vi "Position_TOTAL_R26.vi"(5 "Distance Between \nCameras  (*unit)":sgl=2.25) -> (12 "dX, dY\nLeft Cam":cluster{"X":sgl[], "Y":sgl[]}={"X"=[-1.0065897, 0.099401906, 1.1628555, 2.2500029, 0.0], "Y"=[10.716516, 10.801518, 10.883252, 10.9668045, 0.0]}, 13 "Position Valid":bool=TRUE, 14 "Left Camera Real Coordinates":cluster{"X":sgl, "Y":sgl}={"X"=10.842023, "Y"=1.3735824}, 16 "dX, dY\nRight Cam":cluster{"X":sgl[], "Y":sgl[]}={"X"=[-2.8840373, -1.7780458, -0.7145921, 0.3725553, -1.8774476], "Y"=[9.387911, 9.472914, 9.554648, 9.638201, -1.3286046]}, 18 "Robot Coordinates":cluster{"X":sgl, "Y":sgl}={"X"=10.17772, "Y"=2.3123062}, 19 "Orietnation\n(current)":sgl=-30.94054 format="%#_13g")   [LabVIEW 2015]
uses:
  <vilib>/Analysis/NI_AALPro.lvlib
  <vilib>/myRIO/Instrument Drivers/Onboard IO/DIO/DIO.lvlib
  <vilib>/Instr/_visa.llb/VISA Configure Serial Port (Instr).vi
  <vilib>/Analysis/coordinate.llb/2D Cartesian Coordinate Rotation (Array).vi
panel:
  out "Current Template - Right":T1(ring)
  out "Current Template - Left":T1(ring)
  in  "Tab Control 2":T2(tab)
  out "Beacon Coordinates - Right Image":T3={"Beacon Position - X px"=[88.975365, 121.85722, 157.60713, 192.74931, 229.82234], "Beacon Position - Y px"=[106.21975, 102.49595, 103.61968, 103.22959, 103.920715]}
  out "Beacon Coordinates - Left Image":T3={"Beacon Position - X px"=[96.57839, 127.0317, 159.93825, 190.94315, 221.86247], "Beacon Position - Y px"=[111.67795, 107.306076, 106.92789, 105.73433, 104.09002]}
  in  "Image Width (px)":sgl=320.0
  in  "Image Height (px)":sgl=240.0
  in  "Cam AOV Horizontal (deg)":sgl=58.0
  in  "Cam AOV Vertical (deg)":sgl=45.0
  out "Angle to Pixel Ratios":T4={"Angle to Pixel\nRatio - Horizontal"=0.18125, "Angle to Pixel\nRatio - Vertical"=0.1875} {"Angle to Pixel\nRatio - Vertical" format="%#_13g"; "Angle to Pixel\nRatio - Horizontal" format="%#_13g"}
  in  "Num of Beacons (Total)":i8=5
  out "Left Data\nInput Flag\n- Internal":bool
  out "Right Data\nInput Flag\n- Internal":bool
  out "This Servo \nAngle - Left":sgl=52.96875
  in  "Valid Angles - L":bool[](array[boolean])=[TRUE, TRUE, TRUE, TRUE, TRUE]
  in  "Valid Angles -R":bool[](array[boolean])=[TRUE, TRUE, TRUE, TRUE, TRUE]
  in  "Beacon Angles - L":sgl[](array[numeric])=[64.19745, 58.642975, 52.682835, 47.05908, 41.446476]
  in  "Beacon Angles -R":sgl[](array[numeric])=[71.43643, 65.46979, 58.9926, 52.62266, 45.904842]
  out "This Servo \nAngle - Right":sgl=58.76953
  in  "Position Calc\nReady":bool=TRUE
  out "Array":sgl[](array[numeric])=[9.555056, 8.575206, 8.036942, 7.810829, 6.6351933]
  out "Array 2":sgl[](array[numeric])=[5.5039287, 6.210328, 7.1312, 8.266513, 8.73579]
  out "Array 3":sgl[](array[numeric])=[3.2039287, 3.9103284, 4.8311996, 5.9665127, 6.4357905]
  in  "stop":bool
  in  "Startup GP's - RIGHT":u16[](array[numeric])
  in  "Startup GP's - LEFT":u16[](array[numeric])
  in  "Servo Algorithm\nCycle Time(ms)":i32=25
  in  "Move Servo\nThreshold (deg)":sgl=2.0 format="%#_13g"
  in  "SERVO ENABLE":bool=TRUE
  in  "Max Write\nTx Attempts":u8=3
  in  "Max Read\nTx Attempts":u8=3
  in  "close comms":bool
  in  "Servo Comm\nLoop Time (ms)":i32=20
  out "dT - Comm Loop":u32=21
  in  "Left Servo\nID":string="\u0000"
  in  "Servo Comm\nWait Time - (ms)":i32
  in  "Right Servo\nID":string="\u0001"
  in  "Search Step Size\n(deg)":sgl=15.0 format="%#_13g"
  out "Last Orientation":sgl=-35.285717
  out "Last Position":cluster{"X":sgl, "Y":sgl}={"X"=10.147585, "Y"=2.64441}
  in  "Compliance Slope":u8=128
  in  "Search Step Size":u16=50
  in  "Mounting Offset - Left":sgl=-45.0
  in  "Minimum Delta \nServo Threshold":i16=3
  in  "Maximum Move \nServo Threshold":i16=300
  in  "Wait Tick Threshold":i32=10
  in  "Min Num Frames\nper Search":i32=3
  in  "Middle Beacon\nCoordinates":cluster{"X":sgl, "Y":sgl}={"X"=0.0, "Y"=2.5}
  in  "Max Recovery\nSearch Attempts":u16=3
  in  "Max Recovery Count\n(Recovery Search)":u16=20
  in  "Mounting Offset - Right":sgl=45.0
  in  "Tracking Timeout\nThreshold":i32=10
  in  "Timeout to \nEnable Reactive Predict":u16=5
  out "Beacon Scales - Right":sgl[](array[numeric])=[50.81787, 54.150085, 54.01553, 51.723366, 54.605507]
  out "Beacon Scales - Left":sgl[](array[numeric])=[46.59789, 48.180458, 47.842606, 46.504417, 45.297752]
  in  "Recovery Parallel\nSearch Offset":u16=50
  in  "Max # Pan Moves":u16=3
  in  "Current Angle\n - Right (internal)":sgl=58.76953
  in  "Current Angle\n - Left (internal)":sgl=52.96875
  in  "Servo Goal Position\n - Left":u16=232
  in  "Servo Goal Position\n - Right":u16=563
  out "Move Servo - R":bool
  out "Move Servo - L":bool
  out "Current L (10bit)":u16=232
  out "Servo Moving - L":bool
  out "Servo Moving - R":bool
  out "Current R (10bit)":u16=559
  out "deltaMoveServo\n- L":i16
  out "Move Respond - L":bool
  out "Move Respond - R":bool
  out "deltaMoveServo\n- R":i16
  out "Current Main State - Left":T5(ring)=enum."Tracking"
  in  "Initial Main State - Left":T5(ring)
  in  "Image Lock - Left":bool=TRUE
  in  "Track Angle Valid - Left":bool=TRUE
  out "New Data  Flag\nLeft Servo":bool
  in  "Tracking Angle - Left":sgl=52.933372
  in  "Search Direction - in - L":bool
  out "Frames Processed\nCount - in -L":i32
  out "Recovery Mode Count - in Left":u16
  in  "Image Lock - Right":bool
  out "Recovery Search\nmove Count - in - L":u16
  out "Recovery Search\nAttempt Count - in - L":u16
  out "Current Move Delta - L":u16
  out "Next Main State - Left":T5(ring)=enum."Tracking"
  in  "Recovery Search\nDirection - L":bool=TRUE
  out "Last Track Angle - L":sgl=52.96875
  in  "Initial Main State- Right":T5(ring)
  out "Current Main State - Right":T5(ring)=enum."Tracking"
  in  "Track Angle Valid  - Right":bool
  out "New Data  Flag\nRight Servo":bool
  in  "Tracking Angle - Right":sgl=58.953144
  out "Recovery Search\nAttempt Count - Right":u16
  out "Recovery Search\nmove Count - Right":u16
  out "Frames Processed\nCount - in Right":i32
  out "Recovery Mode Count in Right":i32
  in  "Recovery Search\nDirection - R":bool
  out "Next Main State - Right":T5(ring)=enum."Tracking"
  in  "Search Direction - in - Right":bool=TRUE
  out "Tracking Timeout\nCount - L":i32
  out "Tracking Timeout\nCount - R":i32
  out "Current Tracking State - Left":enum16{"Track", "Reactive Predict", ""}(ring)
  in  "Initial Tracking State - Left":enum16{"Track", "Reactive Predict", ""}(ring)
  out "Next Tracking State - Left":enum16{"Track", "Reactive Predict", ""}(ring)
  in  "Initial Tracking State - Right":enum16{"Track", "Reactive Predict", ""}(ring)
  out "Current Tracking State - Right 2":enum16{"Track", "Reactive Predict", ""}(ring)
  out "Next Tracking State - Right":enum16{"Track", "Reactive Predict", ""}(ring)
  in  "Initial Recovery State - L":enum16{"Generic Sweep", "Recovery Search"}(ring)=enum."Recovery Search"
  in  "Initial Recovery State  - Right":enum16{"Generic Sweep", "Recovery Search"}(ring)=enum."Recovery Search"
  out "Current Recovery State - Right":enum16{"Generic Sweep", "Recovery Search"}(ring)=enum."Recovery Search"
  out "Next Recovery State - Right":enum16{"Generic Sweep", "Recovery Search"}(ring)=enum."Recovery Search"
  out "Next Recovery State - Left":enum16{"Generic Sweep", "Recovery Search"}(ring)=enum."Recovery Search"
  out "Current Recovery State -L":enum16{"Generic Sweep", "Recovery Search"}(ring)=enum."Recovery Search"
  out "Current Move Delta - R":u16
  in  "Mining Alignment\nEnabled":bool
  in  "Real Beacon\n - Coordinates":cluster{"X":dbl[], "Y":dbl[]}={"X"=[0.0, 0.0, 0.0, 0.0, 0.0, 0.0], "Y"=[0.5, 1.5, 2.5, 3.5, 4.5, 0.0]}
  out "LOCAL\nBeacon Coordinates\nRelative to Robot":cluster{"dX_beacon":sgl[], "dY_beacon":sgl[]}={"dX_beacon"=[5.5039287, 6.210328, 7.1312, 8.266513, 8.73579], "dY_beacon"=[9.555056, 8.575206, 8.036942, 7.810829, 6.6351933]}
  out "Local Coordinates - Calculated":cluster{sgl[], sgl[]}(graph)={[5.5039287, 6.210328, 7.1312, 8.266513, 8.73579], [9.555056, 8.575206, 8.036942, 7.810829, 6.6351933]}
  out "Distance to LBF":sgl[](array[numeric])=[0.024284193, 0.015691843, 0.008273765, 0.028971607, 0.03291407]
  out "Right Camera Real Coordinate":cluster{"X":sgl, "Y":sgl}={"X"=9.513418, "Y"=3.25103}
  out "Post Filtering\n- Valid Beacons":bool[](array[boolean])=[TRUE, TRUE, TRUE, TRUE, FALSE]
  in  "Distance\nBetween Beacons":sgl=1.0 format="%#_13g"
  in  "Distance\nBetween Beacons \n- Tolerance":sgl=0.5 format="%#_13g"
  in  "Distance Threshold\nRef Triangles (*unit)":sgl=30.0
  out "All Object Coordinates \n- Local":cluster{"X":sgl[], "Y":sgl[]}={"X"=[2.3, 5.368779, 6.320682, 7.235974, 8.171657, 0.0], "Y"=[0.0, 9.329155, 8.759661, 8.21207, 7.6522775, 0.0]}
  out "Local Coordinates - Normalized":cluster{sgl[], dbl[]}(graph)={[2.3, 5.368779, 6.320682, 7.235974, 8.171657, 0.0], [0.0, 9.329154968261719, 8.759660720825195, 8.21207046508789, 7.65227746963501, 0.0]}
  out "All Object Coordinates \n- Local - Rotated":cluster{"X":sgl[], "Y":sgl[]}={"X"=[1.8774476, -1.0065897, 0.099401906, 1.1628555, 2.2500029, 0.0], "Y"=[1.3286046, 10.716516, 10.801518, 10.883252, 10.9668045, 0.0]}
  out "Local Coordinates - Rotated":cluster{dbl[], dbl[]}(graph)={[1.8774476489648846, -1.0065896210507148, 0.09940190570174412, 1.1628555490135675, 2.250002943734801, 0.0], [1.3286045709883498, 10.716515276262749, 10.801518262128845, 10.883252530212562, 10.966804865321656, 0.0]}
  out "Right_Flag 2":bool
  out "Beacons Found\n- Right (Bool Array)":bool[](array[boolean])=[TRUE, TRUE, TRUE, TRUE, TRUE]
  out "RIGHT Beacon Position - Y px (IN)":sgl[](array[numeric])=[106.21975, 102.49595, 103.61968, 103.22959, 103.920715]
  out "RIGHT Beacon Coord - X px (IN)":sgl[](array[numeric])=[88.975365, 121.85722, 157.60713, 192.74931, 229.82234]
  out "Left_Flag 2":bool
  out "Beacons Found\n- Left (Bool Array) 2":bool[](array[boolean])=[TRUE, TRUE, TRUE, TRUE, TRUE]
  out "LEFT Beacon Coord - X px (IN) 2":sgl[](array[numeric])=[96.57839, 127.0317, 159.93825, 190.94315, 221.86247]
  out "LEFT Beacon Position - Y px (IN) 2":sgl[](array[numeric])=[111.67795, 107.306076, 106.92789, 105.73433, 104.09002]
  in  "Fetch Input\n(mSec)":u32=20 caption="Update Camera Input\n(mSec)"
  in  "Max Std Dev (5)":sgl=0.1 format="%#_13g"
  out "Position \nLock Status":bool=TRUE
  out "Real Position in Course 2":cluster{"X":dbl[], "Y":dbl[]}(graph)={"X"=[10.147584990557128], "Y"=[2.644409845240164]}
  out "Robot Coordinates - Avgd":cluster{"X":sgl, "Y":sgl}={"X"=10.147585, "Y"=2.64441}
  in  "Max Std Dev (4)":sgl=0.1 format="%#_13g"
  in  "Max Std Dev (3)":sgl=0.2 format="%#_13g"
  in  "New Position\nWeight (X coord)":sgl=0.8 format="%#_13g"
  in  "Max X (arena)":sgl=35.0
  in  "Max Y (arena)":sgl=15.0
  in  "History Size":u8=15
  out "Orientation Avgd":sgl=-35.285717
  in  "New Position \nThreshold":sgl=2.0
  out "Robot Coordinates\nHistory":cluster{sgl, sgl}[](array[cluster])=[{10.147585, 2.64441}, {10.056327, 2.8351064}, {10.020484, 2.7815769}, {10.034186, 2.7172103}, {0.0, 0.0}, {10.036168, 2.7859242}, {9.938812, 2.8961887}, {10.1160965, 2.6632404}, {10.016709, 2.7454932}, {10.037537, 2.8544023}, {10.017025, 2.7817721}, {9.997087, 2.8064857}, {10.065648, 2.6537364}, {10.084976, 2.6750228}, {10.082739, 2.688601}]
  out "Orientation\nHistory":sgl[](array[numeric])=[-35.285717, -36.86449, -36.153664, -35.44657, 0.0, -37.6105, -36.02637, -35.82032, -36.08894, -37.01076, -36.293255, -36.40525, -35.738438, -35.683483, -35.770218]
  out "Position Valid\nHistory":bool[](array[boolean])=[TRUE, TRUE, TRUE, TRUE, FALSE, TRUE, TRUE, TRUE, TRUE, TRUE, TRUE, TRUE, TRUE, TRUE, TRUE]
  in  "Moving Average\nWindow Length":u8=10
  in  "New Orientation \nThreshold":sgl=10.0
  in  "Triangle Based\nWeight":sgl format="%#_13g"
  out "Scale Based\nWeight":sgl=1.0 format="%#_13g"
  out "New Position\nWeight (Y coord)":sgl=0.3 format="%#_13g"
  out "New Orientation\nWeight":sgl=0.2
  out "dT":dbl=144.111
  in  "Position Calc\nTimer":u32=100 caption="Position Calc Timer"
  out "inches":dbl
  out "dA2 3":sgl=44.126 format="%#_13g"
  out "Valid Beacon Sets_":bool[](array[boolean])=[TRUE, TRUE, TRUE, TRUE, TRUE]
  in  "Check Shared Var Timer":u32=50 caption="Main Loop\n Timer (ms)"
  out "dA2 2":sgl=48.543114 format="%#_13g"
  out "dA2 4":sgl=48.543114 format="%#_13g"
  out "Last Track Angle - R":sgl=59.941406
  in  "Recovery Search\nDirection - L 2":bool
  in  "Max Recovery Count\n(Recovery Search) 2":u16
  in  "Max Recovery\nSearch Attempts 2":u16
  in  "Image Lock - Right 2":bool
  # "SETTINGS"
  # "IMAGE TO ANGLE VARIABLES"
  # "INPUTS"
  # "OUTPUT VALUES"
  # "CONFIG"
  # "SERVO CONTROL VARIABLES"
  # "SERVO CONTROL VARIABLES"
  # "Servo"
  # "CONFIG"
  # "SHARED VARIABLE INPUTS"
  # "LOCAL VARIABLE INPUTS"
  # "INTERNRAL VARIABLES"
  # "MISC"
  # "SERVO IDs"
  # "CONTROL DELAYS"
  # "COMM LOOP DELAY"
  # "COMM PROTOCOL"
  # "Make function of distance^^"
  # "LEFT SERVO"
  # "RIGHT SERVO"
  # "Main State Machine"
  # "Recovery State Machine"
  # "Current Track Angle Inputs"
  # "Servo Status Inputs"
  # "Main State Machine Inputs"
  # "Recovery State Machine Inputs"
  # "Current Track Angle Inputs"
  # "Servo Status Inputs"
  # "Tracking State Machine Inputs"
  # "Tracking State Machine Inputs"
  # "POSITION CALCULATION VARIABLES"
  # "OUTPUT VALUES"
  # "CONFIG VALUES"
  # "FILTER CONFIG VALUES"
  # "FEEDBACK INPUT VALUES"
  # "INPUT VALUES"
  # "INTERMEDIATE VALUES"
  # "Use moving average for previous orientation thresholds"
  # "*********************"
  # "unfiltered"
  # "Inter Beacon Distance Filtering"
  # "NOTE: Must be 1 bigger than amount of beacons"
  # "NOTE: Must be 1 bigger than amount of beacons"
  # "VISION PROCESSEING INPUTS"
  # "update to coordinate outlier filtering R2"
  # "NEW FILTER VALS"
  # "MOVING AVERAGE\nVARIABLES"
  # "DISTANCE SOURCE WEIGHT"
  # "*****  I made this 0\n         bc it seems to be \n        more stable"
  # "Recovery State Machine Feedback"
  # "SEARCH ROUTINE VARIABLES"
types:
  T1 = enum16{"Range 1", "Range 2", "Range 3", "Range 0"}
  T2 = enum32{"image to angle ", "Empty", "servo control - Config", "left and right servo - Status", "Position Calc - Debug Data", "Position Calc - Debug Data 2", "Vision Processing INputs", "ROBOT POSITION", "Random"}
  T3 = cluster{"Beacon Position - X px":sgl[], "Beacon Position - Y px":sgl[]}
  T4 = cluster{"Angle to Pixel\nRatio - Horizontal":sgl, "Angle to Pixel\nRatio - Vertical":sgl}
  T5 = enum16{"Start Up Search", "Tracking", "Recovery Mode", ""}
  T6 = cluster{"Lock":bool, "Current Valid":bool, "Current Template":enum16{"Range 1", "Range 2", "Range 3", "Range 0"}, "Tracking Coordinates":cluster{"X":dbl, "Y":dbl}, "Setting Values":cluster{"Min Score":dbl, "Min Scale":dbl, "Max Scale":dbl, "Curve Parameters":cluster{"Min Length":i32, "Row Search Step":i32, "Col Search Step":i32}}}
  T7 = cluster{"Array of Double":dbl[], "Array of Double":dbl[]}
  T8 = enum16{"Sub - 2", "Sub - 3", "Sub - 4", "Normal - 5"}
  T9 = typedef "DIO.lvlib/DIO Reference.ctl" = cluster{"myRIO Reference":T10, "DIO Channels List":T14}
  T10 = typedef "myRIO Generic Hardware Reference.ctl" = cluster{"myRIO Model":T11, "myRIO Hardware Reference":T12}
  T11 = typedef "Hardware Version Enum.ctl" = enum16{"Unknown", "myRIO-1900", "myRIO-1950", "roboRIO"}
  T12 = typedef "myRIO v1.0 Reference.ctl" = cluster{"Generic FPGA Reference":T13, "Allow multiple opens":bool}
  T13 = typedef "Generic FPGA Reference.ctl" = refnum<k20>
  T14 = typedef "DIO Channels List.ctl" = T15[]
  T15 = typedef "DIO Channels Enum.ctl" = enum16{"Not Connected", "C/DIO0", "C/DIO1", "C/DIO2", "C/DIO3", "C/DIO4", "C/DIO5", "C/DIO6", "C/DIO7", "A/DIO0", "A/DIO1", "A/DIO2", "A/DIO3", "A/DIO4", "A/DIO5", "A/DIO6", "A/DIO7", "A/DIO8", "A/DIO9", "A/DIO10", "A/DIO11", "A/DIO12", "A/DIO13", "A/DIO14", "A/DIO15", "B/DIO0", "B/DIO1", "B/DIO2", "B/DIO3", "B/DIO4", "B/DIO5", "B/DIO6", "B/DIO7", "B/DIO8", "B/DIO9", "B/DIO10", "B/DIO11", "B/DIO12", "B/DIO13", "B/DIO14", "B/DIO15", "LED0", "LED1", "LED2", "LED3", "Button0", "DIO/DIO0", "DIO/DIO1", "DIO/DIO2", "DIO/DIO3", "DIO/DIO4", "DIO/DIO5", "DIO/DIO6", "DIO/DIO7", "DIO/DIO8", "DIO/DIO9", "SPI/CS0", "SPI/CS1", "SPI/CS2", "SPI/CS3", "LED RADIO (Green)", "LED RADIO (Red)", "LED COMM (Green)", "LED COMM (Red)", "LED MODE (Green)", "LED MODE (Red)"}
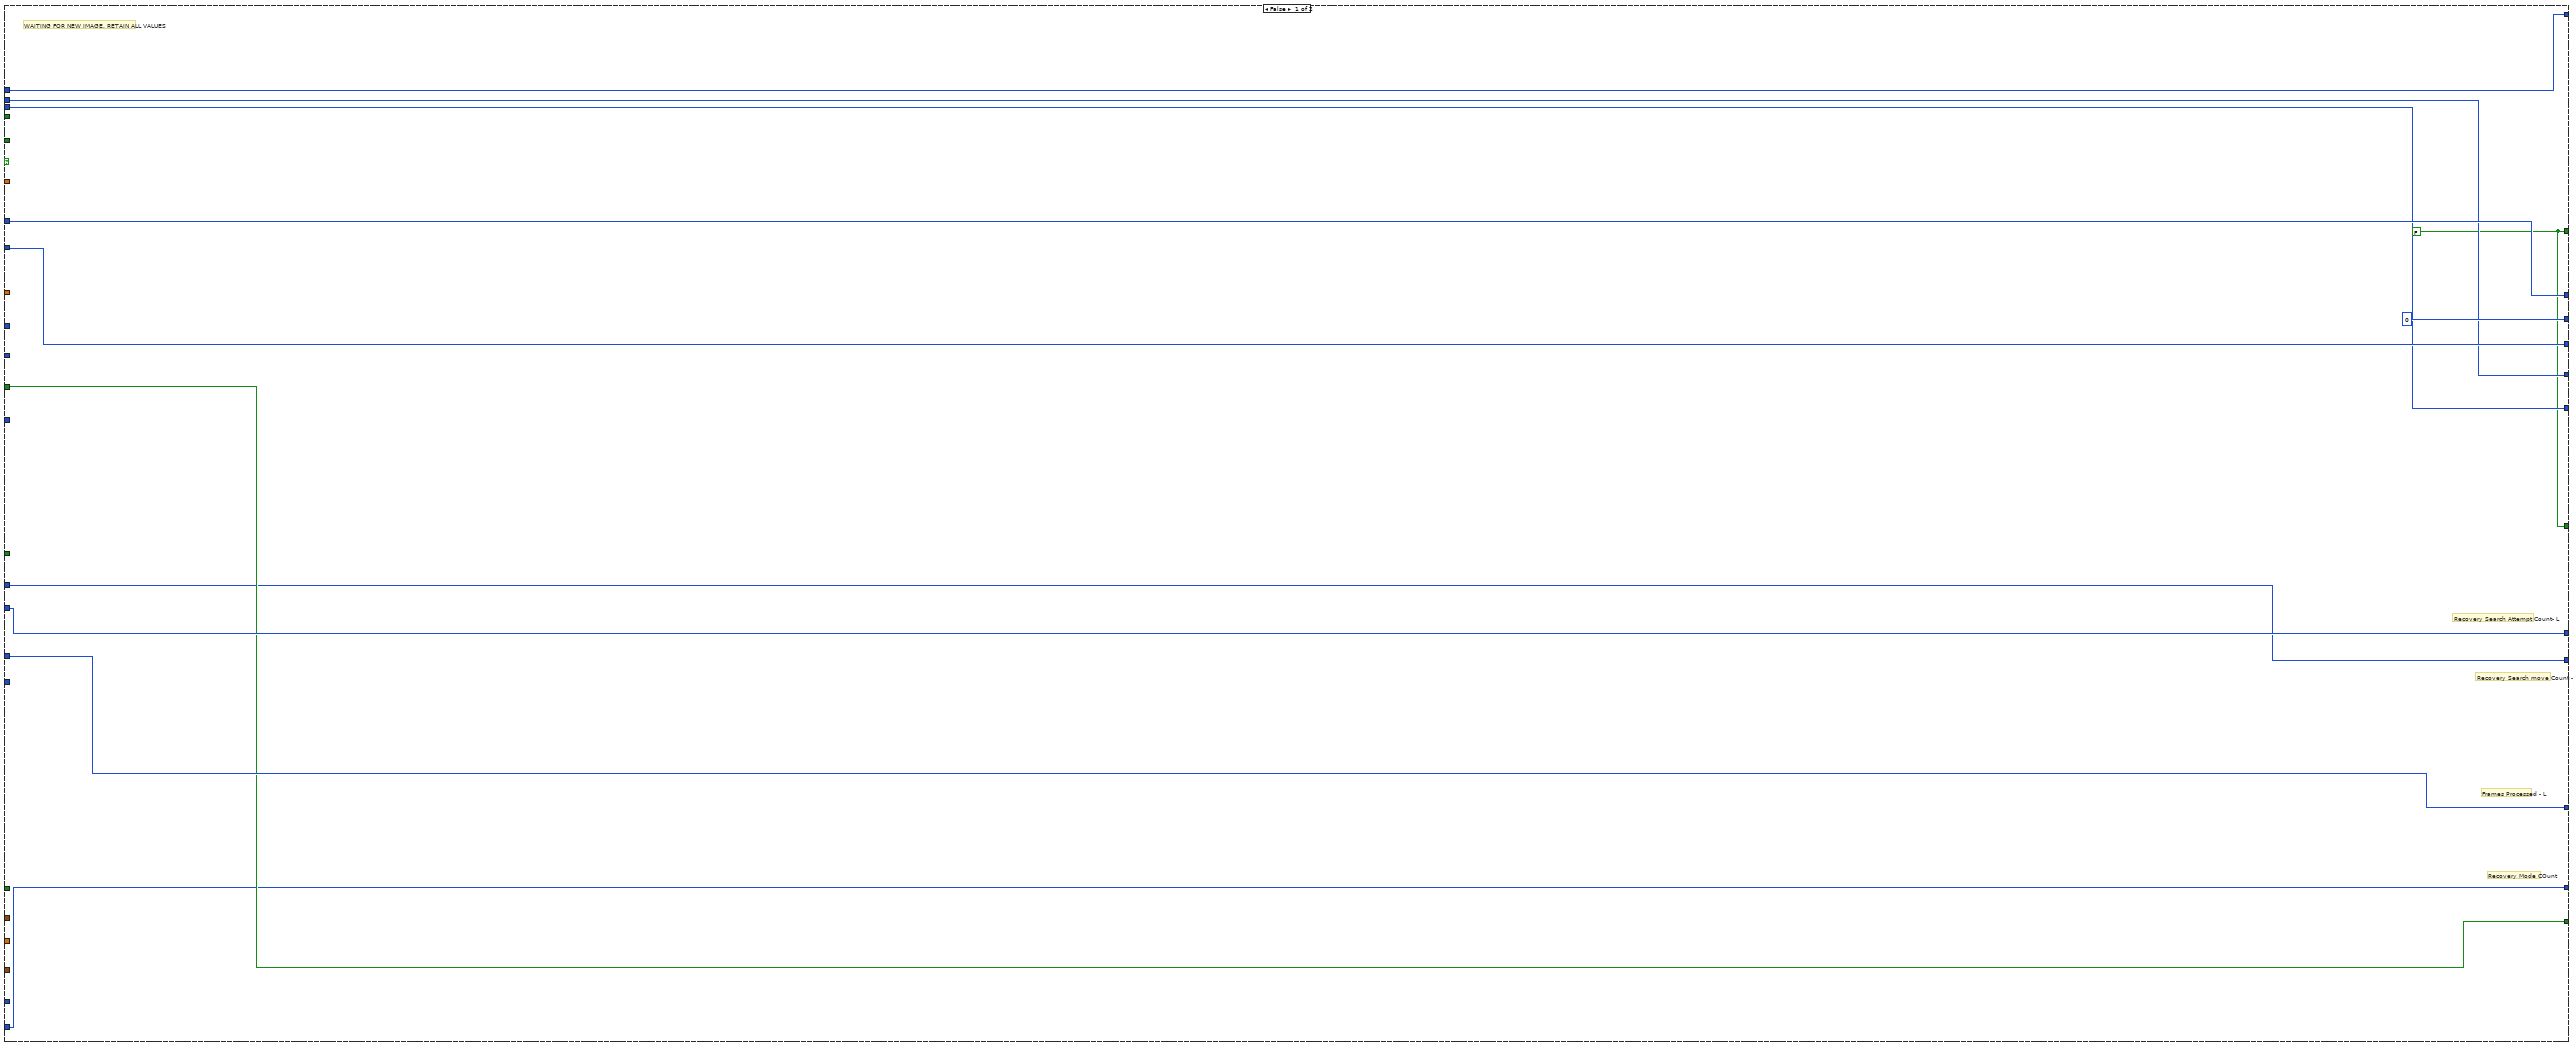
[diagram p2: hidden frame]
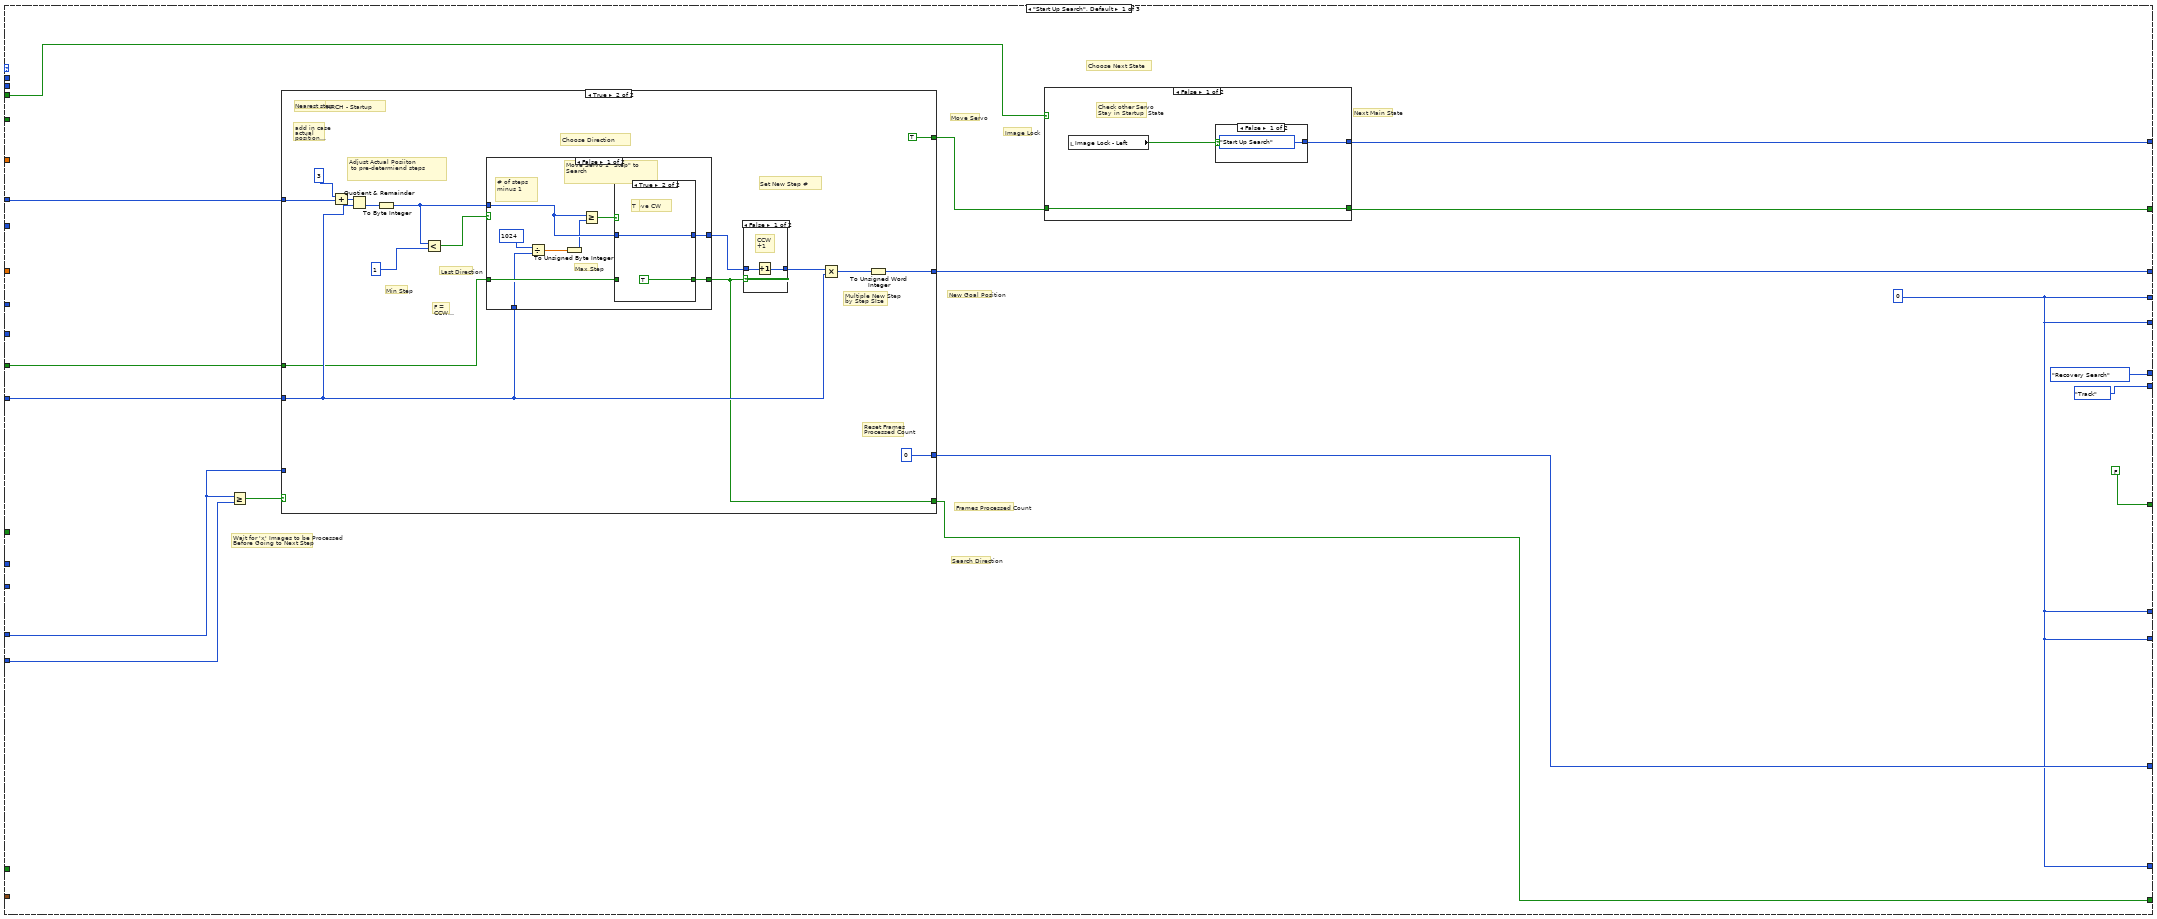
[diagram p3: hidden frame]
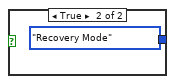
[diagram p4: hidden frame]
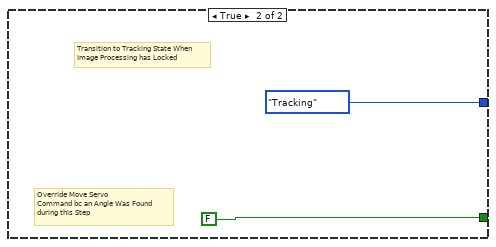
[diagram p5: hidden frame]
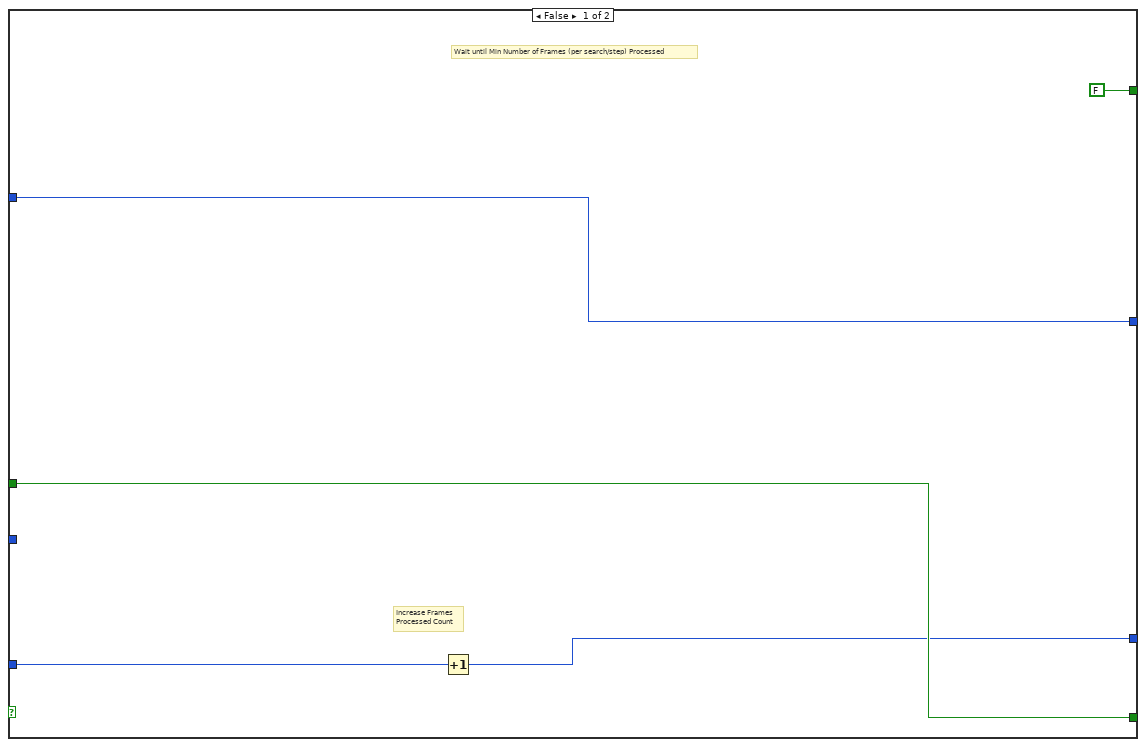
[diagram p6: hidden frame]
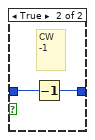
[diagram p7: hidden frame]
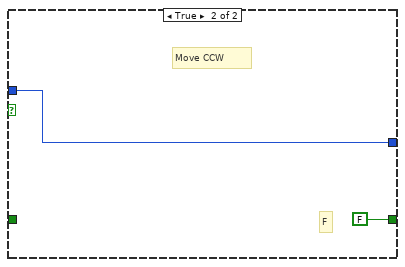
[diagram p9: hidden frame]
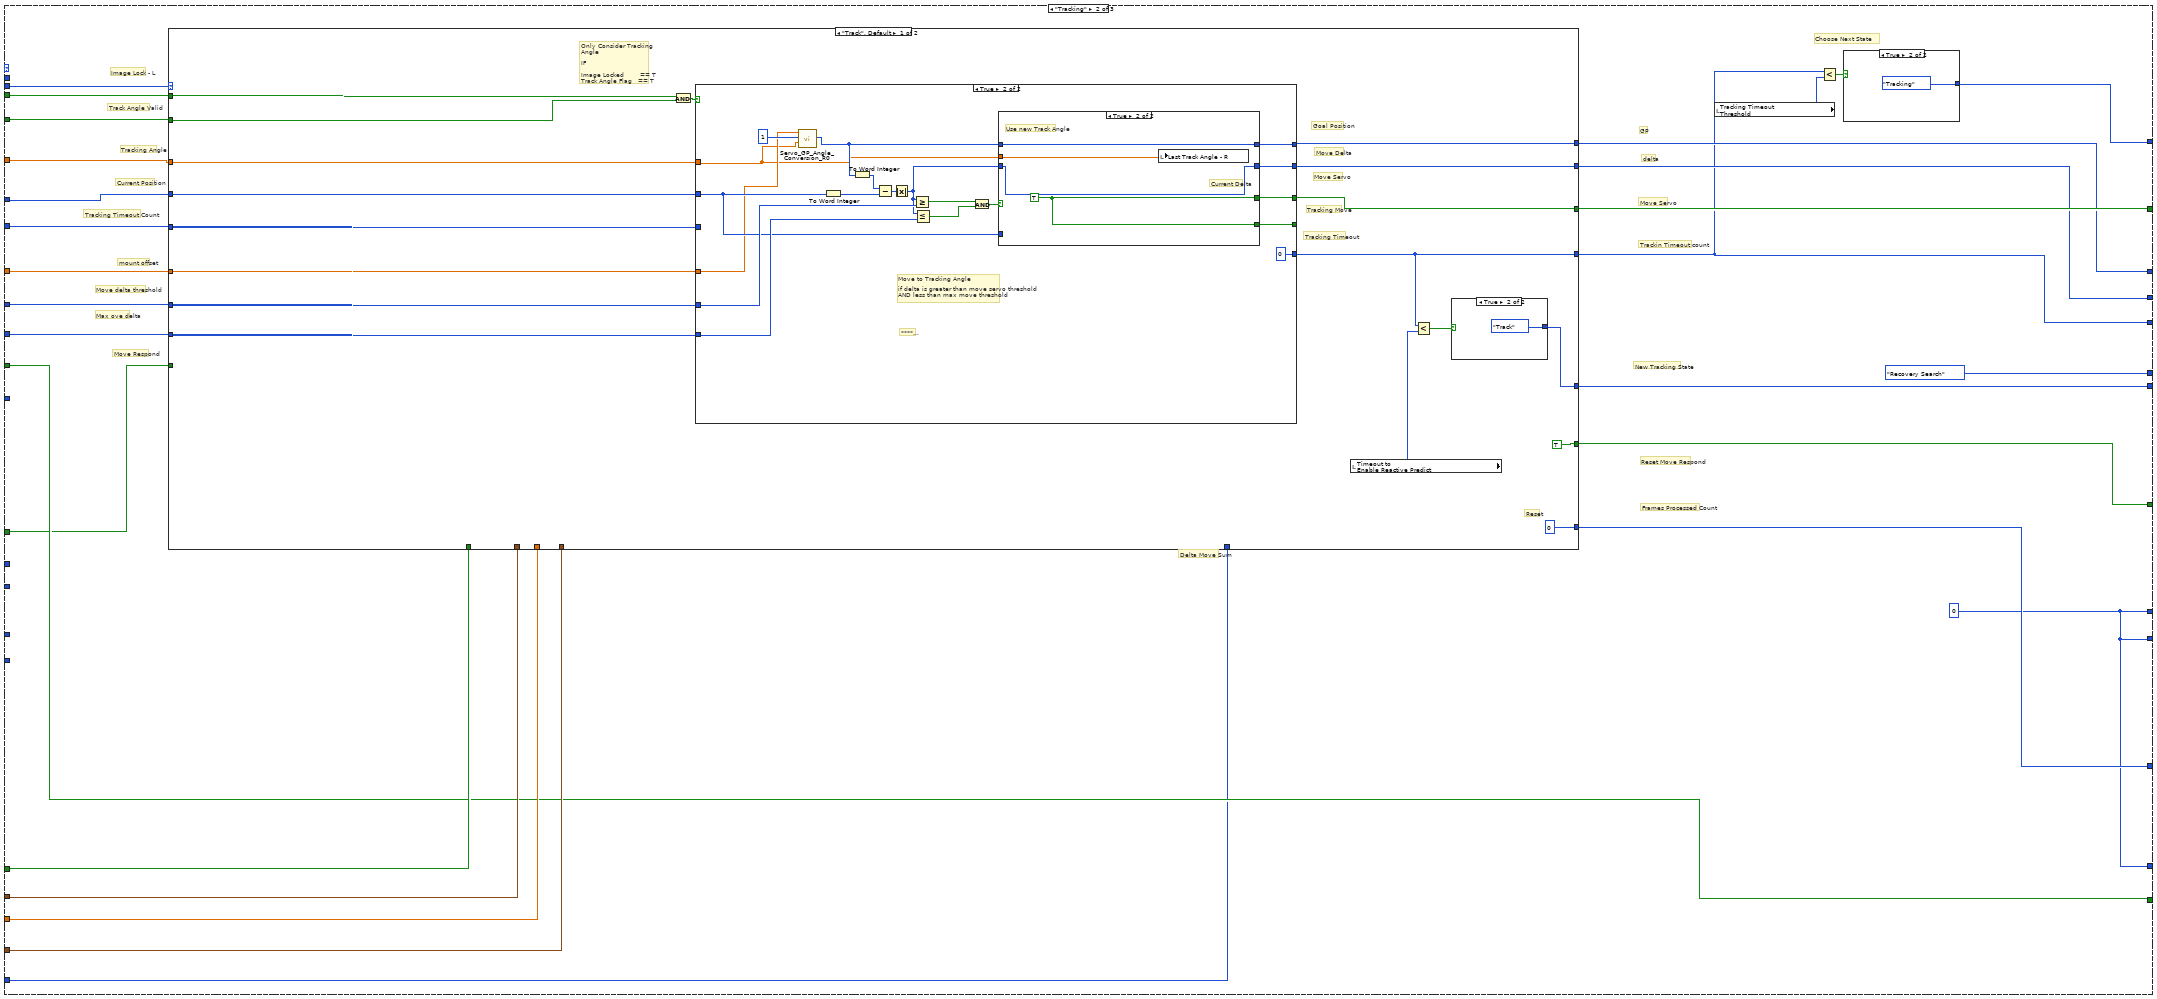
[diagram p10: hidden frame]
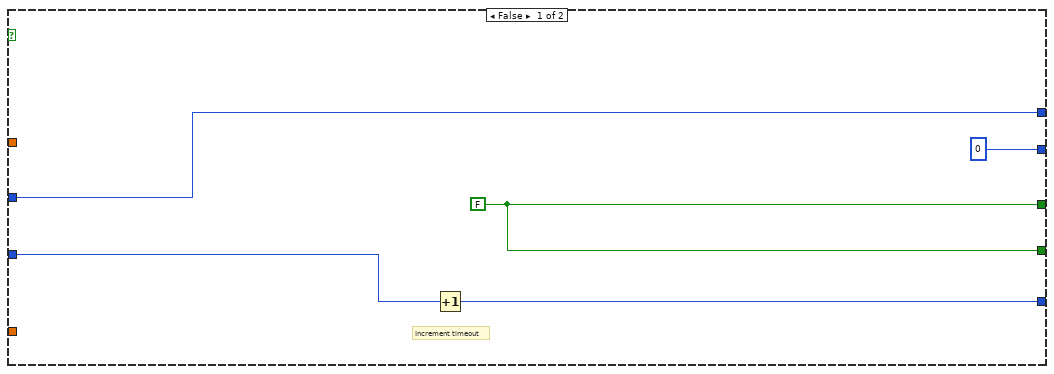
[diagram p11: hidden frame]
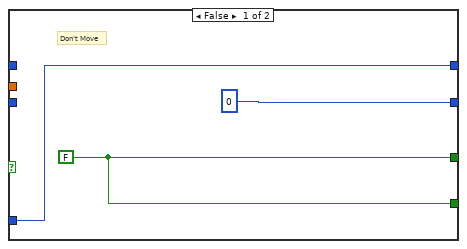
[diagram p12: hidden frame]
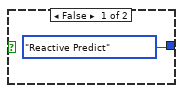
[diagram p13: hidden frame]
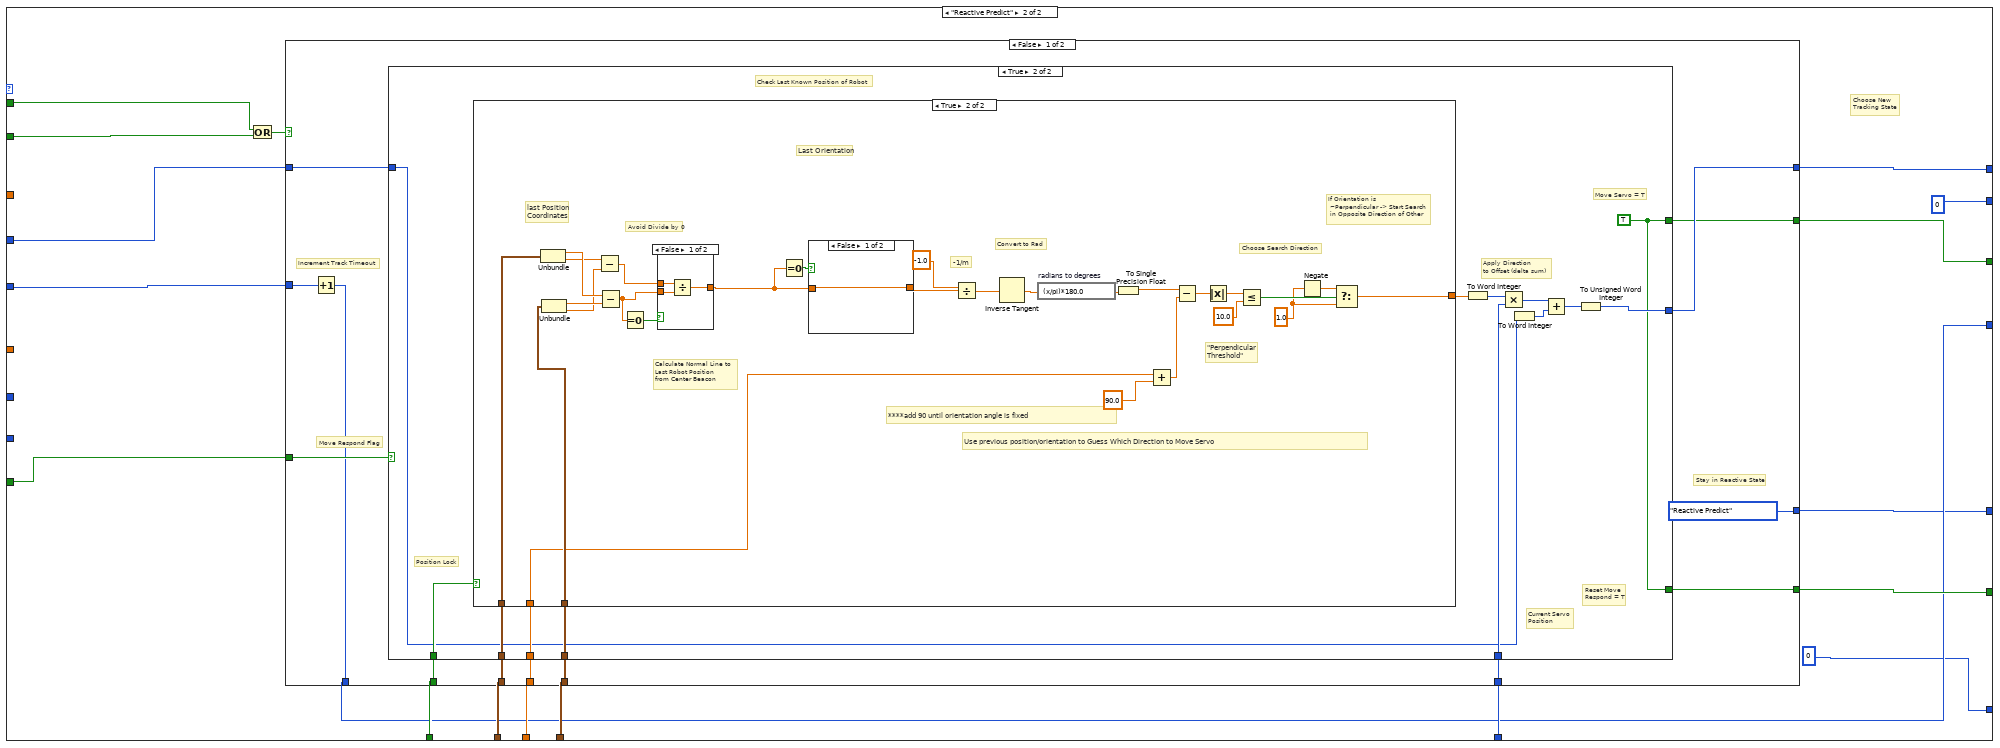
[diagram p14: hidden frame]
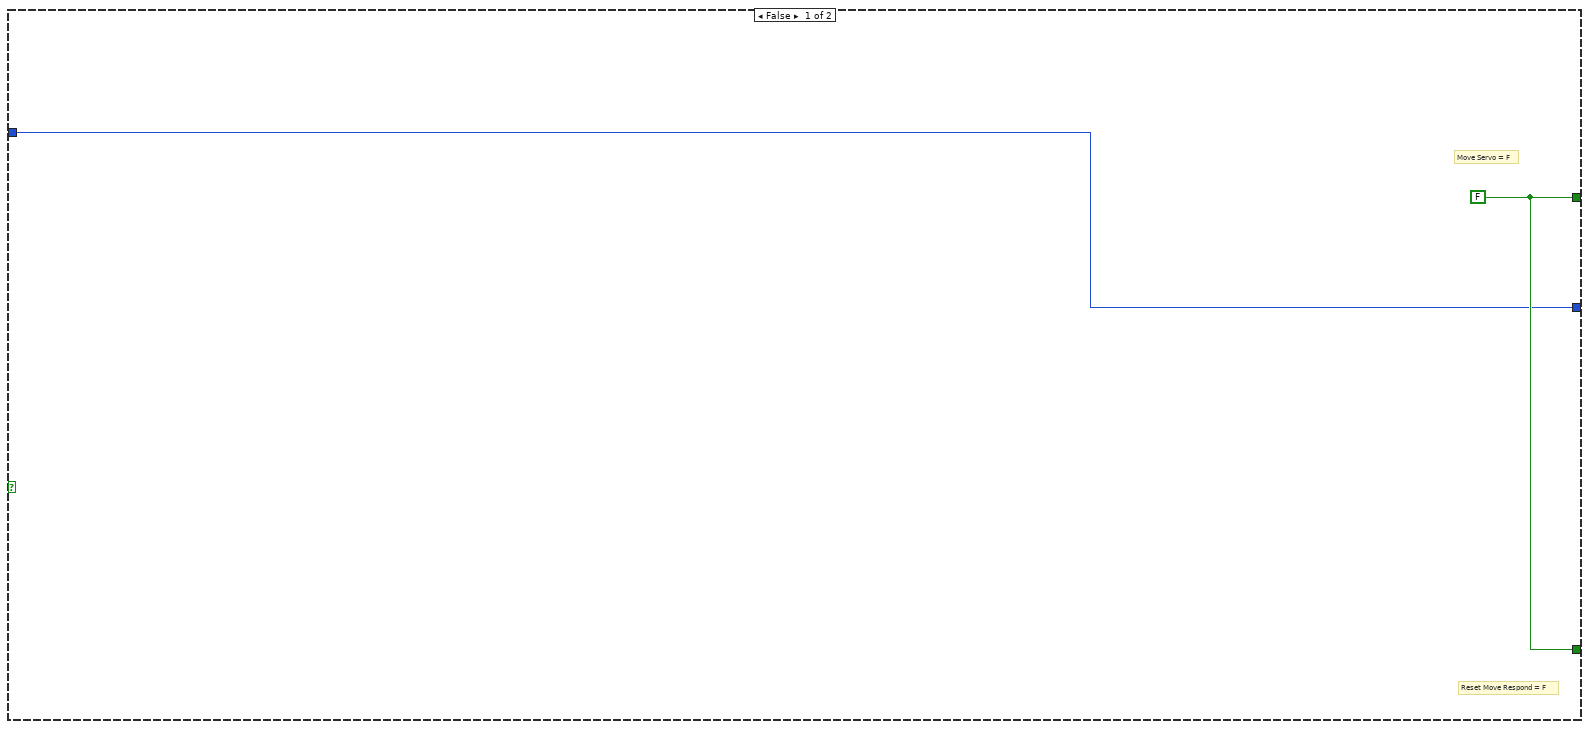
[diagram p15: hidden frame]
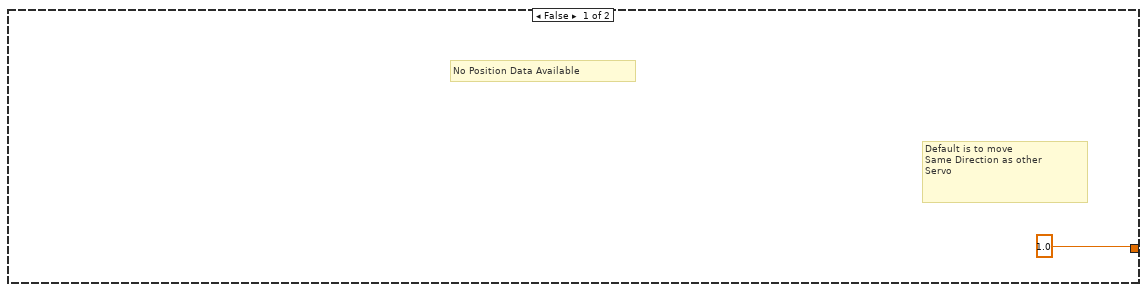
[diagram p16: hidden frame]
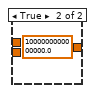
[diagram p17: hidden frame]
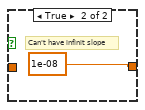
[diagram p18: hidden frame]
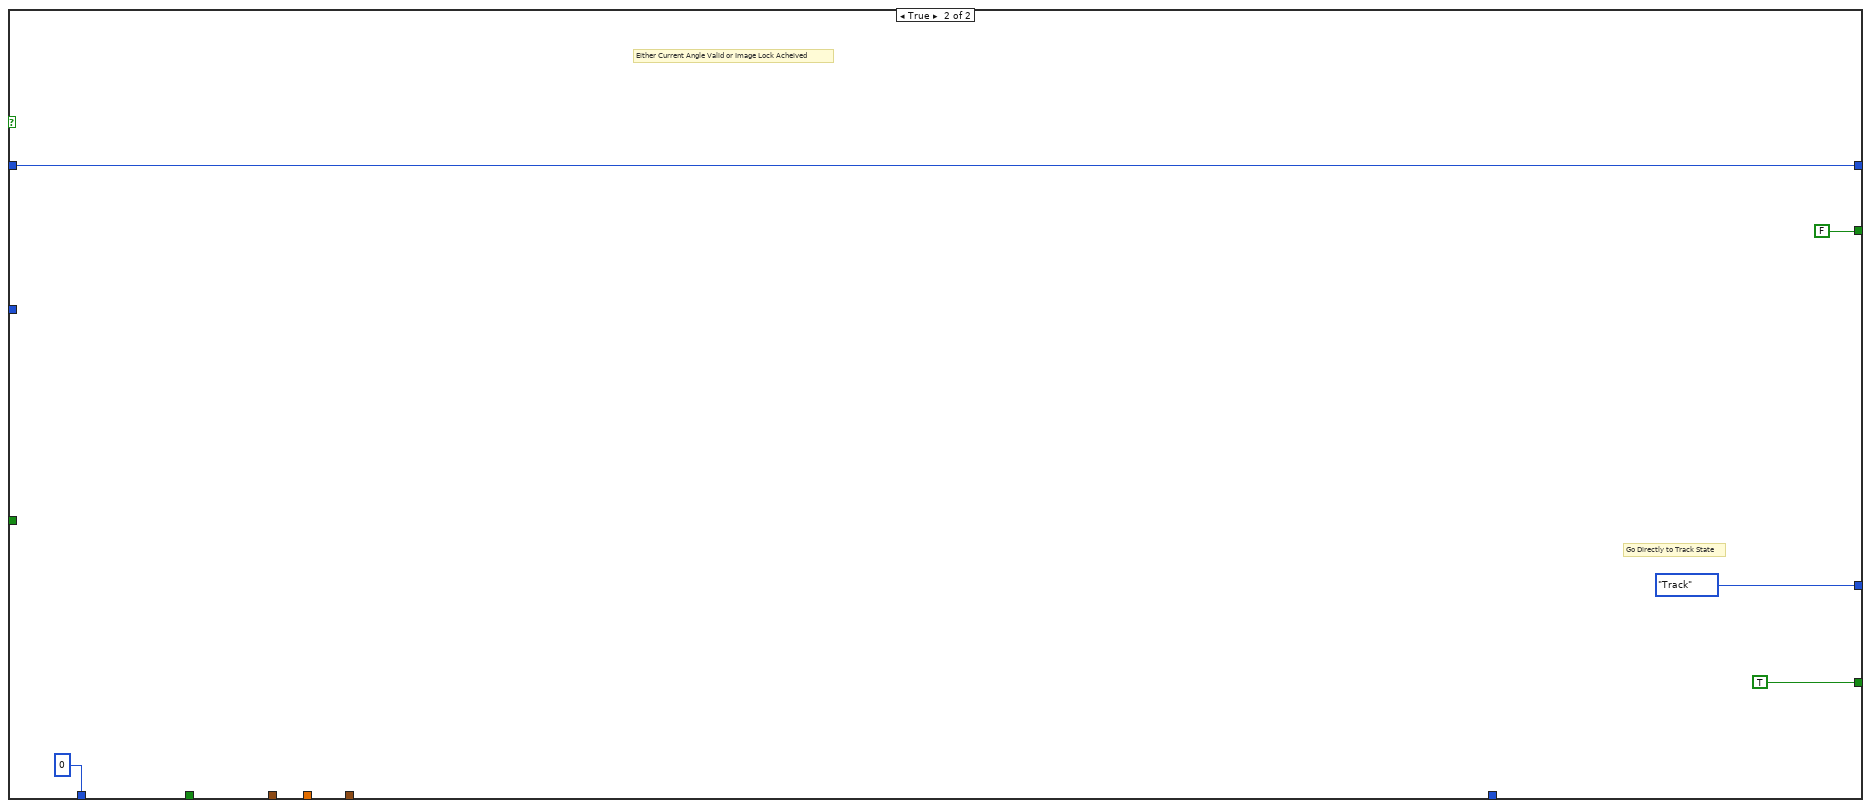
[diagram p19: hidden frame]
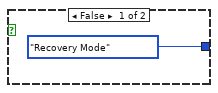
[diagram p20: hidden frame]
diagram:
  (unwired) enum16{"Generic Sweep", "Recovery Search"}."Recovery Search"
  w12 = 0 ("Frames Processed\nCount - in")
  w13 = 0 ("Frames Processed\nCount - in")
  w2 = FALSE
  w34 = sgl 0.0
  # "SERVO CONTROL FLAGS"
  # "***"
  # "Next Tracking State"
  # "Tracking Timeout Count"
  # "Search Direction - L"
  # "Next Recovery State"
  # "Move Respond"
  # "Recovery Mode Count - L"
  # "Delta Move Sum - L"
  # "Wait Tick Count - L"
  # "Frames Processed - L"
  # "Recovery Search move Count - L"
  # "Recovery Search Attempt Count- L"
  # "Next Main State"
  # "Search Direction - L"
  # "Next Recovery State"
  # "INPUTS - Local vars"
  # "Recovery Mode Count - L"
  # "Delta Move Sum - L"
  # "Frames Processed\nLeft"
  # "Move Respond - R"
  # "Initial Search Direction\n- Right"
  # "Move Respond"
  # "Recovery Mode Count - L"
  # "Delta Move Sum - L"
  # "Wait Tick Count - L"
  # "Frames Processed - L"
  # "Recovery Search move Count - L"
  # "Recovery Search Attempt Count- L"
  # "Next Main State"
  # "Settings -- Update in a slow loop"
  # "Recovery Mode Count - L"
  # "Delta Move Sum - L"
  # "Frames Processed\nLeft"
  # "Move Respond - L"
  # "Replace these with\nconstants"
  # "Initial Search Direction\n- Left"
  # "Read Inputs when Available"
  # "# of Physical Beacons"
  # "Right Data Internal Falg"
  # "Left Data Internal Falg"
  # "Initialize Shift Arrays"
  # "Robot Position (cluster)\nShift Array"
  # "Robot Position (cluster)\nShift Array"
  # "Position Valid Shift Array"
  # "Orientation Shift Array"
  # "Position Valid Shift Array"
  # "Orientation Shift Array"
  # "Servo Communication (to Servo- UART))"
  # "Internal Local Variables"
  # "Servo Control Logic"
  # "Local Variables"
  # "Images to Robot Position Calculation Process"
  # "SERVO MOTOR CONTROL"
  # "SERVO MOTOR CONTROL"
  n1 = Divide(x="Cam AOV Horizontal (deg)", y="Image Width (px)") -> (x/y=w25:sgl)
  n2 = Divide(x="Cam AOV Vertical (deg)", y="Image Height (px)") -> (x/y=w26:sgl)
  n3 = Bundle(w25, w26) -> (w20:cluster{sgl, sgl})  [unwired: 1 in]
  "Angle to Pixel Ratios" <- w20
  n4 = disable-structure shown="Disabled" {
    frame Disabled {
      # "Always Read Incoming Flags & Store"
      n5 = while {
        tunnel: "Check Shared Var Timer" -> [w46]
        stop <- FALSE stop-if-true
        n6 = shared-variable "myRIO-1900\\Lib1.lvlib\\RIGHT_FLAG"() -> (→"Right_Flag 2":bool)  [unwired: 1 in, 1 out]
        n7 = shared-variable "myRIO-1900\\Lib1.lvlib\\Left_Flag"() -> (→"Left_Flag 2":bool)  [unwired: 1 in, 1 out]
        n8 = call "Wait8"("Count(mSec)"=w46) -> ()  [unwired: 1 out]
      }
    }
    frame Enabled {
    }
  }
  n9 = while {
    shift-right: [w55] -> _
    shift-left: w2 -> [w60]
    shift-right: [w54] -> _
    shift-left: w2 -> [w58]
    tunnel: w20 -> [w56]
    tunnel: "Num of Beacons (Total)" -> [w57]
    stop <- FALSE stop-if-true
    # "Wait for Both Internal Flags"
    n10 = call "Wait6"("Count(mSec)"="Fetch Input\n(mSec)") -> ()  [unwired: 1 out]
    n11 = shared-variable "RT myRIO Target - Overlord\\Localization_Variables_r0.lvlib\\RIGHT_FLAG"() -> (w51:bool)  [unwired: 1 in, 1 out]
    n12 = shared-variable "RT myRIO Target - Overlord\\Localization_Variables_r0.lvlib\\Left_Flag"() -> (w52:bool)  [unwired: 1 in, 1 out]
    n13 = case shown="True" w51 {
      tunnel: w57 -> [_ w79]
      tunnel: w56 -> [_ w77]
      tunnel: [w61 w67] -> w49
      tunnel: w58 -> [w61 _]
      frame False {
        # "Don't Update Servo Position\nbc we're waiting on new Data to\ncome in and the servo position\nwas set at the previous set of data"
      }
      frame True {
        w67 = TRUE
        # "Store Values"
        # "Raise Internal Flag"
        # "If New Data Available"
        # "From Shift Reg"
        # "Perforrm Indivudual Angle Calculation"
        # "Pull Down Individual Flag"
        n14 = shared-variable "RT myRIO Target - Overlord\\Localization_Variables_r0.lvlib\\RIGHT_BEACON_X_array"() -> (w73:dbl[])  [unwired: 1 in, 1 out]
        "RIGHT Beacon Coord - X px (IN)" <- w73
        n15 = shared-variable "RT myRIO Target - Overlord\\Localization_Variables_r0.lvlib\\Image Lock - R"() -> (w68:bool)  [unwired: 1 in, 1 out]
        n16 = shared-variable "RT myRIO Target - Overlord\\Localization_Variables_r0.lvlib\\RIGHT_BEACON_Scales"() -> (→"Beacon Scales - Right":sgl[])  [unwired: 1 in, 1 out]
        n17 = shared-variable "RT myRIO Target - Overlord\\Localization_Variables_r0.lvlib\\Info - Right"() -> (w65:T6)  [unwired: 1 in, 1 out]
        n18 = shared-variable "RT myRIO Target - Overlord\\Localization_Variables_r0.lvlib\\RIGHT_BEACON_Y_array"() -> (w72:dbl[])  [unwired: 1 in, 1 out]
        "RIGHT Beacon Position - Y px (IN)" <- w72
        n19 = shared-variable "RT myRIO Target - Overlord\\Localization_Variables_r0.lvlib\\RIGHT_BEACON_BOOL_array"() -> (w71:bool[])  [unwired: 1 in, 1 out]
        "Beacons Found\n- Right (Bool Array)" <- w71
        n20 = Unbundle By Name(w65) -> ("Tracking Coordinates"=w64:cluster{"X":dbl, "Y":dbl}, "Current Valid"=w63:bool, "Current Template"=→"Current Template - Right":T1)
        n21 = local write "Image Lock - Right"(w68) -> ()
        n22 = Bundle("Array of Double"=w73, "Array of Double"=w72) -> (w70:T7)  [unwired: 1 in]
        "Beacon Coordinates - Right Image" <- w70
        n23 = shared-variable "RT myRIO Target - Overlord\\Localization_Variables_r0.lvlib\\Right Servo Angle_Image"() -> (w69:dbl)  [unwired: 1 in, 1 out]
        "This Servo \nAngle - Right" <- w69
        n24 = shared-variable "RT myRIO Target - Overlord\\Localization_Variables_r0.lvlib\\RIGHT_FLAG"(FALSE) -> ()  [unwired: 1 in, 1 out]
        n25 = feedback #1() -> (w81:sgl[])  [unwired: 1 in]
        n26 = feedback #2() -> (w80:bool[])  [unwired: 1 in]
        n27 = call "Angle Calc_Individual Process R4.vi"("Angle to Pixel Ratios"=w77, "Previous Angles"=w81, "Num of Beacons"=w79, "Beacon Coordinates - Image"=w70, "Current Servo Angle"=w69, "Beacons Found (Bool Array)"=w71, "Previous Valid Angles"=w80, "Tracking Coordinates"=w64) -> ("Servo Goal Angle"=w76:sgl, "Valid Beacons (Bool Array)\nPosition Calc"=w75:bool[], "Angle Of Beacons \nRelative to Robot"=w74:sgl[])  [unwired: 4 in, 1 out]
        n28 = feedback-in #1(w74) -> ()
        n29 = feedback-in #2(w75) -> ()
        n30 = local write "Tracking Angle - Right"(w76) -> ()
        n31 = local write "Beacon Angles -R"(w74) -> ()
        n32 = local write "Valid Angles -R"(w75) -> ()
        n33 = local write "Track Angle Valid  - Right"(w63) -> ()
        n34 = local write "New Data  Flag\nRight Servo"(w67) -> ()
      }
    }
    "Right Data\nInput Flag\n- Internal" <- w49
    n35 = case shown="True" w52 {
      tunnel: [w82 w88] -> w48
      tunnel: w60 -> [w82 _]
      tunnel: w56 -> [_ w92]
      tunnel: w57 -> [_ w91]
      frame False {
        # "Don't Update Servo Position\nbc we're waiting on new Data to\ncome in and the servo position\nwas set at the previous set of data"
      }
      frame True {
        w88 = TRUE
        # "Store Values"
        # "Raise Internal Flag"
        # "If New Data Available"
        # "Perforrm Indivudual Angle Calculation"
        # "Pull Down Individual Flag"
        n36 = shared-variable ".\\Localization_Variables_r0.lvlib\\LEFT_BEACON_X_array"() -> (w98:dbl[])  [unwired: 1 in, 1 out]
        "LEFT Beacon Coord - X px (IN) 2" <- w98
        n37 = shared-variable "RT myRIO Target - Overlord\\Localization_Variables_r0.lvlib\\LEFT_BEACON_Scales"() -> (→"Beacon Scales - Left":sgl[])  [unwired: 1 in, 1 out]
        n38 = shared-variable "RT myRIO Target - Overlord\\Localization_Variables_r0.lvlib\\LEFT_BEACON_Y_array"() -> (w99:dbl[])  [unwired: 1 in, 1 out]
        "LEFT Beacon Position - Y px (IN) 2" <- w99
        n39 = shared-variable "RT myRIO Target - Overlord\\Localization_Variables_r0.lvlib\\LEFT_BEACON_BOOL_array"() -> (w100:bool[])  [unwired: 1 in, 1 out]
        "Beacons Found\n- Left (Bool Array) 2" <- w100
        n40 = shared-variable "RT myRIO Target - Overlord\\Localization_Variables_r0.lvlib\\Image Lock - L"() -> (w89:bool)  [unwired: 1 in, 1 out]
        n41 = shared-variable "RT myRIO Target - Overlord\\Localization_Variables_r0.lvlib\\Info - Left"() -> (w86:T6)  [unwired: 1 in, 1 out]
        n42 = Unbundle By Name(w86) -> ("Tracking Coordinates"=w85:cluster{"X":dbl, "Y":dbl}, "Current Valid"=w84:bool, "Current Template"=→"Current Template - Left":T1)
        n43 = local write "Image Lock - Left"(w89) -> ()
        n44 = Bundle("Array of Double"=w98, "Array of Double"=w99) -> (w96:T7)  [unwired: 1 in]
        "Beacon Coordinates - Left Image" <- w96
        n45 = shared-variable "RT myRIO Target - Overlord\\Localization_Variables_r0.lvlib\\Left Servo Angle_Image"() -> (w90:dbl)  [unwired: 1 in, 1 out]
        "This Servo \nAngle - Left" <- w90
        n46 = shared-variable "RT myRIO Target - Overlord\\Localization_Variables_r0.lvlib\\Left_Flag"(FALSE) -> ()  [unwired: 1 in, 1 out]
        n47 = feedback #3() -> (w102:sgl[])  [unwired: 1 in]
        n48 = feedback #4() -> (w101:bool[])  [unwired: 1 in]
        n49 = call "Angle Calc_Individual Process R4.vi"("Angle to Pixel Ratios"=w92, "Previous Angles"=w102, "Num of Beacons"=w91, "Beacon Coordinates - Image"=w96, "Current Servo Angle"=w90, "Beacons Found (Bool Array)"=w100, "Previous Valid Angles"=w101, "Tracking Coordinates"=w85) -> ("Servo Goal Angle"=w95:sgl, "Valid Beacons (Bool Array)\nPosition Calc"=w94:bool[], "Angle Of Beacons \nRelative to Robot"=w93:sgl[])  [unwired: 4 in, 1 out]
        n50 = feedback-in #3(w93) -> ()
        n51 = feedback-in #4(w94) -> ()
        n52 = local write "Beacon Angles - L"(w93) -> ()
        n53 = local write "Valid Angles - L"(w94) -> ()
        n54 = local write "Tracking Angle - Left"(w95) -> ()
        n55 = local write "Track Angle Valid - Left"(w84) -> ()
        n56 = local write "New Data  Flag\nLeft Servo"(w88) -> ()
      }
    }
    "Left Data\nInput Flag\n- Internal" <- w48
    n57 = And(x=w48, y=w49) -> (x .and. y?=w59:bool)
    n58 = case shown="True" w59 {
      selector: w59 -> [_ w105]
      tunnel: w48 -> [w104 _]
      tunnel: [w104 w106] -> w55
      tunnel: [w103 w106] -> w54
      tunnel: w49 -> [w103 _]
      frame False {
      }
      frame True {
        w106 = FALSE
        # "Reset Internal Data Flags"
        # "Position Data\nReady Enabled"
        n59 = local write "Position Calc\nReady"(w105) -> ()
      }
    }
  }
  n60 = Bundle(w34, w34) -> (w37:cluster{sgl, sgl})  [unwired: 1 in]
  n61 = Initialize Array(w34, "History Size") -> (w32:sgl[])
  n62 = Initialize Array(w37, "History Size") -> (w33:cluster{sgl, sgl}[])
  n63 = Initialize Array(FALSE, "History Size") -> (w31:bool[])
  n64 = call "Tick Count4"() -> ("Tick Count(uSec)"=w30:u32)
  n65 = while {
    shift-right: [w117] -> _
    shift-left: w32 -> [w114]
    shift-right: [w116] -> _
    shift-left: w31 -> [w115]
    shift-right: [w118] -> _
    shift-left: w33 -> [w109]
    shift-right: [w110] -> _
    shift-left: w30 -> [w111]
    stop <- "stop" stop-if-true
    n66 = call "Wait5"("Count(mSec)"="Position Calc\nTimer") -> ()  [unwired: 1 out]
    n67 = case shown="True" "Position Calc\nReady" {
      selector: "Position Calc\nReady" -> [_ w209]
      tunnel: w109 -> [_ w227]
      tunnel: w109 -> [w127 w222]
      tunnel: w114 -> [w129 w221]
      tunnel: w115 -> [w128 w220]
      tunnel: [w129 w226] -> w117
      tunnel: [w128 w224] -> w116
      tunnel: [w127 w225] -> w118
      tunnel: w115 -> [_ w219]
      tunnel: w114 -> [_ w218]
      tunnel: [w126 w214] -> w112
      tunnel: w111 -> [_ w214]
      tunnel: [FALSE TRUE] -> w113
      tunnel: w109 -> [_ w211]
      frame False {
        n68 = call "Tick Count5"() -> ("Tick Count(uSec)"=w126:u32)
      }
      frame True {
        w147 = 0.0 ("y")
        # "***************************"
        # "dY"
        # "dX"
        # "Valid"
        # "Find Local Coordinates"
        # "Valid COunt"
        # "Make sure 2+ Data Sets are Still available"
        # "Check 1st element\nwith rest of elements"
        # "Make Sure all Pointed \nIn Same Direction"
        # "For Each Valid Beacon\nCalculate Distance from Each Camera to Each Beacon"
        # "Find Common Beacons\nAmong Cameras"
        # "Currently will only\ncalculate position if 2+ \nbeacons are available \nfrom both cameras"
        # "System is in Normal (long range) State"
        # "Average Both Data Sets"
        # "Estimate Distance for each Available Beacon Angle\nPER Camera, indivduallly"
        # "At least 2+ Avaialbe"
        # "CALCULATE AVERAGE ORIENTATION"
        # "Update Outputs\nif Current Calc is Invalid\n(shouldn't matter)"
        # "Estimate Orienation Based on Previous Position"
        # "****# of previous in history that must be true\nin order for position to be considered \"locked\""
        # "New Position is Valid if both \nOrientation and Positions\nis within range of previous"
        # "Robot Position\n Shift Array"
        # "Position Valid Shift Array"
        # "Orientation Shift Array"
        # "Orientation Value"
        # "Shift & Insert Current Position Valid"
        # "Position Valid\n(orientation)"
        # "Position Valid\n(position)"
        # "Update Shift Registers"
        # "Shift & Insert Current Calculated Orientation"
        # "Shift & Insert Current Robot Position"
        # "UPDATE FINAL OUTPUT\n VALUES"
        n69 = local read "Num of Beacons (Total)"() -> (w192:i8)
        n70 = Not(x=w209) -> (.not. x?=w210:bool)
        n71 = local write "Position Calc\nReady"(w210) -> ()
        n72 = disable-structure shown="Disabled" {
          frame Disabled {
            w274 = T8."Normal - 5" ("Initial State")
            # "***********do for both"
            # "sTATE"
            n73 = local read item#-1() -> (w278)
            n74 = local read item#-1() -> (w277)
            n75 = Equal?(x=w278, y=w274) -> (x = y?=w276:bool)
            n76 = Equal?(x=w277, y=w274) -> (x = y?=w275:bool)
            n77 = And(x=w276, y=w275) -> ()  [unwired: 1 out]
          }
          frame Enabled {
          }
        }
        n78 = local read "Current Template - Left"() -> (w151:T1)
        n79 = local read "Current Template - Right"() -> (w150:T1)
        n80 = local read "Beacon Scales - Left"() -> (w198:sgl[])
        n81 = local read "Beacon Scales - Right"() -> (w195:sgl[])
        n82 = for {
          N: w192 -> [_]
          tunnel: "Valid Angles - L" -> [w412] mode=indexing
          tunnel: "Beacon Angles - L" -> [w419] mode=indexing
          tunnel: w198 -> [w420] mode=indexing
          tunnel: "Valid Angles -R" -> [w405] mode=indexing
          tunnel: "Beacon Angles -R" -> [w418] mode=indexing
          tunnel: w195 -> [w417] mode=indexing
          tunnel: "Distance Between \nCameras  (*unit)" -> [w416]
          tunnel: [w411] -> w189 mode=indexing
          tunnel: [w410] -> w188 mode=indexing
          tunnel: [w409] -> w190 mode=indexing
          tunnel: [w408] -> w155 mode=indexing
          tunnel: [w407] -> w154 mode=indexing
          tunnel: [w406] -> w153 mode=indexing
          tunnel: w151 -> [w404]
          tunnel: w150 -> [w403]
          # "dY"
          # "dX"
          # "Valid"
          # "If Both Cameras are using Same Beacon Data,\nAverage the 2 independently esitmated positions"
          # "dY"
          # "dX"
          # "dY"
          # "dX"
          n83 = case shown="True" w412 {
            tunnel: w419 -> [_ w497]
            tunnel: [w484 w488] -> w414
            tunnel: [w484 w489] -> w413
            tunnel: w420 -> [_ w487]
            tunnel: w404 -> [_ w486]
            frame False {
              w484 = sgl 0.0
              # "Current Data Set Was Not Valid\nFill with 0\nWill not be used later"
            }
            frame True {
              # "Estimate Distance"
              # "Negate dX if A2>90"
              # "Find LOCAL Coordinate of Each Beacon"
              # "Current - Valid Data Set"
              n84 = call "Beacon_Scale_to_Distance_R0.vi"("Scale - In"=w487, "Current Template - In"=w486) -> ("Distance - Out"=w485:sgl)  [unwired: 9 in]
              n85 = Less?(x=w497, y=sgl 90.0) -> (x < y?=w499:bool)
              n86 = case shown="False" w499 {
                tunnel: w497 -> [w506 w508]
                tunnel: [w504 w509] -> w496
                tunnel: [FALSE TRUE] -> w491
                frame False {
                  # "Negative Y"
                  # "A2 is > 90"
                  n87 = Subtract(x=w506, y=sgl 90.0) -> (x-y=w504:sgl)
                }
                frame True {
                  # "Positive Y"
                  # "A2 is < 90"
                  n88 = Subtract(x=sgl 90.0, y=w508) -> (x-y=w509:sgl)
                }
              }
              "dA2 2" <- w496
              n89 = expression code="(x/180.0)*pi" "degrees to radians"(w496) -> (w494:sgl)
              n90 = expression code="(x/180.0)*pi" "degrees to radians"(w496) -> (w495:sgl)
              n91 = Cosine(x=w494) -> (cos(x)=w492:sgl)
              n92 = Sine(x=w495) -> (sin(x)=w493:sgl)
              n93 = Multiply(x=w485, y=w492) -> (x*y=w489:sgl)
              n94 = Multiply(x=w485, y=w493) -> (x*y=w490:sgl)
              n95 = case shown="True" w491 {
                tunnel: w490 -> [w501 w502]
                tunnel: [w500 w502] -> w488
                frame False {
                  n96 = Negate(x=w501) -> (-x=w500:sgl)
                }
                frame True {
                }
              }
            }
          }
          n97 = case shown="True" w405 {
            tunnel: w418 -> [_ w470]
            tunnel: [w455 w461] -> w407
            tunnel: [w455 w460] -> w408
            tunnel: w417 -> [_ w457]
            tunnel: w416 -> [_ w462]
            tunnel: [w455 w459] -> w406
            tunnel: w403 -> [_ w458]
            frame False {
              w455 = sgl 0.0
              # "Current Data Set Was Not Valid\nFill with 0\nWill not be used later"
            }
            frame True {
              # "Add delta for\nRIGHT camera ONLY"
              # "Estimate Distance"
              # "Negate dX if A2>90"
              # "Find LOCAL Coordinate of Each Beacon"
              # "Current - Valid Data Set"
              n98 = call "Beacon_Scale_to_Distance_R0.vi"("Scale - In"=w457, "Current Template - In"=w458) -> ("Distance - Out"=w456:sgl)  [unwired: 9 in]
              n99 = Less?(x=w470, y=sgl 90.0) -> (x < y?=w472:bool)
              n100 = case shown="False" w472 {
                tunnel: w470 -> [w479 w481]
                tunnel: [w477 w482] -> w469
                tunnel: [FALSE TRUE] -> w464
                frame False {
                  # "Negative Y"
                  # "A2 is > 90"
                  n101 = Subtract(x=w479, y=sgl 90.0) -> (x-y=w477:sgl)
                }
                frame True {
                  # "Positive Y"
                  # "A2 is < 90"
                  n102 = Subtract(x=sgl 90.0, y=w481) -> (x-y=w482:sgl)
                }
              }
              "dA2 3" <- w469
              n103 = expression code="(x/180.0)*pi" "degrees to radians"(w469) -> (w467:sgl)
              n104 = expression code="(x/180.0)*pi" "degrees to radians"(w469) -> (w468:sgl)
              n105 = Cosine(x=w467) -> (cos(x)=w465:sgl)
              n106 = Sine(x=w468) -> (sin(x)=w466:sgl)
              n107 = Multiply(x=w456, y=w465) -> (x*y=w460:sgl)
              n108 = Multiply(x=w456, y=w466) -> (x*y=w463:sgl)
              n109 = case shown="True" w464 {
                tunnel: w463 -> [w474 w475]
                tunnel: [w473 w475] -> w459
                frame False {
                  n110 = Negate(x=w474) -> (-x=w473:sgl)
                }
                frame True {
                }
              }
              n111 = Add(x=w462, y=w459) -> (x+y=w461:sgl)
            }
          }
          n112 = And(x=w412, y=w405) -> (x .and. y?=w415:bool)
          n113 = case shown="False" w415 {
            tunnel: w414 -> [w428 w454]
            tunnel: w413 -> [w425 w453]
            tunnel: w407 -> [w427 w452]
            tunnel: w408 -> [w426 w451]
            tunnel: [w423 w447] -> w411
            tunnel: [w422 w446] -> w410
            tunnel: w412 -> [w424 _]
            tunnel: w405 -> [w429 _]
            tunnel: [w421 TRUE] -> w409
            frame False {
              n114 = Exclusive Or(1:w429, 2:w424) -> (0:w430:bool)
              n115 = case shown="True" w430 {
                tunnel: w428 -> [_ w438]
                tunnel: w427 -> [_ w435]
                tunnel: w426 -> [_ w434]
                tunnel: w425 -> [_ w436]
                tunnel: w424 -> [_ w440]
                tunnel: [w431 w439] -> w423
                tunnel: [w431 w437] -> w422
                tunnel: [FALSE TRUE] -> w421
                frame False {
                  w431 = sgl 0.0
                  # "None are valid,"
                }
                frame True {
                  # "Only 1 beacon is valid,\nUse the valid beacon"
                  n116 = case shown="False" w440 {
                    tunnel: [w442 w444] -> w439
                    tunnel: w438 -> [_ w444]
                    tunnel: [w441 w443] -> w437
                    tunnel: w436 -> [_ w443]
                    tunnel: w435 -> [w442 _]
                    tunnel: w434 -> [w441 _]
                    frame False {
                      # "Left is invalid,\nRight MUST be valid"
                    }
                    frame True {
                      # "Left is Valid"
                    }
                  }
                }
              }
            }
            frame True {
              w448 = sgl 2.0 ("y")
              # "Both are Valid"
              n117 = Add(x=w454, y=w452) -> (x+y=w449:sgl)
              n118 = Add(x=w453, y=w451) -> (x+y=w450:sgl)
              n119 = Divide(x=w450, y=w448) -> (x/y=w446:sgl)
              n120 = Divide(x=w449, y=w448) -> (x/y=w447:sgl)
            }
          }
        }
        "Array" <- w155
        "Array 2" <- w154
        "Array 3" <- w153
        n121 = And(x="Valid Angles - L", y="Valid Angles -R") -> (x .and. y?=w180:bool[])
        n122 = Boolean To (0,1)(Boolean=w180) -> (0, 1=w177:i16[])
        n123 = Add Array Elements(numeric array=w177) -> (sum=w178:i16)
        n124 = Greater?(x=w178, y=1) -> (0:w176:bool)
        n125 = for {
          N: w192 -> [_]
          tunnel: w176 -> [w339]
          tunnel: "Beacon Angles - L" -> [w338] mode=indexing
          tunnel: "Beacon Angles -R" -> [w337] mode=indexing
          tunnel: "Distance Between \nCameras  (*unit)" -> [w336]
          tunnel: "Distance Threshold\nRef Triangles (*unit)" -> [w335]
          tunnel: [w334] -> w163 mode=indexing
          tunnel: [w333] -> _ mode=indexing
          tunnel: [w332] -> w162 mode=indexing
          tunnel: [w331] -> _ mode=indexing
          tunnel: [w330] -> w164 mode=indexing
          tunnel: [w329] -> w170 mode=indexing
          n126 = case shown="True" w339 {
            tunnel: w338 -> [w344 w354]
            tunnel: w337 -> [w343 w353]
            tunnel: w336 -> [_ w345]
            tunnel: w335 -> [_ w346]
            tunnel: [w344 w352] -> w334
            tunnel: [w343 w351] -> w333
            tunnel: [FALSE w350] -> w332
            tunnel: [w341 w349] -> w331
            tunnel: [w341 w348] -> w330
            tunnel: [0 w347] -> w329
            frame False {
              w341 = sgl 1.0
            }
            frame True {
              # "Build Reference Triangle"
              n127 = call "Position Calc_Build Reference Triangle_R1.vi"("A2_in"=w354, "A3_in"=w353, "S1 (Length Between\n Cameras - inches)"=w345, "Distance\nThreshold"=w346) -> ("S2"=w349:sgl, "S3"=w348:sgl, "Direction"=w347:i8, "A2"=w352:sgl, "A3"=w351:sgl, "Accept"=w350:bool)  [unwired: 6 in]
            }
          }
        }
        n128 = for {
          N: w192 -> [_]
          tunnel: w162 -> [w324] mode=indexing
          tunnel: w170 -> [w328] mode=indexing
          tunnel: [w328] -> w172 mode=indexing if=w324
          shift-right: [w327] -> w166
          shift-left: 0 -> [w325]
          # "Only add to array\nif valid distance"
          n129 = Increment(x=w325) -> (x+1=w326:i32)
          n130 = Select(t=w326, s=w324, f=w325) -> (s? t:f=w327:i32)
        }
        n131 = Index Array(array=w172, index=0) -> (element=w173:i32)
        n132 = Equal?(x=w172, y=w173) -> (x = y?=w174:bool[])
        n133 = And Array Elements(Boolean array=w174) -> (logical AND=w168:bool)
        n134 = Greater?(x=w166, y=1) -> (0:w167:bool)
        n135 = And(x=w168, y=w167) -> (x .and. y?=w161:bool)
        n136 = case shown="True" w161 {
          tunnel: w192 -> [w281 w290]
          tunnel: w164 -> [_ w289]
          tunnel: w163 -> [_ w288]
          tunnel: w162 -> [_ w287]
          tunnel: [w280 w286] -> w191
          tunnel: [w279 w285] -> w187
          tunnel: [w279 w284] -> w186
          frame False {
            # "Build Array for False"
            n137 = for {
              N: w281 -> [_]
              tunnel: [sgl 0.0] -> w279 mode=indexing
              tunnel: [FALSE] -> w280 mode=indexing
            }
          }
          frame True {
            n138 = for {
              N: w290 -> [_]
              tunnel: w288 -> [w296] mode=indexing
              tunnel: w289 -> [w295] mode=indexing
              tunnel: [w294] -> w285 mode=indexing
              tunnel: [w293] -> w284 mode=indexing
              tunnel: [w292] -> w286 mode=indexing
              tunnel: w287 -> [w291] mode=indexing
              n139 = case shown="True" w291 {
                selector: w291 -> [w298 w302]
                tunnel: w296 -> [_ w310]
                tunnel: [w297 w300] -> w294
                tunnel: [w297 w301] -> w293
                tunnel: w295 -> [_ w299]
                tunnel: [w298 w302] -> w292
                frame False {
                  w297 = sgl 0.0
                  # "Current Data Set Was Not Valid\nFill with 0\nWill not be used later"
                }
                frame True {
                  # "dY"
                  # "dX"
                  # "Negate dX if A2>90"
                  # "Find LOCAL Coordinate of Each Beacon"
                  # "Current - Valid Data Set"
                  n140 = Less?(x=w310, y=sgl 90.0) -> (x < y?=w312:bool)
                  n141 = case shown="False" w312 {
                    tunnel: w310 -> [w319 w321]
                    tunnel: [w317 w322] -> w309
                    tunnel: [FALSE TRUE] -> w304
                    frame False {
                      # "Negative Y"
                      # "A2 is > 90"
                      n142 = Subtract(x=w319, y=sgl 90.0) -> (x-y=w317:sgl)
                    }
                    frame True {
                      # "Positive Y"
                      # "A2 is < 90"
                      n143 = Subtract(x=sgl 90.0, y=w321) -> (x-y=w322:sgl)
                    }
                  }
                  "dA2 4" <- w309
                  n144 = expression code="(x/180.0)*pi" "degrees to radians"(w309) -> (w307:sgl)
                  n145 = expression code="(x/180.0)*pi" "degrees to radians"(w309) -> (w308:sgl)
                  n146 = Cosine(x=w307) -> (cos(x)=w305:sgl)
                  n147 = Sine(x=w308) -> (sin(x)=w306:sgl)
                  n148 = Multiply(x=w299, y=w305) -> (x*y=w301:sgl)
                  n149 = Multiply(x=w299, y=w306) -> (x*y=w303:sgl)
                  n150 = case shown="True" w304 {
                    tunnel: w303 -> [w314 w315]
                    tunnel: [w313 w315] -> w300
                    frame False {
                      n151 = Negate(x=w314) -> (-x=w313:sgl)
                    }
                    frame True {
                    }
                  }
                }
              }
            }
          }
        }
        n152 = Subtract(x=sgl 1.0, y="Triangle Based\nWeight") -> (x-y=w183:sgl)
        "Scale Based\nWeight" <- w183
        n153 = for {
          N: w192 -> [_]
          tunnel: w191 -> [w359] mode=indexing
          tunnel: w190 -> [w358] mode=indexing
          tunnel: w189 -> [w363] mode=indexing
          tunnel: w188 -> [w362] mode=indexing
          tunnel: w187 -> [w365] mode=indexing
          tunnel: w186 -> [w364] mode=indexing
          tunnel: "Triangle Based\nWeight" -> [w361]
          tunnel: w183 -> [w360]
          tunnel: [w357] -> w160 mode=indexing
          tunnel: [w356] -> w182 mode=indexing
          tunnel: [w355] -> w181 mode=indexing
          # "If Beacon info \nis available from\nboth"
          n154 = And(x=w359, y=w358) -> (x .and. y?=w366:bool)
          n155 = case shown="True" w366 {
            selector: w366 -> [_ w392]
            tunnel: w365 -> [w373 w400]
            tunnel: w364 -> [w371 w401]
            tunnel: w363 -> [w369 w399]
            tunnel: w362 -> [w368 w398]
            tunnel: w361 -> [_ w402]
            tunnel: w360 -> [_ w397]
            tunnel: [w372 w390] -> w355
            tunnel: [w374 w391] -> w356
            tunnel: w359 -> [w375 _]
            tunnel: w358 -> [w370 _]
            tunnel: [w367 w392] -> w357
            frame False {
              n156 = case shown="False" w375 {
                selector: w375 -> [_ w387]
                tunnel: [w380 w389] -> w374
                tunnel: w373 -> [_ w389]
                tunnel: [w378 w388] -> w372
                tunnel: w371 -> [_ w388]
                tunnel: w370 -> [w381 _]
                tunnel: w369 -> [w379 _]
                tunnel: w368 -> [w377 _]
                tunnel: [w376 w387] -> w367
                frame False {
                  n157 = case shown="False" w381 {
                    selector: w381 -> [w382 w384]
                    tunnel: [w383 w386] -> w380
                    tunnel: w379 -> [_ w386]
                    tunnel: [w383 w385] -> w378
                    tunnel: w377 -> [_ w385]
                    tunnel: [w382 w384] -> w376
                    frame False {
                      w383 = sgl 0.0
                      # "None avail"
                    }
                    frame True {
                    }
                  }
                }
                frame True {
                }
              }
            }
            frame True {
              n158 = Multiply(x=w400, y=w402) -> (x*y=w396:sgl)
              n159 = Multiply(x=w401, y=w402) -> (x*y=w394:sgl)
              n160 = Multiply(x=w399, y=w397) -> (x*y=w395:sgl)
              n161 = Multiply(x=w398, y=w397) -> (x*y=w393:sgl)
              n162 = Add(x=w396, y=w395) -> (x+y=w391:sgl)
              n163 = Add(x=w394, y=w393) -> (x+y=w390:sgl)
            }
          }
        }
        "Valid Beacon Sets_" <- w160
        n164 = Boolean To (0,1)(Boolean=w160) -> (0, 1=w203:i16[])
        n165 = Add Array Elements(numeric array=w203) -> (sum=w202:i16)
        n166 = Greater?(x=w202, y=i16 1) -> (0:w200:bool)
        n167 = case shown="True" w200 {
          tunnel: w227 -> [_ w601]
          tunnel: [0.0 ("f") w600] -> w223
          tunnel: [w513 w599] -> w141
          tunnel: w219 -> [_ w520]
          tunnel: w218 -> [_ w598]
          tunnel: [FALSE w597] -> w139
          tunnel: [FALSE w596] -> w137
          tunnel: w211 -> [_ w595]
          tunnel: [sgl 0.0 w593] -> w204
          tunnel: "Distance Between \nCameras  (*unit)" -> [_ w532]
          tunnel: w182 -> [_ w531]
          tunnel: w181 -> [_ w530]
          tunnel: w160 -> [_ w529]
          tunnel: w192 -> [_ w528]
          frame False {
            w512 = 0.0 ("f")
            n168 = Bundle("f"=w512, "f"=w512) -> (w513:cluster{"f":dbl, "f":dbl})  [unwired: 1 in]
          }
          frame True {
            w565 = sgl 2.0
            w582 = 0
            # "Current Orientaiton"
            # "Valid Position Ccount\n(within moving avg\nwinfow)"
            # "Valid Position Ccount"
            # "Only Apply This Filtering \nif 3 or More Beacons Still Valid"
            # "Orientation Value"
            # "Orientation Valid"
            # "Y (current)"
            # "X (current)"
            # "Number of Valid\nPrevious Orientations"
            # "More than 1 Previous\nValid Positions"
            # "More than\n2previous position\navailable"
            # "Choose Beacon Set\nwith Lowest Std Dev"
            # "Y value cannot be negative"
            # "Find New # Of Valid Beacons"
            # "Adjust/Normalize\nLocal Beacon Positions\nusing Line of Best fit"
            # "# Valid\nData Sets"
            # "cam, y"
            # "cam, x"
            # "Calculate dX and dY\nfor right cam"
            # "Average dX and dY from each (valid) beacon to find position of each camera\n\nthen average all  positions for each camera find center between"
            # "Convert Slope\nto Radians"
            # "*rotate CCW in rad"
            # "Rotate Coordinate\n System by Slope"
            n169 = Boolean To (0,1)(Boolean=w520) -> (0, 1=w549:i16[])
            n170 = Initialize Array(u8 0, "Moving Average\nWindow Length") -> (w525:u8[])
            n171 = Add Array Elements(numeric array=w549) -> (sum=w519:i16)
            n172 = Greater?(x=w519, y=0) -> (0:w522:bool)
            n173 = while {
              shift-right: [w603] -> w523
              shift-left: w525 -> [w605]
              tunnel: w520 -> [w610] mode=indexing
              shift-right: [w609] -> w521
              shift-left: u8 0 -> [w611]
              tunnel: "Moving Average\nWindow Length" -> [w602]
              i -> [w604]
              stop <- w606 stop-if-true
              # "Grab Last 2 Valid Position Indexes"
              n174 = case shown="True" w610 {
                tunnel: w611 -> [w613 w615]
                tunnel: [w613 w618] -> w609
                tunnel: w605 -> [w612 w617]
                tunnel: w604 -> [_ w616]
                tunnel: [w612 w614] -> w603
                frame False {
                }
                frame True {
                  # "Update Index\nto use"
                  # "Increment\nValid Count"
                  n175 = Replace Array Subset(array=w617, new element=w616, index=w615) -> (w614:u8[])
                  n176 = Increment(x=w615) -> (x+1=w618:u8)
                }
              }
              n177 = Greater Or Equal?(x=w609, y=w602) -> (x >= y?=w608:bool)
              n178 = Greater Or Equal?(x=w604, y=w602) -> (x >= y?=w607:bool)
              n179 = Or(x=w608, y=w607) -> (x .or. y?=w606:bool)
            }
            n180 = Bundle(w531, w530) -> (→"LOCAL\nBeacon Coordinates\nRelative to Robot" →"Local Coordinates - Calculated":cluster{sgl[], sgl[]})  [unwired: 1 in]
            n181 = call "Coordinate_Outlier_Filtering_R2.vi"("Num of Beacons"=w528, "Max Std Dev(all 5)"="Max Std Dev (5)", "X in"=w531, "Valid Data\nSets in"=w529, "Y in"=w530, "Max Std Dev( 4 )"="Max Std Dev (4)", "Max Std Dev (3)"="Max Std Dev (3)") -> ("Y out"=w542:sgl[], "X out"=w543:sgl[], "Valid Beacons\nout"=w540:bool[], "Slope out"=w548:dbl)  [unwired: 3 in, 2 out]
            n182 = Inverse Tangent(1:w548) -> (0:w561:dbl)
            n183 = expression code="(x/pi)*180.0" "radians to degrees"(w561) -> (w547:dbl)
            n184 = Boolean To (0,1)(Boolean=w540) -> (0, 1=w539:i16[])
            n185 = To Single Precision Float(number=w547) -> (single precision float=w593:sgl)
            n186 = case shown="True" w522 {
              tunnel: [w628 w648] -> w596
              tunnel: w598 -> [_ w650]
              tunnel: w593 -> [w629 w645]
              tunnel: [w627 w649] -> w600
              tunnel: w595 -> [_ _]
              tunnel: w523 -> [_ w646]
              tunnel: w521 -> [_ w637]
              frame False {
                # "Since no history available,\ncheck that current is with 0-360"
                # "Use Current Orientation bc \nPrevious are not available"
                # "New Position\nValid"
                n187 = In Range and Coerce(upper limit=sgl 360.0, x=w629, lower limit=sgl -360.0 ("upper limit")) -> (In Range?=w628:bool)  [unwired: 1 out]
                n188 = Select(t=w629, s=w628, f=sgl 0.0) -> (s? t:f=w627:sgl)
              }
              frame True {
                # "Calculate New, Weighted\nOrientation"
                # "Moving Average Out"
                n189 = local read "Last Position"() -> (w635:cluster{"X":sgl, "Y":sgl})
                n190 = Unbundle By Name(w635) -> ()  [unwired: 1 out]
                n191 = call "Scaling and Mapping2"() -> ("Scaled Signals"=w634:dynamicdata)  [unwired: 10 in, 1 out]
                n192 = for {
                  N: w637 -> [_]
                  shift-right: [w674] -> w643
                  shift-left: 0.0 -> [w673]
                  tunnel: w646 -> [w672] mode=indexing
                  tunnel: w650 -> [w670]
                  # "Fetch Last Valid Values\nand Sum"
                  n193 = Index Array(array=w670, index=w672) -> (element=w671:sgl)
                  n194 = Add(x=w671, y=w673) -> (x+y=w674:dbl)
                }
                n195 = To Single Precision Float(number=w634) -> (single precision float=w633:sgl)
                "New Orientation\nWeight" <- w633
                n196 = Subtract(x=sgl 1.0, y=w633) -> (x-y=w642:sgl)
                n197 = Multiply(x=w645, y=w633) -> (x*y=w640:sgl)
                n198 = Multiply(x=w642, y=w643) -> (x*y=w638:dbl)
                n199 = To Double Precision Float(number=w637) -> (double precision float=w636:dbl)
                n200 = Divide(x=w638, y=w636) -> (x/y=w639:dbl)
                n201 = Add(x=w640, y=w639) -> (x+y=w641:dbl)
                n202 = Greater Than 0?(x=w637) -> (x > 0?=w647:bool)
                n203 = case shown="True" w647 {
                  tunnel: w641 -> [w654 w660]
                  tunnel: w646 -> [_ w667]
                  tunnel: w650 -> [_ w666]
                  tunnel: [w653 w659] -> w649
                  tunnel: [w652 w662] -> w648
                  frame False {
                    # "No Pevious is Available to Compare\ncheck that current is real angle"
                    n204 = In Range and Coerce(upper limit=sgl 360.0, x=w654, lower limit=sgl -360.0 ("upper limit")) -> (In Range?=w652:bool)  [unwired: 1 out]
                    n205 = Select(t=w654, s=w652, f=sgl 0.0) -> (s? t:f=w653:dbl)
                  }
                  frame True {
                    # "Check That New Value\nis within Range of Old\n(avg)"
                    # "(X1 - X2)^2"
                    # "Previous"
                    # "Pevious is Available to Compare"
                    n206 = Index Array(array=w667, index=u8 0) -> (element=w668:u8)
                    n207 = Index Array(array=w666, index=w668) -> (element=w665:sgl)
                    n208 = Subtract(x=w665, y=w660) -> (x-y=w664:dbl)
                    n209 = Absolute Value(x=w664) -> (abs(x)=w663:dbl)
                    n210 = Less Or Equal?(x=w663, y="New Orientation \nThreshold") -> (x <= y?=w662:bool)
                    n211 = Select(t=w660, s=w662, f=sgl 0.0) -> (s? t:f=w659:dbl)
                  }
                }
              }
            }
            n212 = Add Array Elements(numeric array=w539) -> (sum=w538:i16)
            n213 = Greater?(x=w538, y=i16 2) -> (0:w536:bool)
            n214 = case shown="True" w536 {
              tunnel: w528 -> [_ w626]
              tunnel: w540 -> [w619 w625]
              tunnel: w543 -> [_ w624]
              tunnel: w542 -> [_ w623]
              tunnel: [w619 w622] -> w541
              tunnel: "Distance\nBetween Beacons" -> [_ w621]
              tunnel: "Distance\nBetween Beacons \n- Tolerance" -> [_ w620]
              frame False {
                # "Don't apply filtering,\nnot enough data points"
              }
              frame True {
                # "This will filter beacons if they are calculate to be \ntoo close to each other. The beacon(s) that is\n discarded is chosen based distance between each/every\nbeacon,. Capable of filtering as long as 1/2 of sample\nset has uniform distances (between beacons)."
                # "Validate Distance Between\nEach Beacon"
                n215 = call "Beacon_Filtering_Inter_Beacon_Distance_R1.vi"("Num of Beacons"=w626, "Inter Beacon\nReal Distance"=w621, "X in"=w624, "Inter Beacon\ndelta Threshold"=w620, "Y in"=w623, "Valid Data\nSets in"=w625) -> ("Beacons Valid - Out"=w622:bool[])  [unwired: 9 in]
              }
            }
            "Post Filtering\n- Valid Beacons" <- w541
            n216 = Increment(x=w528) -> (x+1=w583:i8)
            n217 = for {
              N: w583 -> [_]
              tunnel: [w793] -> w584 mode=indexing
              tunnel: w543 -> [w789]
              tunnel: w542 -> [w792]
              tunnel: [w791] -> w585 mode=indexing
              tunnel: w532 -> [w788]
              i -> [w790]
              # "Build Array's of Coordinates\nFor All Objects"
              n218 = Greater Than 0?(x=w790) -> (x > 0?=w794:bool)
              n219 = case shown="True" w794 {
                tunnel: [w796 w802] -> w793
                tunnel: w789 -> [w799 _]
                tunnel: w792 -> [w798 _]
                tunnel: [w795 0.0] -> w791
                tunnel: w790 -> [w800 _]
                tunnel: w788 -> [_ w802]
                frame True {
                  # "Rest of Array is\nBeacon Coordinates"
                  n220 = Decrement(x=w800) -> (x-1=w797:i32)
                  n221 = Index Array(array=w799, index=w797) -> (element=w796:sgl)
                  n222 = Index Array(array=w798, index=w797) -> (element=w795:sgl)
                }
                frame False {
                  # "First object is the\nother Camera\n\nthis coordinate\nis simply:\nx = 0\ny = distance btween cams"
                }
              }
            }
            n223 = Bundle(w584, w585) -> (→"All Object Coordinates \n- Local" →"Local Coordinates - Normalized":cluster{sgl[], dbl[]})  [unwired: 1 in]
            n224 = expression code="(x/180.0)*pi" "degrees to radians"(w600) -> (w546:dbl)
            n225 = call-poly <vilib>:"2D Cartesian Coordinate Rotation.vi"("theta"=w546, "Y"=w585, "X"=w584) -> ("Y Out"=w562:dbl[], "X Out"=w563:dbl[])  [unwired: 6 in, 1 out]
            n226 = Bundle("X Out"=w563, "Y Out"=w562) -> (→"All Object Coordinates \n- Local - Rotated" →"Local Coordinates - Rotated":cluster{"X Out":dbl[], "Y Out":dbl[]})  [unwired: 1 in]
            n227 = Index Array(array=w562, index=w582) -> (element=w558:dbl)
            n228 = Index Array(array=w563, index=w582) -> (element=w581:dbl)
            n229 = for {
              N: w528 -> [_]
              tunnel: w562 -> [w784]
              tunnel: w563 -> [w785]
              tunnel: w581 -> [w783]
              tunnel: w558 -> [w782]
              tunnel: [w781] -> w555 mode=indexing
              tunnel: [w780] -> w554 mode=indexing
              tunnel: [w779] -> w533 mode=indexing
              tunnel: [w778] -> w556 mode=indexing
              i -> [w787]
              n230 = Increment(x=w787) -> (x+1=w786:i32)
              n231 = Index Array(array=w784, index=w786) -> (element=w778:dbl)
              n232 = Index Array(array=w785, index=w786) -> (element=w779:dbl)
              n233 = Subtract(x=w778, y=w782) -> (x-y=w780:dbl)
              n234 = Subtract(x=w779, y=w783) -> (x-y=w781:dbl)
            }
            n235 = Bundle(w555, w554) -> (→"dX, dY\nRight Cam":cluster{dbl[], dbl[]})  [unwired: 1 in]
            n236 = Bundle(w533, w556) -> (→"dX, dY\nLeft Cam":cluster{dbl[], dbl[]})  [unwired: 1 in]
            n237 = Unbundle("Real Beacon\n - Coordinates") -> ("X"=w579:dbl[], "Y"=w559:dbl[])
            n238 = Boolean To (0,1)(Boolean=w541) -> (0, 1=w557:i16[])
            n239 = for {
              N: w528 -> [_]
              tunnel: w541 -> [w764] mode=indexing
              tunnel: w579 -> [w761] mode=indexing
              tunnel: w559 -> [w760] mode=indexing
              tunnel: w533 -> [w763] mode=indexing
              tunnel: w556 -> [w759] mode=indexing
              tunnel: w555 -> [w762] mode=indexing
              tunnel: w554 -> [w758] mode=indexing
              tunnel: [w757] -> w578 mode=indexing
              tunnel: [w756] -> w577 mode=indexing
              tunnel: [w755] -> w576 mode=indexing
              tunnel: [w754] -> w575 mode=indexing
              n240 = case shown="True" w764 {
                tunnel: w763 -> [_ w777]
                tunnel: w762 -> [_ w776]
                tunnel: w761 -> [_ w767]
                tunnel: w760 -> [_ w766]
                tunnel: w759 -> [_ w775]
                tunnel: w758 -> [_ w768]
                tunnel: [w765 w773] -> w757
                tunnel: [w765 w772] -> w756
                tunnel: [w765 w771] -> w755
                tunnel: [w765 w770] -> w754
                frame False {
                  w765 = sgl 0.0
                  # "Add Nothing"
                }
                frame True {
                  # "realX = beaconX + dY\nrealY = beaconY + (-dx)"
                  # "Right Cam"
                  # "Left Cam"
                  # "dX = -dX\nSwap dX, dY"
                  # "Translate to Real Coordinates\nOnly Apply for Valid Beacons"
                  n241 = Negate(x=w777) -> (-x=w774:dbl)
                  n242 = Negate(x=w776) -> (-x=w769:dbl)
                  n243 = Add(x=w767, y=w775) -> (x+y=w773:dbl)
                  n244 = Add(x=w766, y=w774) -> (x+y=w772:dbl)
                  n245 = Add(x=w767, y=w768) -> (x+y=w771:dbl)
                  n246 = Add(x=w766, y=w769) -> (x+y=w770:dbl)
                }
              }
            }
            n247 = Add Array Elements(numeric array=w557) -> (sum=w560:i16)
            n248 = Add Array Elements(numeric array=w578) -> (sum=w574:dbl)
            n249 = Add Array Elements(numeric array=w577) -> (sum=w573:dbl)
            n250 = Add Array Elements(numeric array=w576) -> (sum=w572:dbl)
            n251 = Add Array Elements(numeric array=w575) -> (sum=w571:dbl)
            n252 = Divide(x=w574, y=w560) -> (x/y=w570:dbl)
            n253 = Divide(x=w573, y=w560) -> (x/y=w568:dbl)
            n254 = Divide(x=w572, y=w560) -> (x/y=w569:dbl)
            n255 = Divide(x=w571, y=w560) -> (x/y=w567:dbl)
            n256 = Bundle(w570, w568) -> (→"Left Camera Real Coordinates":cluster{dbl, dbl})  [unwired: 1 in]
            n257 = Bundle(w569, w567) -> (→"Right Camera Real Coordinate":cluster{dbl, dbl})  [unwired: 1 in]
            n258 = Add(x=w570, y=w569) -> (x+y=w566:dbl)
            n259 = Add(x=w568, y=w567) -> (x+y=w564:dbl)
            n260 = Divide(x=w566, y=w565) -> (x/y=w517:dbl)
            n261 = Divide(x=w564, y=w565) -> (x/y=w518:dbl)
            n262 = Bundle(w517, w518) -> (→"Robot Coordinates":cluster{dbl, dbl})  [unwired: 1 in]
            n263 = Less Than 0?(x=w518) -> ()  [unwired: 1 out]
            n264 = case shown="True" w522 {
              tunnel: w519 -> [_ _]
              tunnel: w517 -> [w679 w703]
              tunnel: [w680 w713] -> w597
              tunnel: w601 -> [_ w707]
              tunnel: w518 -> [w678 w690]
              tunnel: [w677 w717] -> w599
              tunnel: "Max X (arena)" -> [w676 w712]
              tunnel: "Max Y (arena)" -> [w675 w711]
              tunnel: w523 -> [_ w709]
              tunnel: w521 -> [_ w708]
              frame False {
                # "New Position\nValid"
                # "Since no history available,\ncheck that current is within\nthe bounds of the arena size"
                # "Use Current Position bc \nPrevious are not available"
                n265 = In Range and Coerce(upper limit=w676, x=w679, lower limit=sgl 0.0 ("upper limit")) -> (In Range?=w682:bool)  [unwired: 1 out]
                n266 = In Range and Coerce(upper limit=w675, x=w678, lower limit=sgl 0.0 ("upper limit")) -> (In Range?=w681:bool)  [unwired: 1 out]
                n267 = Bundle(w679, w678) -> (w677:cluster{dbl, dbl})  [unwired: 1 in]
                n268 = And(x=w682, y=w681) -> (x .and. y?=w680:bool)
              }
              frame True {
                w710 = 0.0
                # "Change Y weight depending\non previous X position in course"
                # "If needed, make seperate FOR Loop for \nY only... Using more previous values than X"
                # "New Y"
                # "New X"
                # "Only consider if velocity is\ngreater than certain speed"
                # "Weighted Robot \nCoordinates"
                # "Position\nValid\n(current)"
                n269 = local read "Last Position"() -> (w688:cluster{"X":sgl, "Y":sgl})
                n270 = Unbundle By Name(w688) -> ("X"=w687:sgl)
                n271 = for {
                  N: w708 -> [_]
                  shift-right: [w726] -> w706
                  shift-left: w710 -> [w725]
                  shift-right: [w724] -> w691
                  shift-left: w710 -> [w723]
                  tunnel: w709 -> [w721] mode=indexing
                  tunnel: w707 -> [w719]
                  # "Fetch Last Valid Values\nand Sum"
                  n272 = Index Array(array=w719, index=w721) -> (element=w720:cluster{sgl, sgl})
                  n273 = Unbundle(w720) -> (w722:sgl, w718:sgl)
                  n274 = Add(x=w718, y=w723) -> (x+y=w724:dbl)
                  n275 = Add(x=w722, y=w725) -> (x+y=w726:dbl)
                }
                n276 = call "Scaling and Mapping"("Signals"=w687) -> ("Scaled Signals"=w686:dynamicdata)  [unwired: 9 in, 1 out]
                n277 = To Single Precision Float(number=w686) -> (single precision float=w685:sgl)
                "New Position\nWeight (Y coord)" <- w685
                n278 = Subtract(x=sgl 1.0, y="New Position\nWeight (X coord)") -> (x-y=w705:sgl)
                n279 = Subtract(x=sgl 1.0, y=w685) -> (x-y=w689:sgl)
                n280 = To Single Precision Float(number=w708) -> (single precision float=w697:sgl)
                n281 = Multiply(x=w705, y=w706) -> (x*y=w698:dbl)
                n282 = Multiply(x=w691, y=w689) -> (x*y=w699:dbl)
                n283 = Divide(x=w698, y=w697) -> (x/y=w695:dbl)
                n284 = Divide(x=w699, y=w697) -> (x/y=w696:dbl)
                n285 = Multiply(x="New Position\nWeight (X coord)", y=w703) -> (x*y=w701:dbl)
                n286 = Multiply(x=w690, y=w685) -> (x*y=w700:dbl)
                n287 = Add(x=w701, y=w695) -> (x+y=w694:dbl)
                n288 = Add(x=w700, y=w696) -> (x+y=w693:dbl)
                n289 = Greater Than 0?(x=w708) -> (x > 0?=w716:bool)
                n290 = case shown="True" w716 {
                  tunnel: w694 -> [w731 w738]
                  tunnel: w693 -> [w730 w737]
                  tunnel: w709 -> [_ w750]
                  tunnel: w707 -> [_ w749]
                  tunnel: [w728 w738] -> w715
                  tunnel: [w727 w737] -> w714
                  tunnel: [w732 w739] -> w713
                  tunnel: w712 -> [w734 _]
                  tunnel: w711 -> [w733 _]
                  frame False {
                    w729 = sgl 0.0 ("upper limit")
                    # "Check that within bounds of arena"
                    # "No Pevious is Available to Compare"
                    n291 = In Range and Coerce(upper limit=w734, x=w731, lower limit=w729) -> (In Range?=w736:bool)  [unwired: 1 out]
                    n292 = In Range and Coerce(upper limit=w733, x=w730, lower limit=w729) -> (In Range?=w735:bool)  [unwired: 1 out]
                    n293 = And(x=w736, y=w735) -> (x .and. y?=w732:bool)
                    n294 = Select(t=w731, s=w732, f=w729) -> (s? t:f=w728:dbl)
                    n295 = Select(t=w730, s=w732, f=w729) -> (s? t:f=w727:dbl)
                  }
                  frame True {
                    # "New"
                    # "(Y1 - Y2)^2"
                    # "(X1 - X2)^2"
                    # "Previous"
                    # "Pevious is Available to Compare"
                    n296 = Index Array(array=w750, index=u8 0) -> (element=w752:u8)
                    n297 = Index Array(array=w749, index=w752) -> (element=w751:cluster{sgl, sgl})
                    n298 = Unbundle(w751) -> (w741:sgl, w740:sgl)
                    n299 = Subtract(x=w741, y=w738) -> (x-y=w746:dbl)
                    n300 = Subtract(x=w737, y=w740) -> (x-y=w745:dbl)
                    n301 = Square(x=w746) -> (x^2=w744:dbl)
                    n302 = Square(x=w745) -> (x^2=w743:dbl)
                    n303 = Add(x=w744, y=w743) -> (x+y=w747:dbl)
                    n304 = Square Root(x=w747) -> (sqrt(x)=w742:dbl)
                    n305 = Less Or Equal?(x=w742, y="New Position \nThreshold") -> (x <= y?=w739:bool)
                  }
                }
                n306 = Bundle("upper limit"=w715, "upper limit"=w714) -> (w717:cluster{"upper limit":dbl, "upper limit":dbl})  [unwired: 1 in]
              }
            }
          }
        }
        "Orietnation\n(current)" <- w204
        n307 = local read "Current Template - Left"() -> (w135:T1)
        n308 = local read "Current Template - Left"() -> (w133:T1)
        n309 = Equal?(x=w135, y=w133) -> (x = y?=w131:bool)
        n310 = Equal?(x=w133, y=T1."Range 0" ("Current Template - Left")) -> (x = y?=w130:bool)
        n311 = And(x=w131, y=w130) -> (x .and. y?=w132:bool)
        n312 = case shown="False" w132 {
          tunnel: [w230 w248] -> w138
          tunnel: [w229 w247] -> w136
          tunnel: w139 -> [w230 _]
          tunnel: w137 -> [w229 _]
          tunnel: [w228 w244] -> w140
          tunnel: w141 -> [w228 _]
          frame False {
            # "Disabled  -- ignore and pass all values thru"
          }
          frame True {
            w256 = 0 ("index")
            # "At Least 1?"
            # "# valid (0,1,2)"
            # "Only Stores in index\n0 for this special case"
            # "Curve Fitting for Range 0"
            # "Latch Y position"
            n313 = local read "Beacons Found\n- Left (Bool Array) 2"() -> (w265:bool[])
            n314 = local read "Beacons Found\n- Right (Bool Array)"() -> (w266:bool[])
            n315 = local read "Beacon Scales - Right"() -> (w257:sgl[])
            n316 = local read "Beacon Scales - Left"() -> (w258:sgl[])
            n317 = Index Array(array=w265, index=w256) -> (element=w264:bool)
            n318 = Index Array(array=w266, index=w256) -> (element=w259:bool)
            n319 = Index Array(array=w258, index=w256) -> (element=w237:sgl)
            n320 = Index Array(array=w257, index=w256) -> (element=w232:sgl)
            n321 = Equal To 0?(x=w232) -> (x = 0?=w234:bool)
            n322 = Select(t=1.0, s=w234, f=w232) -> (s? t:f=w231:dbl)
            n323 = Power Of X(1:w231, 2:-0.826) -> (0:w243:dbl)
            n324 = Select(t=sgl 1.0, s=w264, f=sgl 0.0) -> (s? t:f=w255:sgl)
            n325 = Power Of X(1:w237, 2:-0.826) -> (0:w238:dbl)
            n326 = Select(t=sgl 1.0, s=w259, f=sgl 0.0) -> (s? t:f=w254:sgl)
            n327 = Multiply(x=93.909, y=w243) -> (x*y=w236:dbl)
            n328 = Multiply(x=w254, y=w236) -> (x*y=w252:dbl)
            n329 = Multiply(x=93.909, y=w238) -> (x*y=w235:dbl)
            n330 = Multiply(x=w255, y=w235) -> (x*y=w253:dbl)
            n331 = Add(x=w255, y=w254) -> (x+y=w249:sgl)
            n332 = Add(x=w253, y=w252) -> (x+y=w251:dbl)
            n333 = local read "Last Position"() -> (w267:cluster{"X":sgl, "Y":sgl})
            n334 = Greater Than 0?(x=w249) -> (x > 0?=w250:bool)
            n335 = case shown="False" w250 {
              selector: w250 -> [w268 w270]
              tunnel: w251 -> [_ w273]
              tunnel: w249 -> [_ w272]
              tunnel: [sgl 0.0 w271] -> w245
              tunnel: [w268 w270] -> w248
              tunnel: [w268 w270] -> w247
              frame False {
              }
              frame True {
                # "Avg Values"
                n336 = Divide(x=w273, y=w272) -> (x/y=w271:dbl)
              }
            }
            n337 = Unbundle(w267) -> ("Y"=w246:sgl)  [unwired: 1 out]
            n338 = Bundle(w245, "Y"=w246) -> (w244:cluster{dbl, "Y":sgl})  [unwired: 1 in]
          }
        }
        n339 = And(x=w138, y=w136) -> (x .and. y?=w156:bool)
        "Position Valid" <- w156
        n340 = Exclusive Or(1:w136, 2:w138) -> (0:w212:bool)
        n341 = case shown="True" w156 {
          tunnel: [w809 w812] -> w157
          tunnel: [w810 w811] -> w149
          tunnel: w223 -> [_ w812]
          tunnel: w140 -> [_ w811]
          tunnel: w212 -> [_ _]
          frame False {
            w809 = sgl 0.0 ("f")
            n342 = Bundle("f"=w809, "f"=w809) -> (w810:cluster{"f":sgl, "f":sgl})  [unwired: 1 in]
          }
          frame True {
            # "For Servos"
            n343 = shared-variable "RT myRIO Target - Overlord\\Localization_Variables_r0.lvlib\\Last Robot Position"(w811) -> ()  [unwired: 1 in, 1 out]
            "Last Orientation" <- w812
            "Last Position" <- w811
          }
        }
        "Robot Coordinates - Avgd" <- w149
        "Orientation Avgd" <- w157
        n344 = local read "History Size"() -> (w206:u8)
        n345 = Decrement(x=w206) -> (x-1=w207:u8)
        n346 = for {
          N: w206 -> [_]
          shift-right: [w850] -> w225
          shift-left: w222 -> [w849]
          tunnel: w149 -> [w848]
          tunnel: w207 -> [w847]
          i -> [w846]
          n347 = Subtract(x=w847, y=w846) -> (x-y=w845:i32)
          n348 = Equal To 0?(x=w845) -> (x = 0?=w844:bool)
          n349 = case shown="False" w844 {
            tunnel: w845 -> [w852 w857]
            tunnel: w849 -> [w855 w858]
            tunnel: [w853 w859] -> w850
            tunnel: w848 -> [_ w856]
            frame False {
              n350 = Decrement(x=w852) -> (x-1=w851:i32)
              n351 = Index Array(array=w855, index=w851) -> (element=w854:cluster{sgl, sgl})
              n352 = Replace Array Subset(array=w855, new element=w854, index=w852) -> (w853:cluster{sgl, sgl}[])
            }
            frame True {
              n353 = Replace Array Subset(array=w858, new element=w856, index=w857) -> (w859:cluster{sgl, sgl}[])
            }
          }
        }
        n354 = Unbundle(w149) -> ("upper limit"=w159:dbl, "upper limit"=w158:dbl)
        n355 = shared-variable "RT myRIO Target - Overlord\\Localization_Variables_r0.lvlib\\loc_x"(w159) -> ()  [unwired: 1 in, 1 out]
        n356 = shared-variable "RT myRIO Target - Overlord\\Localization_Variables_r0.lvlib\\loc_y"(w158) -> ()  [unwired: 1 in, 1 out]
        n357 = shared-variable "RT myRIO Target - Overlord\\Localization_Variables_r0.lvlib\\loc_theta"(w157) -> ()  [unwired: 1 in, 1 out]
        n358 = shared-variable "RT myRIO Target - Overlord\\Localization_Variables_r0.lvlib\\loc_flag"(w156) -> ()  [unwired: 1 in, 1 out]
        n359 = Decrement(x=w206) -> (x-1=w208:u8)
        n360 = for {
          N: w206 -> [_]
          shift-right: [w834] -> w226
          shift-left: w221 -> [w833]
          tunnel: w157 -> [w832]
          tunnel: w208 -> [w831]
          i -> [w830]
          n361 = Subtract(x=w831, y=w830) -> (x-y=w828:i32)
          n362 = Equal To 0?(x=w828) -> (x = 0?=w829:bool)
          n363 = case shown="False" w829 {
            tunnel: w828 -> [w836 w841]
            tunnel: w833 -> [w839 w842]
            tunnel: [w837 w843] -> w834
            tunnel: w832 -> [_ w840]
            frame False {
              # "Shift"
              n364 = Decrement(x=w836) -> (x-1=w835:i32)
              n365 = Index Array(array=w839, index=w835) -> (element=w838:sgl)
              n366 = Replace Array Subset(array=w839, new element=w838, index=w836) -> (w837:sgl[])
            }
            frame True {
              # "insert new"
              n367 = Replace Array Subset(array=w842, new element=w840, index=w841) -> (w843:sgl[])
            }
          }
        }
        n368 = Decrement(x=w206) -> (x-1=w205:u8)
        n369 = for {
          N: w206 -> [_]
          shift-right: [w819] -> w224
          shift-left: w220 -> [w818]
          tunnel: w156 -> [w817]
          tunnel: w205 -> [w816]
          i -> [w815]
          n370 = Subtract(x=w816, y=w815) -> (x-y=w813:i32)
          n371 = Equal To 0?(x=w813) -> (x = 0?=w814:bool)
          n372 = case shown="False" w814 {
            tunnel: w818 -> [w824 w826]
            tunnel: [w822 w827] -> w819
            tunnel: w817 -> [_ w825]
            tunnel: w813 -> [w820 _]
            frame False {
              n373 = Decrement(x=w820) -> (x-1=w821:i32)
              n374 = Index Array(array=w824, index=w821) -> (element=w823:bool)
              n375 = Replace Array Subset(array=w824, new element=w823, index=w820) -> (w822:bool[])
            }
            frame True {
              n376 = Replace Array Subset(array=w826, new element=w825) -> (w827:bool[])  [unwired: 1 in]
            }
          }
        }
        n377 = Boolean To (0,1)(Boolean=w224) -> (0, 1=w217:i16[])
        n378 = Add Array Elements(numeric array=w217) -> (sum=w216:i16)
        n379 = Greater Or Equal?(x=w216, y=i16 2) -> (x >= y?=w152:bool)
        "Position \nLock Status" <- w152
        n380 = shared-variable "RT myRIO Target - Overlord\\Localization_Variables_r0.lvlib\\Position_Lock"(w152) -> ()  [unwired: 1 in, 1 out]
        n381 = case shown="True" w156 {
          tunnel: w149 -> [_ w808]
          frame False {
          }
          frame True {
            # "update debug graph\nif current is valid"
            n382 = Unbundle(w808) -> ("upper limit"=w807:dbl, "upper limit"=w806:dbl)
            n383 = Build Array(w806) -> (w804:dbl[])
            n384 = Build Array(w807) -> (w805:dbl[])
            n385 = Bundle(w805, w804) -> (→"Real Position in Course 2":cluster{dbl[], dbl[]})  [unwired: 1 in]
          }
        }
        n386 = Unbundle By Name(w149) -> ("upper limit"=w146:dbl, "upper limit"=w148:dbl)
        n387 = Multiply(x=w146, y=w147) -> ()  [unwired: 1 out]
        n388 = Multiply(x=w148, y=w147) -> ()  [unwired: 1 out]
        n389 = Round Toward -Infinity(1:w146) -> (0:w145:dbl)
        n390 = Subtract(x=w146, y=w145) -> (x-y=w144:dbl)
        n391 = Multiply(x=w144, y=12.0) -> (x*y=→"inches":dbl)
      }
    }
    n392 = case shown="True" w113 {
      tunnel: w112 -> [_ w120]
      frame False {
      }
      frame True {
        n393 = call "Tick Count3"() -> ("Tick Count(uSec)"=w121:u32)
        n394 = Subtract(x=w121, y=w120) -> (x-y=w124:u32)
        n395 = Divide(x=w124, y=u32 1000 ("x")) -> (x/y=→"dT":dbl)
      }
    }
    n396 = call "Tick Count6"() -> ("Tick Count(uSec)"=w110:u32)
    "Robot Coordinates\nHistory" <- w109
    "Orientation\nHistory" <- w114
    "Position Valid\nHistory" <- w115
  }
  n397 = disable-structure shown="Enabled" {
    disable-tunnel: [w862 _] -> _
    disable-tunnel: ["Search Step Size\n(deg)" _] -> _
    frame Enabled {
      n398 = Multiply(x=3.413333333333333, y="Search Step Size\n(deg)") -> (x*y=w860:dbl)
      n399 = To Unsigned Word Integer(number=w860) -> (unsigned 16bit integer=w862:u16)
    }
    frame Disabled {
    }
  }
  n400 = Multiply(x="Move Servo\nThreshold (deg)", y=3.413333333333333) -> (x*y=w18:dbl)
  n401 = To Unsigned Word Integer(number=w18) -> ()  [unwired: 1 out]
  n402 = flat-sequence {
    tunnel: [w866] -> w42
    tunnel: [w865] -> w41
    tunnel: [w870] -> w40
    tunnel: ["Left Servo\nID"] -> w29
    tunnel: ["Right Servo\nID"] -> w28
    tunnel: ["Compliance Slope"] -> w27
    tunnel: [w910] -> w39
    tunnel: [w909] -> w38
    tunnel: w42 -> [w908]
    tunnel: w41 -> [w907]
    tunnel: w40 -> [w906]
    tunnel: w29 -> [w904]
    tunnel: w28 -> [w903]
    tunnel: w27 -> [w902]
    tunnel: w39 -> [w1177]
    tunnel: w38 -> [w1176]
    frame #0 {
      # "BAUD RATE"
      # "Initialize UART and DIO"
      n403 = call-poly "VISA Configure Serial Port"("VISA resource name"=refnum<visa-resource-name> "ASRL1::INSTR", "Enable Termination\nChar (T)"=FALSE ("Enable Termination\nChar (T)"), "baud rate (9600)"=u32 115200) -> ("VISA resource name out"=w866:refnum<visa-resource-name>)  [unwired: 11 in, 1 out]
      n404 = call <vilib>:"Smart Open.vi"("Channel Names"=tag[] ["A/DIO2"]) -> ("DIO Ref Out"=w865:T9)  [unwired: 9 in, 1 out]
      n405 = flat-sequence {
        tunnel: w866 -> [w878]
        tunnel: w865 -> [w877]
        tunnel: "Left Servo\nID" -> [w879]
        tunnel: [w876] -> w867
        tunnel: "Compliance Slope" -> [w875]
        tunnel: "Right Servo\nID" -> [w892]
        tunnel: w867 -> [w891]
        tunnel: "Compliance Slope" -> [w890]
        tunnel: w866 -> [w889]
        tunnel: w865 -> [w888]
        frame #0 {
          w876 = 3
          n406 = while {
            tunnel: w876 -> [w885]
            tunnel: w878 -> [w883]
            tunnel: w877 -> [w882]
            tunnel: w879 -> [w881]
            tunnel: w875 -> [w880]
            i -> [w886]
            stop <- w884 stop-if-true
            n407 = call "Set_Compliance_Slope_R2.vi"("Compliance Slope"=w880, "DIO Ref Out"=w882, "VISA resource name"=w883, "Servo ID"=w881) -> ()  [unwired: 6 in, 2 out]
            n408 = Increment(x=w886) -> (x+1=w887:i32)
            n409 = Greater Or Equal?(x=w887, y=w885) -> (x >= y?=w884:bool)
          }
        }
        frame #1 {
          n410 = while {
            tunnel: w891 -> [w898]
            tunnel: w892 -> [w896]
            tunnel: w889 -> [w895]
            tunnel: w888 -> [w894]
            tunnel: w890 -> [w893]
            i -> [w899]
            stop <- w897 stop-if-true
            n411 = call "Set_Compliance_Slope_R2.vi"("Compliance Slope"=w893, "DIO Ref Out"=w894, "VISA resource name"=w895, "Servo ID"=w896) -> ()  [unwired: 6 in, 2 out]
            n412 = Increment(x=w899) -> (x+1=w900:i32)
            n413 = Greater Or Equal?(x=w900, y=w898) -> (x >= y?=w897:bool)
          }
        }
      }
      n414 = call "Tick Count"() -> ("Tick Count(uSec)"=w870:u32)
    }
    frame #1 {
      # "Service Count"
      n415 = while {
        shift-right: [w913] -> _
        shift-left: w906 -> [w930]
        tunnel: "Max Write\nTx Attempts" -> [w925]
        tunnel: "Max Read\nTx Attempts" -> [w924]
        shift-right: [w920] -> w910
        shift-left: w908 -> [w923]
        shift-right: [w919] -> w909
        shift-left: w907 -> [w922]
        tunnel: w904 -> [w918]
        tunnel: w903 -> [w917]
        tunnel: w902 -> [w916]
        shift-right: [w914] -> _
        shift-left: u16 0 -> [w915]
        stop <- "close comms" stop-if-true
        # "Loop Timer"
        n416 = local read "SERVO ENABLE"() -> (w912:bool)
        n417 = call "Tick Count2"() -> ("Tick Count(uSec)"=w913:u32)
        n418 = Subtract(x=w913, y=w930) -> (x-y=w929:u32)
        n419 = call "Wait4"("Count(mSec)"="Servo Comm\nLoop Time (ms)") -> ()  [unwired: 1 out]
        n420 = Divide(x=w929, y=u32 1000) -> (x/y=→"dT - Comm Loop":dbl)
        n421 = case shown="True" w912 {
          tunnel: w925 -> [_ w939]
          tunnel: w924 -> [_ w970]
          tunnel: w923 -> [w933 w934]
          tunnel: w922 -> [w932 w963]
          tunnel: [w933 w936] -> w920
          tunnel: [w932 w935] -> w919
          tunnel: w918 -> [_ w942]
          tunnel: w917 -> [_ w941]
          tunnel: w916 -> [_ w940]
          tunnel: w915 -> [_ w938]
          tunnel: [u16 100 w937] -> w914
          frame False {
            # "Restart at same value\nUsed to Periodically update \nCompliance Slope"
          }
          frame True {
            n422 = flat-sequence {
              tunnel: [w976] -> w974
              tunnel: [w977] -> w973
              tunnel: [w975] -> w972
              tunnel: w970 -> [w978]
              tunnel: [w980] -> w961
              tunnel: [w979] -> w959
              tunnel: w934 -> [w980]
              tunnel: w963 -> [w979]
              tunnel: w942 -> [w975]
              tunnel: w974 -> [w998]
              tunnel: w973 -> [w999]
              tunnel: w972 -> [w997]
              tunnel: [w997] -> w971
              tunnel: [w996] -> w964
              tunnel: [w995] -> w962
              tunnel: w961 -> [w995]
              tunnel: [w994] -> w960
              tunnel: w959 -> [w994]
              tunnel: w971 -> [w1017]
              tunnel: w939 -> [w1016]
              tunnel: w964 -> [w1011]
              tunnel: w962 -> [w1013]
              tunnel: w960 -> [w1012]
              tunnel: [w1013] -> w957
              tunnel: [w1012] -> w955
              tunnel: [w1050] -> w958
              tunnel: w957 -> [w1050]
              tunnel: [w1049] -> w956
              tunnel: w955 -> [w1049]
              tunnel: ["Servo Comm\nWait Time - (ms)"] -> w947
              tunnel: w970 -> [w1057]
              tunnel: [w1056] -> w969
              tunnel: [w1055] -> w968
              tunnel: [w1051] -> w966
              tunnel: w958 -> [w1054]
              tunnel: w956 -> [w1053]
              tunnel: [w1054] -> w954
              tunnel: [w1053] -> w951
              tunnel: [w1052] -> w948
              tunnel: w947 -> [w1052]
              tunnel: w941 -> [w1051]
              tunnel: w969 -> [w1077]
              tunnel: w968 -> [w1076]
              tunnel: [w1075] -> w967
              tunnel: w966 -> [w1075]
              tunnel: [w1074] -> w965
              tunnel: w954 -> [w1073]
              tunnel: [w1073] -> w953
              tunnel: [w1072] -> w952
              tunnel: w951 -> [w1072]
              tunnel: w948 -> [w1071]
              tunnel: [w1071] -> w946
              tunnel: w967 -> [w1096]
              tunnel: w965 -> [w1094]
              tunnel: w939 -> [w1095]
              tunnel: w953 -> [w1093]
              tunnel: w952 -> [w1092]
              tunnel: [w1093] -> w950
              tunnel: [w1092] -> w949
              tunnel: w946 -> [w1089]
              tunnel: [w1089] -> w945
              tunnel: w950 -> [w1129]
              tunnel: w949 -> [w1128]
              tunnel: w945 -> [w1127]
              tunnel: [w1129] -> w944
              tunnel: [w1128] -> w943
              tunnel: w944 -> [w1133]
              tunnel: w943 -> [w1132]
              tunnel: w942 -> [w1138]
              tunnel: w941 -> [w1137]
              tunnel: w940 -> [w1136]
              tunnel: w938 -> [w1131]
              tunnel: w939 -> [w1135]
              tunnel: [w1134] -> w937
              tunnel: [w1133] -> w936
              tunnel: [w1132] -> w935
              frame #0 {
                n423 = while {
                  tunnel: [w993] -> w976
                  tunnel: w975 -> [w992]
                  tunnel: [w985] -> w977
                  tunnel: w978 -> [w983]
                  tunnel: w980 -> [w982]
                  tunnel: w979 -> [w981]
                  i -> [w984]
                  stop <- w986 stop-if-true
                  # "Attemp to Read Until\nMax Read Tx Attemps Limit"
                  n424 = call "ReadServo_R3.vi"("DIO Ref In"=w981, "VISA resource name out"=w982, "Servo ID"=w992) -> ("Error"=w989:u8, "Valid Checksum"=w990:bool, "Current Position"=w993:u64)  [unwired: 6 in]
                  n425 = Increment(x=w984) -> (x+1=w987:i32)
                  n426 = Equal To 0?(x=w989) -> (x = 0?=w991:bool)
                  n427 = Greater Or Equal?(x=w987, y=w983) -> (x >= y?=w988:bool)
                  n428 = And(x=w990, y=w991) -> (x .and. y?=w985:bool)
                  n429 = Or(x=w985, y=w988) -> (x .or. y?=w986:bool)
                }
              }
              frame #1 {
                # "Read Position First"
                n430 = local read "Servo Goal Position\n - Left"() -> (w996:u16)
                n431 = case shown="True" w999 {
                  tunnel: w998 -> [_ w1001]
                  tunnel: w996 -> [_ w1005]
                  frame False {
                  }
                  frame True {
                    # "Convert Received Position to Angle Relative to Robot"
                    n432 = local write "Current L (10bit)"(w1001) -> ()
                    n433 = local read "Mounting Offset - Left"() -> (w1003:sgl)
                    n434 = To Word Integer(number=w1001) -> (16bit integer=w1010:i16)
                    n435 = To Word Integer(number=w1005) -> (16bit integer=w1009:i16)
                    n436 = Subtract(x=w1009, y=w1010) -> (x-y=w1008:i16)
                    n437 = Absolute Value(x=w1008) -> (abs(x)=w1007:i16)
                    n438 = call "Servo_GP_Angle_Conversion_R0.vi"("GP in"=w1001, "Mode Select"=0, "Mount Offset"=w1003) -> ("Angle Out"=w1000:sgl)  [unwired: 7 in, 1 out]
                    n439 = Greater?(x=w1007, y=u16 5) -> (0:w1004:bool)
                    n440 = local write "Servo Moving - L"(w1004) -> ()
                    n441 = local write "Move Servo - L"(w1004) -> ()
                    n442 = local write "Current Angle\n - Left (internal)"(w1000) -> ()
                    n443 = shared-variable "RT myRIO Target - Overlord\\Localization_Variables_r0.lvlib\\Left Servo Angle_Current"(w1000) -> ()  [unwired: 1 in, 1 out]
                  }
                }
              }
              frame #2 {
                n444 = local read "Move Servo - L"() -> (w1014:bool)
                n445 = case shown="True" w1014 {
                  tunnel: w1017 -> [_ w1032]
                  tunnel: w1011 -> [_ w1019]
                  tunnel: [TRUE w1030] -> w1015
                  tunnel: w1016 -> [_ w1022]
                  tunnel: w1013 -> [_ w1021]
                  tunnel: w1012 -> [_ w1020]
                  frame False {
                    # "Only Send if Current Position is far enough"
                  }
                  frame True {
                    w1028 = 1
                    # "High Byte"
                    # "Low Byte"
                    n446 = Type Cast(type="", x=w1019) -> (*(type *) &x=w1029:string)
                    n447 = local write "Servo Moving - L"(TRUE) -> ()
                    n448 = String Subset(string=w1029, offset (0)=1, length (rest)=w1028) -> (substring=w1024:string)
                    n449 = String Subset(string=w1029, offset (0)=0, length (rest)=w1028) -> (substring=w1023:string)
                    n450 = while {
                      tunnel: w1032 -> [w1046]
                      tunnel: [w1038] -> w1030
                      tunnel: w1024 -> [w1042]
                      tunnel: w1023 -> [w1041]
                      tunnel: w1022 -> [w1035]
                      tunnel: w1021 -> [w1034]
                      tunnel: w1020 -> [w1033]
                      i -> [w1036]
                      stop <- w1037 stop-if-true
                      # "Attemp to Write Until\nMax Write Tx Attemps Limit"
                      n451 = call "MoveServo_R3.vi"("DIO Ref Out"=w1033, "VISA resource name out"=w1034, "GP - Low Byte"=w1042, "GP - High Byte"=w1041, "Servo ID"=w1046) -> ("Valid Checksum"=w1043:bool, "Error"=w1045:u64)  [unwired: 5 in]
                      n452 = Equal To 0?(x=w1045) -> (x = 0?=w1044:bool)
                      n453 = And(x=w1043, y=w1044) -> (x .and. y?=w1038:bool)
                      n454 = Increment(x=w1036) -> (x+1=w1040:i32)
                      n455 = Greater Or Equal?(x=w1040, y=w1035) -> (x >= y?=w1039:bool)
                      n456 = Or(x=w1038, y=w1039) -> (x .or. y?=w1037:bool)
                    }
                  }
                }
                n457 = case shown="True" w1015 {
                  frame False {
                  }
                  frame True {
                    # "Update Servo flag"
                    n458 = local write "Move Servo - L"(FALSE) -> ()
                  }
                }
              }
              frame #3 {
                n459 = call "Wait2"("Count(mSec)"="Servo Comm\nWait Time - (ms)") -> ()  [unwired: 1 out]
              }
              frame #4 {
                n460 = while {
                  tunnel: [w1070] -> w1056
                  tunnel: w1051 -> [w1069]
                  tunnel: [w1062] -> w1055
                  tunnel: w1057 -> [w1060]
                  tunnel: w1054 -> [w1059]
                  tunnel: w1053 -> [w1058]
                  i -> [w1061]
                  stop <- w1063 stop-if-true
                  # "Attemp to Read Until\nMax Read Tx Attemps Limit"
                  n461 = call "ReadServo_R3.vi"("DIO Ref In"=w1058, "VISA resource name out"=w1059, "Servo ID"=w1069) -> ("Error"=w1066:u8, "Valid Checksum"=w1067:bool, "Current Position"=w1070:u64)  [unwired: 6 in]
                  n462 = Increment(x=w1061) -> (x+1=w1064:i32)
                  n463 = Equal To 0?(x=w1066) -> (x = 0?=w1068:bool)
                  n464 = Greater Or Equal?(x=w1064, y=w1060) -> (x >= y?=w1065:bool)
                  n465 = And(x=w1067, y=w1068) -> (x .and. y?=w1062:bool)
                  n466 = Or(x=w1062, y=w1065) -> (x .or. y?=w1063:bool)
                }
              }
              frame #5 {
                n467 = local read "Servo Goal Position\n - Right"() -> (w1074:u16)
                n468 = case shown="True" w1076 {
                  tunnel: w1077 -> [_ w1079]
                  tunnel: w1074 -> [_ w1083]
                  frame False {
                    # "Don't update current position"
                  }
                  frame True {
                    # "Convert Received Position to Angle Relative to Robot"
                    n469 = local read "Mounting Offset - Right"() -> (w1081:sgl)
                    n470 = local write "Current R (10bit)"(w1079) -> ()
                    n471 = call "Servo_GP_Angle_Conversion_R0.vi"("GP in"=w1079, "Mode Select"=0, "Mount Offset"=w1081) -> ("Angle Out"=w1078:sgl)  [unwired: 7 in, 1 out]
                    n472 = To Word Integer(number=w1083) -> (16bit integer=w1087:i16)
                    n473 = local write "Current Angle\n - Right (internal)"(w1078) -> ()
                    n474 = To Word Integer(number=w1079) -> (16bit integer=w1088:i16)
                    n475 = shared-variable "RT myRIO Target - Overlord\\Localization_Variables_r0.lvlib\\Right Servo Angle_Current"(w1078) -> ()  [unwired: 1 in, 1 out]
                    n476 = Subtract(x=w1087, y=w1088) -> (x-y=w1086:i16)
                    n477 = Absolute Value(x=w1086) -> (abs(x)=w1085:i16)
                    n478 = Greater?(x=w1085, y=u16 5) -> (0:w1082:bool)
                    n479 = local write "Servo Moving - R"(w1082) -> ()
                    n480 = local write "Move Servo - R"(w1082) -> ()
                  }
                }
              }
              frame #6 {
                n481 = local read "Move Servo - R"() -> (w1090:bool)
                n482 = case shown="True" w1090 {
                  tunnel: w1094 -> [_ w1099]
                  tunnel: w1096 -> [_ w1106]
                  tunnel: [TRUE w1107] -> w1091
                  tunnel: w1095 -> [_ w1102]
                  tunnel: w1093 -> [_ w1101]
                  tunnel: w1092 -> [_ w1100]
                  frame False {
                  }
                  frame True {
                    w1109 = 1
                    # "High Byte"
                    # "Low Byte"
                    n483 = Type Cast(type="", x=w1099) -> (*(type *) &x=w1108:string)
                    n484 = local write "Servo Moving - R"(TRUE) -> ()
                    n485 = String Subset(string=w1108, offset (0)=1, length (rest)=w1109) -> (substring=w1105:string)
                    n486 = String Subset(string=w1108, offset (0)=0, length (rest)=w1109) -> (substring=w1104:string)
                    n487 = while {
                      tunnel: [w1118] -> w1107
                      tunnel: w1106 -> [w1123]
                      tunnel: w1105 -> [w1122]
                      tunnel: w1104 -> [w1121]
                      tunnel: w1102 -> [w1116]
                      tunnel: w1101 -> [w1114]
                      tunnel: w1100 -> [w1113]
                      i -> [w1117]
                      stop <- w1115 stop-if-true
                      # "Attemp to Write Until\nMax Write Tx Attemps Limit"
                      n488 = call "MoveServo_R3.vi"("DIO Ref Out"=w1113, "VISA resource name out"=w1114, "GP - Low Byte"=w1122, "GP - High Byte"=w1121, "Servo ID"=w1123) -> ("Valid Checksum"=w1125:bool, "Error"=w1124:u64)  [unwired: 5 in]
                      n489 = Increment(x=w1117) -> (x+1=w1119:i32)
                      n490 = Greater Or Equal?(x=w1119, y=w1116) -> (x >= y?=w1120:bool)
                      n491 = Equal To 0?(x=w1124) -> (x = 0?=w1126:bool)
                      n492 = And(x=w1125, y=w1126) -> (x .and. y?=w1118:bool)
                      n493 = Or(x=w1118, y=w1120) -> (x .or. y?=w1115:bool)
                    }
                  }
                }
                n494 = case shown="True" w1091 {
                  frame False {
                  }
                  frame True {
                    # "Update Servo flag"
                    n495 = local write "Move Servo - R"(FALSE) -> ()
                  }
                }
              }
              frame #7 {
                n496 = call "Wait3"("Count(mSec)"=w1127) -> ()  [unwired: 1 out]
              }
              frame #8 {
                # "Increment Service Count"
                # "Update Compliance Slope\nEvery x loops"
                n497 = Equal?(x=w1131, y=u16 1000) -> (x = y?=w1140:bool)
                n498 = case shown="True" w1140 {
                  tunnel: w1136 -> [_ w1150]
                  tunnel: w1133 -> [_ w1149]
                  tunnel: w1132 -> [_ w1148]
                  tunnel: w1133 -> [_ w1147]
                  tunnel: w1132 -> [_ w1146]
                  tunnel: w1138 -> [_ w1145]
                  tunnel: w1137 -> [_ w1144]
                  tunnel: w1131 -> [w1141 _]
                  tunnel: [w1141 u16 0] -> w1139
                  tunnel: w1135 -> [_ w1142]
                  frame False {
                  }
                  frame True {
                    # "Reset Service\nCount"
                    n499 = flat-sequence {
                      tunnel: w1149 -> [w1155]
                      tunnel: w1148 -> [w1154]
                      tunnel: w1145 -> [w1156]
                      tunnel: [w1152] -> w1151
                      tunnel: w1150 -> [w1153]
                      tunnel: w1142 -> [w1152]
                      tunnel: w1144 -> [w1168]
                      tunnel: w1151 -> [w1167]
                      tunnel: w1150 -> [w1166]
                      tunnel: w1147 -> [w1165]
                      tunnel: w1146 -> [w1164]
                      frame #0 {
                        n500 = while {
                          tunnel: w1152 -> [w1163]
                          tunnel: w1155 -> [w1161]
                          tunnel: w1154 -> [w1160]
                          tunnel: w1156 -> [w1159]
                          tunnel: w1153 -> [w1158]
                          i -> [w1157]
                          stop <- w1162 stop-if-true
                          n501 = call "Set_Compliance_Slope_R2.vi"("Compliance Slope"=w1158, "DIO Ref Out"=w1160, "VISA resource name"=w1161, "Servo ID"=w1159) -> ()  [unwired: 6 in, 2 out]
                          n502 = Greater Or Equal?(x=w1157, y=w1163) -> (x >= y?=w1162:bool)
                        }
                      }
                      frame #1 {
                        n503 = while {
                          tunnel: w1167 -> [w1175]
                          tunnel: w1168 -> [w1173]
                          tunnel: w1165 -> [w1172]
                          tunnel: w1164 -> [w1171]
                          tunnel: w1166 -> [w1170]
                          i -> [w1169]
                          stop <- w1174 stop-if-true
                          n504 = call "Set_Compliance_Slope_R2.vi"("Compliance Slope"=w1170, "DIO Ref Out"=w1171, "VISA resource name"=w1172, "Servo ID"=w1173) -> ()  [unwired: 6 in, 2 out]
                          n505 = Greater Or Equal?(x=w1169, y=w1175) -> (x >= y?=w1174:bool)
                        }
                      }
                    }
                  }
                }
                n506 = Increment(x=w1139) -> (x+1=w1134:u16)
              }
            }
          }
        }
      }
    }
    frame #2 {
      n507 = VISA Close(VISA resource name=w1177) -> ()  [unwired: 1 in, 1 out]
      n508 = call <vilib>:"Close.vi"("DIO Ref In"=w1176) -> ()  [unwired: 10 in, 1 out]
    }
  }
  n509 = while {
    stop <- FALSE stop-if-true
    n510 = call "Wait9"("Count(mSec)"=u32 1000) -> ()  [unwired: 1 out]
  }
  n511 = while {
    shift-right: [w1248] -> _
    shift-left: "Initial Main State - Left" -> [w1270]
    shift-right: [w1240] -> _
    shift-left: "Search Direction - in - L" -> [w1264]
    shift-right: [w1239] -> _
    shift-left: FALSE -> [w1263]
    shift-right: [w1242] -> _
    shift-left: w13 -> [w1241]
    shift-right: [w1243] -> _
    shift-left: w13 -> [w1257]
    shift-right: [w1244] -> _
    shift-left: w13 -> [w1262]
    shift-right: [w1245] -> _
    shift-left: w13 -> [w1256]
    shift-right: [w1246] -> _
    shift-left: w13 -> [w1255]
    shift-right: [w1192] -> _
    shift-left: "Search Direction - in - Right" -> [w1205]
    shift-right: [w1236] -> _
    shift-left: FALSE -> [w1203]
    shift-right: [w1237] -> _
    shift-left: w12 -> [w1194]
    shift-right: [w1191] -> _
    shift-left: w12 -> [w1193]
    shift-right: [w1190] -> _
    shift-left: w12 -> [w1200]
    shift-right: [w1189] -> _
    shift-left: w12 -> [w1202]
    shift-right: [w1188] -> _
    shift-left: w12 -> [w1201]
    shift-right: [w1180] -> _
    shift-left: "Initial Main State- Right" -> [w1217]
    shift-right: [w1232] -> _
    shift-left: 0 -> [w1234]
    shift-right: [w1184] -> _
    shift-left: 0 -> [w1209]
    shift-right: [w1231] -> _
    shift-left: "Initial Tracking State - Left" -> [w1233]
    shift-right: [w1186] -> _
    shift-left: "Initial Tracking State - Right" -> [w1215]
    shift-right: [w1185] -> _
    shift-left: "Initial Recovery State  - Right" -> [w1216]
    shift-right: [w1229] -> _
    shift-left: "Initial Recovery State - L" -> [w1230]
    stop <- FALSE stop-if-true
    w1224 = enum16{"Track", "Reactive Predict", ""}."Track" ("Initial Tracking State - Right")
    w1250 = T5."Tracking" ("Next Main State")
    # "Wait for New"
    # "ADD TRACKING TIMEOUT COUNT**********************"
    # "Service Track Angle Flag"
    # "Add Logic to Have Search Directions\nopposite if Both Searching"
    # "REMOVE LAST GOAL POSITION WITH cURRENT"
    # "Go to Current State"
    # "Add Logic to Have Search Directions\nopposite if Both Searching"
    # "Manuallly Reset\nRespond Var"
    # "Manuallly Reset\nRespond Var"
    # "Update Comm Process Variables"
    # "Both  inTracking (main state)"
    # "Current delta - L"
    # "delta move sum - R"
    # "delta move sum - L"
    # "Current delta - R"
    # "Service Move Respond Variables"
    n512 = local read "Min Num Frames\nper Search"() -> (w1238:i32)
    n513 = local read "Minimum Delta \nServo Threshold"() -> (w1254:i16)
    n514 = local read "Maximum Move \nServo Threshold"() -> (w1253:i16)
    n515 = local read "Middle Beacon\nCoordinates"() -> (w1195:cluster{"X":sgl, "Y":sgl})
    n516 = local read "Position \nLock Status"() -> (w1261:bool)
    n517 = local read "Position \nLock Status"() -> (w1198:bool)
    n518 = local read "Search Step Size"() -> (w1252:u16)
    n519 = local read "Last Orientation"() -> (w1259:sgl)
    n520 = local read "Last Orientation"() -> (w1196:sgl)
    n521 = local read "Last Position"() -> (w1260:cluster{"X":sgl, "Y":sgl})
    n522 = local read "Last Position"() -> (w1197:cluster{"X":sgl, "Y":sgl})
    n523 = local read "Min Num Frames\nper Search"() -> (w1199:i32)
    n524 = call "Wait"("Count(mSec)"="Servo Algorithm\nCycle Time(ms)") -> ()  [unwired: 1 out]
    n525 = local read "Minimum Delta \nServo Threshold"() -> (w1207:i16)
    n526 = local read "Maximum Move \nServo Threshold"() -> (w1206:i16)
    n527 = local read "Search Step Size"() -> (w1204:u16)
    n528 = local read "New Data  Flag\nRight Servo"() -> (w1212:bool)
    n529 = local read "New Data  Flag\nLeft Servo"() -> (w1228:bool)
    n530 = local read "Image Lock - Right"() -> (w1214:bool)
    n531 = local read "Tracking Angle - Right"() -> (w1211:sgl)
    n532 = local read "Image Lock - Left"() -> (w1269:bool)
    n533 = local read "Tracking Angle - Left"() -> (w1267:sgl)
    n534 = local read "Current R (10bit)"() -> (w1210:u16)
    n535 = local read "Current L (10bit)"() -> (w1266:u16)
    n536 = case shown="True" w1228 {
      tunnel: [w1782 w1820] -> w1272
      tunnel: [w1776 w1819] -> w1271
      tunnel: w1270 -> [w1777 w1818]
      tunnel: w1269 -> [_ w1817]
      tunnel: "Track Angle Valid - Left" -> [_ w1816]
      tunnel: w1267 -> [_ w1815]
      tunnel: w1266 -> [w1782 w1814]
      tunnel: "Mounting Offset - Left" -> [_ w1813]
      tunnel: w1264 -> [w1773 w1812]
      tunnel: w1263 -> [_ w1811]
      tunnel: w1262 -> [w1774 w1810]
      tunnel: w1261 -> [_ w1809]
      tunnel: w1260 -> [_ w1808]
      tunnel: w1259 -> [_ w1807]
      tunnel: "Middle Beacon\nCoordinates" -> [_ w1806]
      tunnel: w1257 -> [w1772 w1805]
      tunnel: w1256 -> [w1771 w1804]
      tunnel: w1255 -> [w1775 w1803]
      tunnel: w1254 -> [_ w1802]
      tunnel: w1253 -> [_ w1801]
      tunnel: w1252 -> [_ w1800]
      tunnel: [0 w1799] -> w1249
      tunnel: [w1777 w1798] -> w1248
      tunnel: [w1776 w1797] -> w1247
      tunnel: [w1775 w1796] -> w1246
      tunnel: [w1771 w1795] -> w1245
      tunnel: [w1774 w1794] -> w1244
      tunnel: [w1772 w1793] -> w1243
      tunnel: w1241 -> [_ w1792]
      tunnel: [w1773 w1791] -> w1240
      tunnel: w1238 -> [_ w1790]
      tunnel: w1234 -> [w1780 w1789]
      tunnel: w1233 -> [w1779 w1788]
      tunnel: [w1780 w1787] -> w1232
      tunnel: [w1779 w1786] -> w1231
      tunnel: w1230 -> [w1778 w1785]
      tunnel: [w1778 w1784] -> w1229
      frame False {
        w1776 = FALSE
        # "Recovery Mode COunt"
        # "Frames Processed - L"
        # "Recovery Search move Count - L"
        # "Recovery Search Attempt Count- L"
        # "WAITING FOR NEW IMAGE, RETAIN ALL VALUES"
      }
      frame True {
        w1822 = u16 1023
        w1825 = u16 0
        # "New Tracking State"
        # "Tracking Timeout Count"
        # "Next Main State"
        # "Next Recovery State"
        # "Reset Respond"
        # "Search Direction"
        # "Recovery Count"
        # "Recovery Search move Count"
        # "Recovery Search Attempt Count"
        # "Frames Processed"
        # "Apply Floor/Ceiling to Goal Position"
        # "Current move Delta"
        # "Service Track Angle Flag"
        # "Move Servo"
        # "Goal Position"
        # "Go to Current State"
        n537 = case shown="\"Start Up Search\", Default" w1818 {
          tunnel: w1814 -> [w1843 w1882 w2050]
          tunnel: w1815 -> [_ w1884 _]
          tunnel: w1800 -> [w1842 _ w2045]
          tunnel: w1812 -> [w1841 w1865 w2039]
          tunnel: [w1840 w1880 w2049] -> w1826
          tunnel: [w1838 w1881 w2048] -> w1819
          tunnel: w1816 -> [_ w1875 w2026]
          tunnel: [w1836 w1877 w2035] -> w1798
          tunnel: w1817 -> [w1827 w1876 w2024]
          tunnel: w1813 -> [_ w1885 w2046]
          tunnel: w1802 -> [_ w1883 _]
          tunnel: [w1830 w1879 w2030] -> w1799
          tunnel: w1801 -> [_ w1878 _]
          tunnel: w1810 -> [w1835 _ w2040]
          tunnel: [enum16{"Generic Sweep", "Recovery Search"}."Recovery Search" enum16{"Generic Sweep", "Recovery Search"}."Recovery Search" w2047] -> w1784
          tunnel: w1805 -> [_ _ w2044]
          tunnel: w1785 -> [_ _ w2027]
          tunnel: w1811 -> [_ w1862 w2056]
          tunnel: w1792 -> [_ w1858 w2051]
          tunnel: w1807 -> [_ w1868 w2053]
          tunnel: w1808 -> [_ w1869 w2054]
          tunnel: w1809 -> [_ w1870 w2055]
          tunnel: w1806 -> [_ w1867 w2052]
          tunnel: [FALSE w1864 w2028] -> w1797
          tunnel: w1790 -> [w1834 _ w2038]
          tunnel: [w1830 w1859 w2037] -> w1793
          tunnel: [w1830 w1859 w2043] -> w1796
          tunnel: [w1830 w1859 w2042] -> w1795
          tunnel: [w1833 w1860 w2041] -> w1794
          tunnel: w1804 -> [_ _ w2033]
          tunnel: w1803 -> [_ _ w2032]
          tunnel: [w1831 w1865 w2031] -> w1791
          tunnel: w1789 -> [_ w1874 _]
          tunnel: [w1830 w1866 w2030] -> w1787
          tunnel: w1788 -> [_ w1871 _]
          tunnel: [enum16{"Track", "Reactive Predict", ""}."Track" ("Initial Tracking State - Right") w1863 enum16{"Track", "Reactive Predict", ""}."Track" ("Initial Tracking State - Right")] -> w1786
          frame "Start Up Search", Default {
            w1830 = u16 0
            # "ONly Exit Startup\nafter we've rotated to correct orientation"
            # "Image Lock"
            # "Search Direction"
            # "Wait for 'x' Images to be Processed\nBefore Going to Next Step"
            # "Next Main State"
            # "New Goal Position"
            # "Move Servo"
            # "Choose Next State"
            # "Frames Processed Count"
            n538 = Greater Or Equal?(x=w1835, y=w1834) -> (x >= y?=w1839:bool)
            n539 = case shown="True" w1839 {
              tunnel: w1843 -> [w1853 _]
              tunnel: w1842 -> [_ _]
              tunnel: w1841 -> [w1852 _]
              tunnel: [w1853 _] -> w1840
              tunnel: [w1851 0] -> w1833
              tunnel: [FALSE TRUE] -> w1837
              tunnel: w1835 -> [w1854 _]
              tunnel: [w1852 _] -> w1831
              frame False {
                # "Wait until Min Number of Frames (per search/step) Processed"
                # "Increase Frames\nProcessed Count"
                n540 = Increment(x=w1854) -> (x+1=w1851:i32)
              }
              frame True {
                # "Reset Frames\nProcessed Count"
                # "Nearest step"
                n541 = case shown="True" {
                  selector: _ -> [_ _]
                  frame False {
                  }
                  frame True {
                  }
                }
              }
            }
            n542 = case shown="False" w1827 {
              tunnel: [w1845 FALSE] -> w1838
              tunnel: w1837 -> [w1845 _]
              tunnel: [w1846 T5."Tracking" ("Next Main State")] -> w1836
              frame False {
                # "Check other Servo\nStay in Startup  State"
                n543 = local read "Image Lock - Right"() -> (w1844:bool)
                n544 = case shown="False" w1844 {
                  tunnel: [T5."Start Up Search" ("Next Main State") T5."Recovery Mode" ("Next Main State")] -> w1846
                  frame False {
                  }
                  frame True {
                  }
                }
              }
              frame True {
                # "Override Move Servo\nCommand bc an Angle Was Found\nduring this Step"
                # "Transition to Tracking State When\nImage Processing has Locked"
              }
            }
          }
          frame "Tracking" {
            w1859 = 0
            # "Frames Processed Count"
            # "Image Lock - L"
            # "Track Angle Valid"
            # "Tracking Angle"
            # "Tracking Timeout Count"
            # "Max ove delta"
            # "Move delta threshold"
            # "mount offset"
            # "Current Position"
            # "Move Respond"
            # "Trackin Timeout count"
            # "Move Servo"
            # "delta"
            # "GP"
            # "Reset Move Respond"
            # "New Tracking State"
            # "Delta Move Sum"
            # "Choose Next State"
            n545 = case shown="\"Track\", Default" w1871 {
              tunnel: w1885 -> [w1903 _]
              tunnel: w1884 -> [w1902 _]
              tunnel: w1883 -> [w1901 _]
              tunnel: w1882 -> [w1900 w1948]
              tunnel: [w1899 w1946] -> w1881
              tunnel: [w1898 w1954] -> w1880
              tunnel: [w1897 0] -> w1879
              tunnel: w1878 -> [w1896 _]
              tunnel: w1876 -> [w1895 w1938]
              tunnel: w1875 -> [w1894 w1941]
              tunnel: w1874 -> [w1893 w1943]
              tunnel: w1870 -> [_ w1953]
              tunnel: w1869 -> [_ w1952]
              tunnel: w1868 -> [_ w1951]
              tunnel: w1867 -> [_ w1950]
              tunnel: w1862 -> [_ w1949]
              tunnel: w1858 -> [_ w1947]
              tunnel: [TRUE w1944] -> w1864
              tunnel: [w1890 w1942] -> w1866
              tunnel: [w1888 w1940] -> w1863
              tunnel: [0 0] -> w1860
              frame "Track", Default {
                # "Reset"
                # "Tracking Timeout"
                # "Move Delta"
                # "Goal Position"
                # "Tracking Move"
                # "Move Servo"
                # "Only Consider Tracking Angle\n\nIF\n\nImage Locked        == T\nTrack Angle Flag   == T"
                n546 = And(x=w1895, y=w1894) -> (x .and. y?=w1887:bool)
                n547 = case shown="True" w1887 {
                  tunnel: w1903 -> [_ w1911]
                  tunnel: w1902 -> [_ w1909]
                  tunnel: w1901 -> [_ w1926]
                  tunnel: w1900 -> [w1906 w1916]
                  tunnel: [w1906 w1925] -> w1898
                  tunnel: [w1908 w1924] -> w1899
                  tunnel: [w1908 w1923] -> _
                  tunnel: [u16 0 w1922] -> w1897
                  tunnel: w1896 -> [_ w1918]
                  tunnel: w1893 -> [w1905 _]
                  tunnel: [w1904 0] -> w1890
                  frame False {
                    w1908 = FALSE
                    # "Increment timeout"
                    n548 = Increment(x=w1905) -> (x+1=w1904:i32)
                  }
                  frame True {
                    # "******"
                    # "Move to Tracking Angle \n\nif delta is greater than move servo threshold\nAND less than max move threshold"
                    n549 = call "Servo_GP_Angle_Conversion_R0.vi"("Angle In"=w1909, "Mode Select"=1, "Mount Offset"=w1911) -> ("GP out"=w1910:u16)  [unwired: 7 in, 1 out]
                    n550 = To Word Integer(number=w1916) -> (16bit integer=w1914:i16)
                    n551 = To Word Integer(number=w1910) -> (16bit integer=w1927:i16)
                    n552 = Subtract(x=w1927, y=w1914) -> (x-y=w1917:i16)
                    n553 = Absolute Value(x=w1917) -> (abs(x)=w1913:i16)
                    n554 = Greater Or Equal?(x=w1913, y=w1926) -> (x >= y?=w1920:bool)
                    n555 = Less Or Equal?(x=w1913, y=w1918) -> (x <= y?=w1919:bool)
                    n556 = And(x=w1920, y=w1919) -> (x .and. y?=w1921:bool)
                    n557 = case shown="True" w1921 {
                      tunnel: w1910 -> [_ w1932]
                      tunnel: [w1929 w1932] -> w1925
                      tunnel: [w1930 w1934] -> w1924
                      tunnel: [w1930 w1934] -> w1923
                      tunnel: w1916 -> [w1929 _]
                      tunnel: w1913 -> [_ w1933]
                      tunnel: [u16 0 w1933] -> w1922
                      tunnel: w1909 -> [_ w1931]
                      frame False {
                        w1930 = FALSE
                        # "Don't Move"
                      }
                      frame True {
                        w1934 = TRUE
                        # "1024/300"
                        # "Current Delta"
                        # "Use new Track Angle"
                        n558 = local write "Last Track Angle - L"(w1931) -> ()
                      }
                    }
                  }
                }
                n559 = local read "Timeout to \nEnable Reactive Predict"() -> (w1891:u16)
                n560 = Less?(x=w1890, y=w1891) -> (x < y?=w1889:bool)
                n561 = case shown="True" w1889 {
                  tunnel: [enum16{"Track", "Reactive Predict", ""}."Reactive Predict" ("Initial Tracking State - Right") enum16{"Track", "Reactive Predict", ""}."Track" ("Initial Tracking State - Right")] -> w1888
                  frame False {
                  }
                  frame True {
                  }
                }
              }
              frame "Reactive Predict" {
                # "Choose New\nTracking State"
                n562 = Or(x=w1938, y=w1941) -> (x .or. y?=w1937:bool)
                n563 = case shown="False" w1937 {
                  tunnel: [w1967 w2020] -> w1954
                  tunnel: w1953 -> [w1966 _]
                  tunnel: w1952 -> [w1965 _]
                  tunnel: w1951 -> [w1964 _]
                  tunnel: w1950 -> [w1963 _]
                  tunnel: w1949 -> [w1962 _]
                  tunnel: w1947 -> [w1961 _]
                  tunnel: [w1960 FALSE] -> w1946
                  tunnel: [w1959 TRUE] -> w1944
                  tunnel: w1943 -> [w1958 _]
                  tunnel: [w1957 0] -> w1942
                  tunnel: [enum16{"Track", "Reactive Predict", ""}."Reactive Predict" ("Initial Tracking State - Right") enum16{"Track", "Reactive Predict", ""}."Track" ("Initial Tracking State - Right")] -> w1940
                  tunnel: w1948 -> [w1955 w2020]
                  frame False {
                    # "Stay in Reactive State"
                    # "Increment Track Timeout"
                    # "Move Respond Flag"
                    n564 = Increment(x=w1958) -> (x+1=w1957:i32)
                    n565 = case shown="True" w1962 {
                      tunnel: w1966 -> [_ w1982]
                      tunnel: w1965 -> [_ w1981]
                      tunnel: w1964 -> [_ w1980]
                      tunnel: w1963 -> [_ w1979]
                      tunnel: w1961 -> [_ w1976]
                      tunnel: [w1968 w1972] -> w1967
                      tunnel: [w1969 w1971] -> w1960
                      tunnel: [w1969 w1971] -> w1959
                      tunnel: w1955 -> [w1968 w1970]
                      frame False {
                        w1969 = FALSE
                        # "Reset Move Respond = F"
                        # "Move Servo = F"
                      }
                      frame True {
                        w1971 = TRUE
                        # "Position Lock"
                        # "Current Servo\nPosition"
                        # "Reset Move\nRespond = T"
                        # "Move Servo = T"
                        # "Apply Direction \nto Offset (delta sum)"
                        # "Check Last Known Position of Robot"
                        n566 = case shown="True" w1982 {
                          tunnel: w1981 -> [_ w2010]
                          tunnel: w1980 -> [_ w1985]
                          tunnel: w1979 -> [_ w1986]
                          tunnel: [sgl 1.0 ("y") w1984] -> w1978
                          frame False {
                            # "No Position Data Available"
                            # "Default is to move\nSame Direction as other\nServo"
                          }
                          frame True {
                            w1991 = sgl 1.0 ("y")
                            # "Use previous position/orientation to Guess Which Direction to Move Servo"
                            # "Choose Search Direction"
                            # "\"Perpendicular \nThreshold\""
                            # "If Orientation is\n ~Perpendicular -> Start Search\n in Opposite Direction of Other"
                            # "****add 90 until orientation angle is fixed"
                            # "Last Orientation"
                            # "Convert to Rad"
                            # "Avoid Divide by 0"
                            # "-1/m"
                            # "Calculate Normal Line to \nLast Robot Position\nfrom Center Beacon"
                            # "last Position \nCoordinates"
                            n567 = Unbundle(w2010) -> ("X"=w1990:sgl, "Y"=w1989:sgl)
                            n568 = Unbundle(w1986) -> ("X"=w1988:sgl, "Y"=w1987:sgl)
                            n569 = Subtract(x=w1989, y=w1987) -> (x-y=w2006:sgl)
                            n570 = Subtract(x=w1990, y=w1988) -> (x-y=w2004:sgl)
                            n571 = Equal To 0?(x=w2004) -> (x = 0?=w2005:bool)
                            n572 = case shown="False" w2005 {
                              tunnel: w2006 -> [w2013 _]
                              tunnel: w2004 -> [w2012 _]
                              tunnel: [w2011 1000000000000000.0] -> w2003
                              frame False {
                                n573 = Divide(x=w2013, y=w2012) -> (x/y=w2011:sgl)
                              }
                              frame True {
                              }
                            }
                            n574 = Equal To 0?(x=w2003) -> (x = 0?=w2008:bool)
                            n575 = case shown="False" w2008 {
                              tunnel: [w2015 1e-08] -> w2007
                              tunnel: w2003 -> [w2015 _]
                              frame False {
                              }
                              frame True {
                                # "Can't have infinit slope"
                              }
                            }
                            n576 = Divide(x=-1.0, y=w2007) -> (x/y=w2002:dbl)
                            n577 = Inverse Tangent(1:w2002) -> (0:w2000:dbl)
                            n578 = expression code="(x/pi)*180.0" "radians to degrees"(w2000) -> (w2001:dbl)
                            n579 = To Single Precision Float(number=w2001) -> (single precision float=w1998:sgl)
                            n580 = Add(x=w1985, y=sgl 90.0) -> (x+y=w1997:sgl)
                            n581 = Subtract(x=w1998, y=w1997) -> (x-y=w1996:sgl)
                            n582 = Absolute Value(x=w1996) -> (abs(x)=w1995:sgl)
                            n583 = Less Or Equal?(x=w1995, y=sgl 10.0) -> (x <= y?=w1993:bool)
                            n584 = Negate(x=w1991) -> (-x=w1992:sgl)
                            n585 = Select(t=w1992, s=w1993, f=w1991) -> (s? t:f=w1984:sgl)
                          }
                        }
                        n586 = To Word Integer(number=w1978) -> (16bit integer=w1977:i16)
                        n587 = Multiply(x=w1977, y=w1976) -> (x*y=w1975:i32)
                        n588 = To Word Integer(number=w1970) -> (16bit integer=w1974:i16)
                        n589 = Add(x=w1975, y=w1974) -> (x+y=w1973:i32)
                        n590 = To Unsigned Word Integer(number=w1973) -> (unsigned 16bit integer=w1972:u16)
                      }
                    }
                  }
                  frame True {
                    # "Either Current Angle Valid or Image Lock Acheived"
                    # "Go Directly to Track State"
                  }
                }
              }
            }
            n591 = local read "Tracking Timeout\nThreshold"() -> (w1872:i32)
            n592 = Less?(x=w1866, y=w1872) -> (x < y?=w1873:bool)
            n593 = case shown="True" w1873 {
              tunnel: [T5."Recovery Mode" ("Next Main State") T5."Tracking" ("Next Main State")] -> w1877
              frame False {
              }
              frame True {
              }
            }
          }
          frame "Recovery Mode" {
            w2030 = u16 0
            # "Recovery Search Move Count"
            # "***Compltetly resets as of R17, used to just reset to \"Max Recovery Count - 1\""
            # "Increment Recoveyr Mode Count"
            # "Frames Processed"
            # "Choose Next Main State"
            # "Reset recovery count"
            # "Recovery move\nCount"
            # "Recovery Search\nAttempt count"
            # "Move Servo = T"
            # "delta move sum"
            # "Robot Position Valid"
            n594 = local read "Image Lock - Right"() -> (w2034:bool)
            n595 = case shown="\"Recovery Search\"" w2027 {
              tunnel: w2056 -> [_ _]
              tunnel: w2055 -> [_ _]
              tunnel: w2054 -> [_ _]
              tunnel: w2053 -> [_ _]
              tunnel: w2052 -> [_ _]
              tunnel: w2051 -> [_ _]
              tunnel: w2050 -> [w2084 w2164]
              tunnel: [w2076 w2162] -> w2049
              tunnel: [w2073 w2156] -> w2048
              tunnel: [FALSE FALSE] -> w2028
              tunnel: [w2078 w2154] -> w2047
              tunnel: w2044 -> [w2082 _]
              tunnel: w2046 -> [w2085 _]
              tunnel: w2045 -> [w2083 w2159]
              tunnel: [w2075 w2153] -> w2042
              tunnel: [w2074 w2153] -> w2043
              tunnel: w2034 -> [w2072 _]
              tunnel: [w2063 w2163] -> w2041
              tunnel: w2040 -> [w2061 w2151]
              tunnel: w2039 -> [w2066 w2160]
              tunnel: w2038 -> [w2062 w2158]
              tunnel: w2024 -> [_ _]
              tunnel: w2026 -> [_ _]
              tunnel: [FALSE w2155] -> w2036
              tunnel: w2033 -> [w2070 _]
              tunnel: w2032 -> [w2069 _]
              tunnel: [w2066 w2152] -> w2031
              tunnel: w2024 -> [_ w2149]
              frame "Recovery Search" {
                # "Wait for 2 Images to be Processed\nBefore Going to Next Step"
                # "Choose Next Reovery State"
                # "Recovery Search \nAttempt Count"
                # "Move Servo"
                # "Goal Position"
                # "Recovery Search\nmove Count"
                # "Attempt Recovery Search if Other Servo has Valid Angle"
                n596 = local read "Last Track Angle - R"() -> (w2065:sgl)
                n597 = Greater Or Equal?(x=w2061, y=w2062) -> (x >= y?=w2064:bool)
                n598 = case shown="True" w2064 {
                  tunnel: w2085 -> [_ w2105]
                  tunnel: [w2090 w2104] -> w2074
                  tunnel: w2084 -> [w2093 w2103]
                  tunnel: w2083 -> [_ w2102]
                  tunnel: [w2091 w2101] -> w2075
                  tunnel: [w2093 w2100] -> w2076
                  tunnel: [FALSE w2099] -> w2073
                  tunnel: w2070 -> [w2091 w2098]
                  tunnel: w2069 -> [w2090 w2097]
                  tunnel: w2072 -> [_ w2096]
                  tunnel: w2065 -> [_ w2095]
                  tunnel: [w2088 0 ("Frames Processed\nCount - in")] -> w2063
                  tunnel: w2061 -> [w2089 _]
                  frame False {
                    # "Increment Frames Processed"
                    # "WAIT"
                    n599 = Increment(x=w2089) -> (x+1=w2088:i32)
                  }
                  frame True {
                    n600 = case shown="True" w2096 {
                      tunnel: w2095 -> [_ w2118]
                      tunnel: w2098 -> [w2106 w2114]
                      tunnel: w2105 -> [_ w2119]
                      tunnel: [w2109 w2117] -> w2100
                      tunnel: [w2107 w2116] -> w2104
                      tunnel: w2097 -> [w2107 w2115]
                      tunnel: w2103 -> [w2109 w2113]
                      tunnel: w2102 -> [_ w2112]
                      tunnel: [FALSE TRUE] -> w2099
                      tunnel: [w2106 w2110] -> w2101
                      frame False {
                        # "Don't Move bc Other Servo Doesn't Have Image Lock"
                      }
                      frame True {
                        # "Move Servo = T"
                        n601 = Greater Than 0?(x=w2114) -> (x > 0?=w2120:bool)
                        n602 = case shown="False" w2120 {
                          tunnel: w2119 -> [w2121 _]
                          tunnel: w2118 -> [w2122 _]
                          tunnel: [w2125 w2133] -> w2117
                          tunnel: [w2129 w2139] -> w2116
                          tunnel: w2115 -> [w2130 w2139]
                          tunnel: w2114 -> [w2128 w2136]
                          tunnel: [w2127 w2138] -> w2110
                          tunnel: w2113 -> [_ w2134]
                          tunnel: w2112 -> [_ w2131]
                          frame False {
                            # "************************"
                            # "Increment move count to transition\nto Pan mode"
                            # "Increment Recovery Search Attempt Count"
                            # "Move Parallel to Other Servo"
                            n603 = Increment(x=w2130) -> (x+1=w2129:i32)
                            n604 = call "Servo_GP_Angle_Conversion_R0.vi"("Angle In"=w2122, "Mode Select"=1, "Mount Offset"=w2121) -> ("GP out"=w2123:u16)  [unwired: 7 in, 1 out]
                            n605 = Increment(x=w2128) -> (x+1=w2127:i32)
                            n606 = Add(x=w2123, y="Recovery Parallel\nSearch Offset") -> (x+y=w2125:u16)
                          }
                          frame True {
                            # "Apply Direction"
                            # "Step SIze"
                            # "Current Position"
                            # "Attempt to Pan in Steps Towards other Servo"
                            # "Could be same or function of \nregular search step size"
                            # "Max # of Pan\nMoves"
                            # "Pan Towards Other Servo"
                            n607 = Greater Or Equal?(x=w2136, y="Max # Pan Moves") -> (x >= y?=w2137:bool)
                            n608 = case shown="False" w2137 {
                              tunnel: w2136 -> [w2147 _]
                              tunnel: [w2146 u16 0] -> w2138
                              frame False {
                                # "Increment Pan Count"
                                n609 = Increment(x=w2147) -> (x+1=w2146:i32)
                              }
                              frame True {
                                # "Reset move count"
                              }
                            }
                            n610 = local read "Recovery Search\nDirection - L"() -> (w2132:bool)
                            n611 = case shown="True" w2132 {
                              tunnel: w2134 -> [w2141 w2145]
                              tunnel: w2131 -> [w2142 w2144]
                              tunnel: [w2140 w2143] -> w2133
                              frame False {
                                # "CCW"
                                n612 = Add(x=w2141, y=w2142) -> (x+y=w2140:u16)
                              }
                              frame True {
                                # "CW"
                                n613 = Subtract(x=w2145, y=w2144) -> (x-y=w2143:u16)
                              }
                            }
                          }
                        }
                      }
                    }
                  }
                }
                n614 = local read "Max Recovery Count\n(Recovery Search)"() -> (w2067:u16)
                n615 = local read "Max Recovery\nSearch Attempts"() -> (w2068:u16)
                n616 = Less Or Equal?(x=w2074, y=w2068) -> (x <= y?=w2080:bool)
                n617 = Less Or Equal?(x=w2082, y=w2067) -> (x <= y?=w2081:bool)
                n618 = And(x=w2080, y=w2081) -> (x .and. y?=w2079:bool)
                n619 = case shown="True" w2079 {
                  tunnel: [enum16{"Generic Sweep", "Recovery Search"}."Generic Sweep" enum16{"Generic Sweep", "Recovery Search"}."Recovery Search"] -> w2078
                  frame False {
                  }
                  frame True {
                  }
                }
              }
              frame "Generic Sweep" {
                w2153 = u16 0
                # "Image Locked?"
                # "Choose Next Recovery State"
                # "Wait for 2 Images to be Processed\nBefore Going to Next Step"
                # "New Goal Position"
                # "Move Servo"
                # "Frames Processed Count"
                n620 = Greater Or Equal?(x=w2151, y=w2158) -> (x >= y?=w2165:bool)
                n621 = case shown="True" w2165 {
                  tunnel: w2164 -> [w2181 w2197]
                  tunnel: w2159 -> [_ w2195]
                  tunnel: w2160 -> [w2180 w2194]
                  tunnel: [w2181 w2185] -> w2162
                  tunnel: [w2179 0] -> w2163
                  tunnel: [FALSE TRUE] -> w2157
                  tunnel: w2151 -> [w2182 _]
                  tunnel: [w2180 w2188] -> w2152
                  frame False {
                    # "Increment Frames Processed"
                    n622 = Increment(x=w2182) -> (x+1=w2179:i32)
                  }
                  frame True {
                    # "Reset Frames\nProcessed Count"
                    # "SWEEP SEARCH - Startup"
                    # "Multiple New Step\nby Step SIze"
                    # "F = CCW\nT = CW"
                    # "Last Direction"
                    # "Min Step"
                    # "add 10 in case\nactual position\nis lower than GP"
                    # "Set New Step #"
                    # "Choose Direction"
                    # "Nearest step"
                    # "Adjust Actual Posiiton\n to pre-determiend steps"
                    # "Move Servo 1 \"Step\" to\nSearch"
                    n623 = Subtract(x=w2197, y=200) -> (x-y=w2187:i32)
                    n624 = Add(x=5, y=w2187) -> (x+y=w2203:i32)
                    n625 = Quotient & Remainder(x=w2203, y=w2195) -> (floor(x/y)=w2201:i32)  [unwired: 1 out]
                    n626 = To Byte Integer(number=w2201) -> (8bit integer=w2192:i8)
                    n627 = Less?(x=w2192, y=1) -> (x < y?=w2198:bool)
                    n628 = case shown="False" w2198 {
                      tunnel: w2192 -> [w2214 w2222]
                      tunnel: [w2216 FALSE] -> w2188
                      tunnel: [w2215 w2222] -> w2200
                      tunnel: w2194 -> [w2213 _]
                      tunnel: w2195 -> [w2211 _]
                      frame False {
                        # "Max Step"
                        # "# of steps\nminus 1"
                        n629 = Divide(x=300, y=w2211) -> (x/y=w2208:dbl)
                        n630 = To Unsigned Byte Integer(number=w2208) -> (unsigned 8bit integer=w2209:u8)
                        n631 = Greater Or Equal?(x=w2214, y=w2209) -> (x >= y?=w2210:bool)
                        n632 = case shown="True" w2210 {
                          tunnel: [w2217 TRUE] -> w2216
                          tunnel: [w2218 w2219] -> w2215
                          tunnel: w2214 -> [w2218 w2219]
                          tunnel: w2213 -> [w2217 _]
                          frame False {
                            # "No Need to\nChange Direction"
                          }
                          frame True {
                            # "T"
                            # "Move CW"
                          }
                        }
                      }
                      frame True {
                        # "F"
                        # "Move CCW"
                      }
                    }
                    n633 = case shown="True" w2188 {
                      tunnel: w2200 -> [w2205 w2206]
                      tunnel: [w2204 w2207] -> w2196
                      frame False {
                        # "CCW\n+1"
                        n634 = Increment(x=w2205) -> (x+1=w2204:i8)
                      }
                      frame True {
                        # "CW\n-1"
                        n635 = Decrement(x=w2206) -> (x-1=w2207:i8)
                      }
                    }
                    n636 = Multiply(x=w2196, y=w2195) -> (x*y=w2193:u16)
                    n637 = To Unsigned Word Integer(number=w2193) -> (unsigned 16bit integer=w2191:u16)
                    n638 = Add(x=200, y=w2191) -> (x+y=w2185:i32)
                  }
                }
                n639 = local read "Image Lock - Right"() -> (w2150:bool)
                n640 = case shown="True" w2149 {
                  tunnel: [w2168 w2178] -> w2156
                  tunnel: w2157 -> [w2169 _]
                  tunnel: [w2170 enum16{"Generic Sweep", "Recovery Search"}."Generic Sweep"] -> w2154
                  tunnel: [w2167 w2178] -> w2155
                  tunnel: w2150 -> [w2166 _]
                  frame False {
                    # "Is other servo tracking?"
                    n641 = case shown="True" w2166 {
                      tunnel: [enum16{"Generic Sweep", "Recovery Search"}."Generic Sweep" enum16{"Generic Sweep", "Recovery Search"}."Recovery Search"] -> w2170
                      tunnel: w2169 -> [w2173 _]
                      tunnel: [w2173 FALSE] -> w2168
                      tunnel: [FALSE TRUE] -> w2167
                      frame False {
                        # "Stay in Sweep"
                      }
                      frame True {
                        # "G o to Recovery Search  State"
                      }
                    }
                  }
                  frame True {
                    w2178 = FALSE
                    # "Override Move Servo\nCommand bc an Angle Was Found\nduring this Step"
                    # "Stay In Sweep\nLet Main State Machine transition\ninto Tracking"
                  }
                }
              }
            }
            n642 = Increment(x=w2044) -> (x+1=w2025:i32)
            n643 = case shown="False" w2036 {
              tunnel: w2025 -> [w2059 _]
              tunnel: [w2059 0] -> w2037
              frame False {
              }
              frame True {
              }
            }
            n644 = case shown="False" w2024 {
              tunnel: [T5."Recovery Mode" ("Next Main State") T5."Tracking" ("Next Main State")] -> w2035
              frame False {
              }
              frame True {
              }
            }
          }
        }
        "Current Move Delta - L" <- w1799
        n645 = Less?(x=w1826, y=w1825) -> (x < y?=w1824:bool)
        n646 = local write "New Data  Flag\nLeft Servo"(FALSE) -> ()
        n647 = Select(t=w1825, s=w1824, f=w1826) -> (s? t:f=w1821:i32)
        n648 = Greater?(x=w1821, y=w1822) -> (0:w1823:bool)
        n649 = Select(t=w1822, s=w1823, f=w1821) -> (s? t:f=w1820:i32)
      }
    }
    "Next Main State - Left" <- w1248
    "Next Tracking State - Left" <- w1231
    "Next Recovery State - Left" <- w1229
    n650 = case shown="True" w1212 {
      tunnel: [w1297 w1335] -> w1182
      tunnel: [w1291 w1334] -> w1181
      tunnel: w1217 -> [w1292 w1333]
      tunnel: w1214 -> [_ w1332]
      tunnel: "Track Angle Valid  - Right" -> [_ w1331]
      tunnel: w1211 -> [_ w1330]
      tunnel: w1210 -> [w1297 w1329]
      tunnel: "Mounting Offset - Right" -> [_ w1328]
      tunnel: w1205 -> [w1288 w1327]
      tunnel: w1203 -> [_ w1326]
      tunnel: w1200 -> [w1289 w1325]
      tunnel: w1198 -> [_ w1324]
      tunnel: w1197 -> [_ w1323]
      tunnel: w1196 -> [_ w1322]
      tunnel: w1195 -> [_ w1321]
      tunnel: w1193 -> [w1287 w1320]
      tunnel: w1202 -> [w1286 w1319]
      tunnel: w1201 -> [w1290 w1318]
      tunnel: w1207 -> [_ w1317]
      tunnel: w1206 -> [_ w1316]
      tunnel: w1204 -> [_ w1315]
      tunnel: [0 w1314] -> w1183
      tunnel: [w1292 w1313] -> w1180
      tunnel: [w1291 w1312] -> w1187
      tunnel: [w1290 w1311] -> w1188
      tunnel: [w1286 w1310] -> w1189
      tunnel: [w1289 w1309] -> w1190
      tunnel: [w1287 w1308] -> w1191
      tunnel: w1194 -> [_ w1307]
      tunnel: [w1288 w1306] -> w1192
      tunnel: w1199 -> [_ w1305]
      tunnel: w1209 -> [w1295 w1304]
      tunnel: w1215 -> [w1294 w1303]
      tunnel: [w1295 w1302] -> w1184
      tunnel: [w1294 w1301] -> w1186
      tunnel: w1216 -> [w1293 w1300]
      tunnel: [w1293 w1299] -> w1185
      frame False {
        w1291 = FALSE
        # "Recovery Mode COunt"
        # "Frames Processed - L"
        # "Recovery Search move Count - L"
        # "Recovery Search Attempt Count- L"
        # "WAITING FOR NEW IMAGE, RETAIN ALL VALUES"
      }
      frame True {
        w1337 = u16 1023
        w1340 = u16 0
        # "New Tracking State"
        # "Tracking Timeout Count"
        # "Next Main State"
        # "Next Recovery State"
        # "Reset Respond"
        # "Search Direction"
        # "Recovery Count"
        # "Recovery Search move Count"
        # "Recovery Search Attempt Count"
        # "Frames Processed"
        # "Apply Floor/Ceiling to Goal Position"
        # "Current move Delta"
        # "Service Track Angle Flag"
        # "Move Servo"
        # "Goal Position"
        # "Go to Current State"
        n651 = case shown="\"Recovery Mode\"" w1333 {
          tunnel: w1329 -> [w1358 w1430 w1598]
          tunnel: w1330 -> [_ w1432 _]
          tunnel: w1315 -> [w1357 _ w1593]
          tunnel: w1327 -> [w1356 w1413 w1587]
          tunnel: [w1355 w1428 w1597] -> w1341
          tunnel: [w1353 w1429 w1596] -> w1334
          tunnel: w1331 -> [_ w1423 w1574]
          tunnel: [w1351 w1425 w1583] -> w1313
          tunnel: w1332 -> [w1342 w1424 w1572]
          tunnel: w1328 -> [_ w1433 w1594]
          tunnel: w1317 -> [_ w1431 _]
          tunnel: [w1345 w1427 w1578] -> w1314
          tunnel: w1316 -> [_ w1426 _]
          tunnel: w1325 -> [w1350 _ w1588]
          tunnel: [enum16{"Generic Sweep", "Recovery Search"}."Recovery Search" enum16{"Generic Sweep", "Recovery Search"}."Recovery Search" w1595] -> w1299
          tunnel: w1320 -> [_ _ w1592]
          tunnel: w1300 -> [_ _ w1575]
          tunnel: w1326 -> [_ w1410 w1604]
          tunnel: w1307 -> [_ w1406 w1599]
          tunnel: w1322 -> [_ w1416 w1601]
          tunnel: w1323 -> [_ w1417 w1602]
          tunnel: w1324 -> [_ w1418 w1603]
          tunnel: w1321 -> [_ w1415 w1600]
          tunnel: [FALSE w1412 w1576] -> w1312
          tunnel: w1305 -> [w1349 _ w1586]
          tunnel: [w1345 w1407 w1585] -> w1308
          tunnel: [w1345 w1407 w1591] -> w1311
          tunnel: [w1345 w1407 w1590] -> w1310
          tunnel: [w1348 w1408 w1589] -> w1309
          tunnel: w1319 -> [_ _ w1581]
          tunnel: w1318 -> [_ _ w1580]
          tunnel: [w1346 w1413 w1579] -> w1306
          tunnel: w1304 -> [_ w1422 _]
          tunnel: [w1345 w1414 w1578] -> w1302
          tunnel: w1303 -> [_ w1419 _]
          tunnel: [enum16{"Track", "Reactive Predict", ""}."Track" ("Initial Tracking State - Right") w1411 enum16{"Track", "Reactive Predict", ""}."Track" ("Initial Tracking State - Right")] -> w1301
          frame "Start Up Search", Default {
            w1345 = u16 0
            # "Image Lock"
            # "Search Direction"
            # "Wait for 'x' Images to be Processed\nBefore Going to Next Step"
            # "Next Main State"
            # "New Goal Position"
            # "Move Servo"
            # "Choose Next State"
            # "Frames Processed Count"
            n652 = Greater Or Equal?(x=w1350, y=w1349) -> (x >= y?=w1354:bool)
            n653 = case shown="True" w1354 {
              tunnel: w1358 -> [w1368 w1380]
              tunnel: w1357 -> [_ w1378]
              tunnel: w1356 -> [w1367 w1377]
              tunnel: [w1368 w1374] -> w1355
              tunnel: [w1366 0] -> w1348
              tunnel: [FALSE TRUE] -> w1352
              tunnel: w1350 -> [w1369 _]
              tunnel: [w1367 w1371] -> w1346
              frame False {
                # "Wait until Min Number of Frames (per search/step) Processed"
                # "Increase Frames\nProcessed Count"
                n654 = Increment(x=w1369) -> (x+1=w1366:i32)
              }
              frame True {
                # "Reset Frames\nProcessed Count"
                # "SWEEP SEARCH - Startup"
                # "Multiple New Step\nby Step SIze"
                # "F = CCW\nT = CW"
                # "Last Direction"
                # "Min Step"
                # "add in case\nactual position\nis lower than GP"
                # "Set New Step #"
                # "Choose Direction"
                # "Nearest step"
                # "Adjust Actual Posiiton\n to pre-determiend steps"
                # "Move Servo 1 \"Step\" to\nSearch"
                n655 = Add(x=3, y=w1380) -> (x+y=w1386:i32)
                n656 = Quotient & Remainder(x=w1386, y=w1378) -> (floor(x/y)=w1384:i32)  [unwired: 1 out]
                n657 = To Byte Integer(number=w1384) -> (8bit integer=w1375:i8)
                n658 = Less?(x=w1375, y=1) -> (x < y?=w1381:bool)
                n659 = case shown="False" w1381 {
                  tunnel: w1375 -> [w1397 w1405]
                  tunnel: [w1399 FALSE] -> w1371
                  tunnel: [w1398 w1405] -> w1383
                  tunnel: w1377 -> [w1396 _]
                  tunnel: w1378 -> [w1394 _]
                  frame False {
                    # "Max Step"
                    # "# of steps\nminus 1"
                    n660 = Divide(x=1024, y=w1394) -> (x/y=w1391:dbl)
                    n661 = To Unsigned Byte Integer(number=w1391) -> (unsigned 8bit integer=w1392:u8)
                    n662 = Greater Or Equal?(x=w1397, y=w1392) -> (x >= y?=w1393:bool)
                    n663 = case shown="True" w1393 {
                      tunnel: [w1400 TRUE] -> w1399
                      tunnel: [w1401 w1402] -> w1398
                      tunnel: w1397 -> [w1401 w1402]
                      tunnel: w1396 -> [w1400 _]
                      frame False {
                        # "No Need to\nChange Direction"
                      }
                      frame True {
                        # "T"
                        # "Move CW"
                      }
                    }
                  }
                  frame True {
                    # "F"
                    # "Move CCW"
                  }
                }
                n664 = case shown="False" w1371 {
                  tunnel: w1383 -> [w1388 w1389]
                  tunnel: [w1387 w1390] -> w1379
                  frame False {
                    # "CCW\n+1"
                    n665 = Increment(x=w1388) -> (x+1=w1387:i8)
                  }
                  frame True {
                    # "CW\n-1"
                    n666 = Decrement(x=w1389) -> (x-1=w1390:i8)
                  }
                }
                n667 = Multiply(x=w1379, y=w1378) -> (x*y=w1376:u16)
                n668 = To Unsigned Word Integer(number=w1376) -> (unsigned 16bit integer=w1374:u16)
              }
            }
            n669 = case shown="False" w1342 {
              tunnel: [w1360 FALSE] -> w1353
              tunnel: w1352 -> [w1360 _]
              tunnel: [w1361 T5."Tracking" ("Next Main State")] -> w1351
              frame False {
                # "Check other Servo\nStay in Startup  State"
                n670 = local read "Image Lock - Left"() -> (w1359:bool)
                n671 = case shown="False" w1359 {
                  tunnel: [T5."Start Up Search" ("Next Main State") T5."Recovery Mode" ("Next Main State")] -> w1361
                  frame False {
                  }
                  frame True {
                  }
                }
              }
              frame True {
                # "Override Move Servo\nCommand bc an Angle Was Found\nduring this Step"
                # "Transition to Tracking State When\nImage Processing has Locked"
              }
            }
          }
          frame "Tracking" {
            w1407 = 0
            # "Frames Processed Count"
            # "Image Lock - L"
            # "Track Angle Valid"
            # "Tracking Angle"
            # "Tracking Timeout Count"
            # "Max ove delta"
            # "Move delta threshold"
            # "mount offset"
            # "Current Position"
            # "Move Respond"
            # "Trackin Timeout count"
            # "Move Servo"
            # "delta"
            # "GP"
            # "Reset Move Respond"
            # "New Tracking State"
            # "Delta Move Sum"
            # "Choose Next State"
            n672 = case shown="\"Track\", Default" w1419 {
              tunnel: w1433 -> [w1451 _]
              tunnel: w1432 -> [w1450 _]
              tunnel: w1431 -> [w1449 _]
              tunnel: w1430 -> [w1448 w1496]
              tunnel: [w1447 w1494] -> w1429
              tunnel: [w1446 w1502] -> w1428
              tunnel: [w1445 0] -> w1427
              tunnel: w1426 -> [w1444 _]
              tunnel: w1424 -> [w1443 w1486]
              tunnel: w1423 -> [w1442 w1489]
              tunnel: w1422 -> [w1441 w1491]
              tunnel: w1418 -> [_ w1501]
              tunnel: w1417 -> [_ w1500]
              tunnel: w1416 -> [_ w1499]
              tunnel: w1415 -> [_ w1498]
              tunnel: w1410 -> [_ w1497]
              tunnel: w1406 -> [_ w1495]
              tunnel: [TRUE w1492] -> w1412
              tunnel: [w1438 w1490] -> w1414
              tunnel: [w1436 w1488] -> w1411
              tunnel: [0 0] -> w1408
              frame "Track", Default {
                # "Reset"
                # "Tracking Timeout"
                # "Move Delta"
                # "Goal Position"
                # "Tracking Move"
                # "Move Servo"
                # "Only Consider Tracking Angle\n\nIF\n\nImage Locked        == T\nTrack Angle Flag   == T"
                n673 = And(x=w1443, y=w1442) -> (x .and. y?=w1435:bool)
                n674 = case shown="True" w1435 {
                  tunnel: w1451 -> [_ w1459]
                  tunnel: w1450 -> [_ w1457]
                  tunnel: w1449 -> [_ w1474]
                  tunnel: w1448 -> [w1454 w1464]
                  tunnel: [w1454 w1473] -> w1446
                  tunnel: [w1456 w1472] -> w1447
                  tunnel: [w1456 w1471] -> _
                  tunnel: [u16 0 w1470] -> w1445
                  tunnel: w1444 -> [_ w1466]
                  tunnel: w1441 -> [w1453 _]
                  tunnel: [w1452 0] -> w1438
                  frame False {
                    w1456 = FALSE
                    # "Increment timeout"
                    n675 = Increment(x=w1453) -> (x+1=w1452:i32)
                  }
                  frame True {
                    # "******"
                    # "Move to Tracking Angle \n\nif delta is greater than move servo threshold\nAND less than max move threshold"
                    n676 = call "Servo_GP_Angle_Conversion_R0.vi"("Angle In"=w1457, "Mode Select"=1, "Mount Offset"=w1459) -> ("GP out"=w1458:u16)  [unwired: 7 in, 1 out]
                    n677 = To Word Integer(number=w1464) -> (16bit integer=w1462:i16)
                    n678 = To Word Integer(number=w1458) -> (16bit integer=w1475:i16)
                    n679 = Subtract(x=w1475, y=w1462) -> (x-y=w1465:i16)
                    n680 = Absolute Value(x=w1465) -> (abs(x)=w1461:i16)
                    n681 = Greater Or Equal?(x=w1461, y=w1474) -> (x >= y?=w1468:bool)
                    n682 = Less Or Equal?(x=w1461, y=w1466) -> (x <= y?=w1467:bool)
                    n683 = And(x=w1468, y=w1467) -> (x .and. y?=w1469:bool)
                    n684 = case shown="True" w1469 {
                      tunnel: w1458 -> [_ w1480]
                      tunnel: [w1477 w1480] -> w1473
                      tunnel: [w1478 w1482] -> w1472
                      tunnel: [w1478 w1482] -> w1471
                      tunnel: w1464 -> [w1477 _]
                      tunnel: w1461 -> [_ w1481]
                      tunnel: [u16 0 w1481] -> w1470
                      tunnel: w1457 -> [_ w1479]
                      frame False {
                        w1478 = FALSE
                        # "Don't Move"
                      }
                      frame True {
                        w1482 = TRUE
                        # "Current Delta"
                        # "Use new Track Angle"
                        n685 = local write "Last Track Angle - R"(w1479) -> ()
                      }
                    }
                  }
                }
                n686 = local read "Timeout to \nEnable Reactive Predict"() -> (w1439:u16)
                n687 = Less?(x=w1438, y=w1439) -> (x < y?=w1437:bool)
                n688 = case shown="True" w1437 {
                  tunnel: [enum16{"Track", "Reactive Predict", ""}."Reactive Predict" ("Initial Tracking State - Right") enum16{"Track", "Reactive Predict", ""}."Track" ("Initial Tracking State - Right")] -> w1436
                  frame False {
                  }
                  frame True {
                  }
                }
              }
              frame "Reactive Predict" {
                # "Choose New\nTracking State"
                n689 = Or(x=w1486, y=w1489) -> (x .or. y?=w1485:bool)
                n690 = case shown="False" w1485 {
                  tunnel: [w1515 w1568] -> w1502
                  tunnel: w1501 -> [w1514 _]
                  tunnel: w1500 -> [w1513 _]
                  tunnel: w1499 -> [w1512 _]
                  tunnel: w1498 -> [w1511 _]
                  tunnel: w1497 -> [w1510 _]
                  tunnel: w1495 -> [w1509 _]
                  tunnel: [w1508 FALSE] -> w1494
                  tunnel: [w1507 TRUE] -> w1492
                  tunnel: w1491 -> [w1506 _]
                  tunnel: [w1505 0] -> w1490
                  tunnel: [enum16{"Track", "Reactive Predict", ""}."Reactive Predict" ("Initial Tracking State - Right") enum16{"Track", "Reactive Predict", ""}."Track" ("Initial Tracking State - Right")] -> w1488
                  tunnel: w1496 -> [w1503 w1568]
                  frame False {
                    # "Stay in Reactive State"
                    # "Increment Track Timeout"
                    # "Move Respond Flag"
                    n691 = Increment(x=w1506) -> (x+1=w1505:i32)
                    n692 = case shown="True" w1510 {
                      tunnel: w1514 -> [_ w1530]
                      tunnel: w1513 -> [_ w1529]
                      tunnel: w1512 -> [_ w1528]
                      tunnel: w1511 -> [_ w1527]
                      tunnel: w1509 -> [_ w1524]
                      tunnel: [w1516 w1520] -> w1515
                      tunnel: [w1517 w1519] -> w1508
                      tunnel: [w1517 w1519] -> w1507
                      tunnel: w1503 -> [w1516 w1518]
                      frame False {
                        w1517 = FALSE
                        # "Reset Move Respond = F"
                        # "Move Servo = F"
                      }
                      frame True {
                        w1519 = TRUE
                        # "Position Lock"
                        # "Current Servo\nPosition"
                        # "Reset Move\nRespond = T"
                        # "Move Servo = T"
                        # "Apply Direction \nto Offset (delta sum)"
                        # "Check Last Known Position of Robot"
                        n693 = case shown="True" w1530 {
                          tunnel: w1529 -> [_ w1558]
                          tunnel: w1528 -> [_ w1533]
                          tunnel: w1527 -> [_ w1534]
                          tunnel: [sgl 1.0 ("y") w1532] -> w1526
                          frame False {
                            # "No Position Data Available"
                            # "Default is to move\nSame Direction as other\nServo"
                          }
                          frame True {
                            w1539 = sgl 1.0 ("y")
                            # "Use previous position/orientation to Guess Which Direction to Move Servo"
                            # "Choose Search Direction"
                            # "\"Perpendicular \nThreshold\""
                            # "If Orientation is\n ~Perpendicular -> Start Search\n in Opposite Direction of Other"
                            # "****add 90 until orientation angle is fixed"
                            # "Last Orientation"
                            # "Convert to Rad"
                            # "Avoid Divide by 0"
                            # "-1/m"
                            # "Calculate Normal Line to \nLast Robot Position\nfrom Center Beacon"
                            # "last Position \nCoordinates"
                            n694 = Unbundle(w1558) -> ("X"=w1538:sgl, "Y"=w1537:sgl)
                            n695 = Unbundle(w1534) -> ("X"=w1536:sgl, "Y"=w1535:sgl)
                            n696 = Subtract(x=w1537, y=w1535) -> (x-y=w1554:sgl)
                            n697 = Subtract(x=w1538, y=w1536) -> (x-y=w1552:sgl)
                            n698 = Equal To 0?(x=w1552) -> (x = 0?=w1553:bool)
                            n699 = case shown="False" w1553 {
                              tunnel: w1554 -> [w1561 _]
                              tunnel: w1552 -> [w1560 _]
                              tunnel: [w1559 1000000000000000.0] -> w1551
                              frame False {
                                n700 = Divide(x=w1561, y=w1560) -> (x/y=w1559:sgl)
                              }
                              frame True {
                              }
                            }
                            n701 = Equal To 0?(x=w1551) -> (x = 0?=w1556:bool)
                            n702 = case shown="False" w1556 {
                              tunnel: [w1563 1e-08] -> w1555
                              tunnel: w1551 -> [w1563 _]
                              frame False {
                              }
                              frame True {
                                # "Can't have infinit slope"
                              }
                            }
                            n703 = Divide(x=-1.0, y=w1555) -> (x/y=w1550:dbl)
                            n704 = Inverse Tangent(1:w1550) -> (0:w1548:dbl)
                            n705 = expression code="(x/pi)*180.0" "radians to degrees"(w1548) -> (w1549:dbl)
                            n706 = To Single Precision Float(number=w1549) -> (single precision float=w1546:sgl)
                            n707 = Add(x=w1533, y=sgl 90.0) -> (x+y=w1545:sgl)
                            n708 = Subtract(x=w1546, y=w1545) -> (x-y=w1544:sgl)
                            n709 = Absolute Value(x=w1544) -> (abs(x)=w1543:sgl)
                            n710 = Less Or Equal?(x=w1543, y=sgl 10.0) -> (x <= y?=w1541:bool)
                            n711 = Negate(x=w1539) -> (-x=w1540:sgl)
                            n712 = Select(t=w1540, s=w1541, f=w1539) -> (s? t:f=w1532:sgl)
                          }
                        }
                        n713 = To Word Integer(number=w1526) -> (16bit integer=w1525:i16)
                        n714 = Multiply(x=w1525, y=w1524) -> (x*y=w1523:i32)
                        n715 = To Word Integer(number=w1518) -> (16bit integer=w1522:i16)
                        n716 = Add(x=w1523, y=w1522) -> (x+y=w1521:i32)
                        n717 = To Unsigned Word Integer(number=w1521) -> (unsigned 16bit integer=w1520:u16)
                      }
                    }
                  }
                  frame True {
                    # "Either Current Angle Valid or Image Lock Acheived"
                    # "Go Directly to Track State"
                  }
                }
              }
            }
            n718 = local read "Tracking Timeout\nThreshold"() -> (w1420:i32)
            n719 = Less?(x=w1414, y=w1420) -> (x < y?=w1421:bool)
            n720 = case shown="True" w1421 {
              tunnel: [T5."Recovery Mode" ("Next Main State") T5."Tracking" ("Next Main State")] -> w1425
              frame False {
              }
              frame True {
              }
            }
          }
          frame "Recovery Mode" {
            w1578 = u16 0
            # "Recovery Search Move Count"
            # "***Compltetly resets as of R17, used to just reset to \"Max Recovery Count - 1\""
            # "Increment Recoveyr Mode Count"
            # "Frames Processed"
            # "Choose Next Main State"
            # "Reset recovery count"
            # "Recovery move\nCount"
            # "Recovery Search\nAttempt count"
            # "Move Servo = T"
            # "delta move sum"
            # "Robot Position Valid"
            n721 = local read "Image Lock - Left"() -> (w1582:bool)
            n722 = case shown="\"Generic Sweep\"" w1575 {
              tunnel: w1604 -> [_ _]
              tunnel: w1603 -> [_ _]
              tunnel: w1602 -> [_ _]
              tunnel: w1601 -> [_ _]
              tunnel: w1600 -> [_ _]
              tunnel: w1599 -> [_ _]
              tunnel: w1598 -> [w1632 w1712]
              tunnel: [w1624 w1710] -> w1597
              tunnel: [w1621 w1704] -> w1596
              tunnel: [FALSE FALSE] -> w1576
              tunnel: [w1626 w1702] -> w1595
              tunnel: w1592 -> [w1630 _]
              tunnel: w1594 -> [w1633 _]
              tunnel: w1593 -> [w1631 w1707]
              tunnel: [w1623 w1701] -> w1590
              tunnel: [w1622 w1701] -> w1591
              tunnel: w1582 -> [w1620 _]
              tunnel: [w1611 w1711] -> w1589
              tunnel: w1588 -> [w1609 w1699]
              tunnel: w1587 -> [w1614 w1708]
              tunnel: w1586 -> [w1610 w1706]
              tunnel: w1572 -> [_ _]
              tunnel: w1574 -> [_ _]
              tunnel: [FALSE w1703] -> w1584
              tunnel: w1581 -> [w1618 _]
              tunnel: w1580 -> [w1617 _]
              tunnel: [w1614 w1700] -> w1579
              tunnel: w1572 -> [_ w1697]
              frame "Recovery Search" {
                # "Wait for 2 Images to be Processed\nBefore Going to Next Step"
                # "Choose Next Reovery State"
                # "Recovery Search \nAttempt Count"
                # "Move Servo"
                # "Goal Position"
                # "Recovery Search\nmove Count"
                # "Attempt Recovery Search if Other Servo has Valid Angle"
                n723 = local read "Last Track Angle - L"() -> (w1613:sgl)
                n724 = Greater Or Equal?(x=w1609, y=w1610) -> (x >= y?=w1612:bool)
                n725 = case shown="True" w1612 {
                  tunnel: w1633 -> [_ w1653]
                  tunnel: [w1638 w1652] -> w1622
                  tunnel: w1632 -> [w1641 w1651]
                  tunnel: w1631 -> [_ w1650]
                  tunnel: [w1639 w1649] -> w1623
                  tunnel: [w1641 w1648] -> w1624
                  tunnel: [FALSE w1647] -> w1621
                  tunnel: w1618 -> [w1639 w1646]
                  tunnel: w1617 -> [w1638 w1645]
                  tunnel: w1620 -> [_ w1644]
                  tunnel: w1613 -> [_ w1643]
                  tunnel: [w1636 0 ("Frames Processed\nCount - in")] -> w1611
                  tunnel: w1609 -> [w1637 _]
                  frame False {
                    # "Increment Frames Processed"
                    # "WAIT"
                    n726 = Increment(x=w1637) -> (x+1=w1636:i32)
                  }
                  frame True {
                    n727 = case shown="True" w1644 {
                      tunnel: w1643 -> [_ w1666]
                      tunnel: w1646 -> [w1654 w1662]
                      tunnel: w1653 -> [_ w1667]
                      tunnel: [w1657 w1665] -> w1648
                      tunnel: [w1655 w1664] -> w1652
                      tunnel: w1645 -> [w1655 w1663]
                      tunnel: w1651 -> [w1657 w1661]
                      tunnel: w1650 -> [_ w1660]
                      tunnel: [FALSE TRUE] -> w1647
                      tunnel: [w1654 w1658] -> w1649
                      frame False {
                        # "Don't Move bc Other Servo Doesn't Have Image Lock"
                      }
                      frame True {
                        # "Move Servo = T"
                        n728 = Greater Than 0?(x=w1662) -> (x > 0?=w1668:bool)
                        n729 = case shown="False" w1668 {
                          tunnel: w1667 -> [w1670 _]
                          tunnel: w1666 -> [w1671 _]
                          tunnel: [w1674 w1682] -> w1665
                          tunnel: [w1677 w1687] -> w1664
                          tunnel: w1663 -> [w1678 w1687]
                          tunnel: w1662 -> [w1676 w1684]
                          tunnel: [w1675 w1686] -> w1658
                          tunnel: w1661 -> [_ w1683]
                          tunnel: w1660 -> [_ w1680]
                          frame False {
                            # "************************"
                            # "Increment move count to transition\nto Pan mode"
                            # "Increment Recovery Search Attempt Count"
                            # "Move Parallel to Other Servo"
                            n730 = Increment(x=w1678) -> (x+1=w1677:i32)
                            n731 = call "Servo_GP_Angle_Conversion_R0.vi"("Angle In"=w1671, "Mode Select"=1, "Mount Offset"=w1670) -> ("GP out"=w1669:u16)  [unwired: 7 in, 1 out]
                            n732 = Increment(x=w1676) -> (x+1=w1675:i32)
                            n733 = local read "Recovery Parallel\nSearch Offset"() -> (w1673:u16)
                            n734 = Add(x=w1669, y=w1673) -> (x+y=w1674:u16)
                          }
                          frame True {
                            # "Apply Direction"
                            # "Step SIze"
                            # "Current Position"
                            # "Attempt to Pan in Steps Towards other Servo"
                            # "Could be same or function of \nregular search step size"
                            # "Max # of Pan\nMoves"
                            # "Pan Towards Other Servo"
                            n735 = local read "Max # Pan Moves"() -> (w1679:u16)
                            n736 = Greater Or Equal?(x=w1684, y=w1679) -> (x >= y?=w1685:bool)
                            n737 = case shown="False" w1685 {
                              tunnel: w1684 -> [w1695 _]
                              tunnel: [w1694 u16 0] -> w1686
                              frame False {
                                # "Increment Pan Count"
                                n738 = Increment(x=w1695) -> (x+1=w1694:i32)
                              }
                              frame True {
                                # "Reset move count"
                              }
                            }
                            n739 = local read "Recovery Search\nDirection - R"() -> (w1681:bool)
                            n740 = case shown="True" w1681 {
                              tunnel: w1683 -> [w1689 w1693]
                              tunnel: w1680 -> [w1690 w1692]
                              tunnel: [w1688 w1691] -> w1682
                              frame False {
                                # "CCW"
                                n741 = Add(x=w1689, y=w1690) -> (x+y=w1688:u16)
                              }
                              frame True {
                                # "CW"
                                n742 = Subtract(x=w1693, y=w1692) -> (x-y=w1691:u16)
                              }
                            }
                          }
                        }
                      }
                    }
                  }
                }
                n743 = local read "Max Recovery Count\n(Recovery Search)"() -> (w1615:u16)
                n744 = local read "Max Recovery\nSearch Attempts"() -> (w1616:u16)
                n745 = Less Or Equal?(x=w1622, y=w1616) -> (x <= y?=w1628:bool)
                n746 = Less Or Equal?(x=w1630, y=w1615) -> (x <= y?=w1629:bool)
                n747 = And(x=w1628, y=w1629) -> (x .and. y?=w1627:bool)
                n748 = case shown="True" w1627 {
                  tunnel: [enum16{"Generic Sweep", "Recovery Search"}."Generic Sweep" enum16{"Generic Sweep", "Recovery Search"}."Recovery Search"] -> w1626
                  frame False {
                  }
                  frame True {
                  }
                }
              }
              frame "Generic Sweep" {
                w1701 = u16 0
                # "Image Locked?"
                # "Choose Next Recovery State"
                # "Wait for 2 Images to be Processed\nBefore Going to Next Step"
                # "New Goal Position"
                # "Move Servo"
                # "Frames Processed Count"
                n749 = Greater Or Equal?(x=w1699, y=w1706) -> (x >= y?=w1713:bool)
                n750 = case shown="True" w1713 {
                  tunnel: w1712 -> [w1729 w1745]
                  tunnel: w1707 -> [_ w1743]
                  tunnel: w1708 -> [w1728 w1742]
                  tunnel: [w1729 w1735] -> w1710
                  tunnel: [w1727 0] -> w1711
                  tunnel: [FALSE TRUE] -> w1705
                  tunnel: w1699 -> [w1730 _]
                  tunnel: [w1728 w1736] -> w1700
                  frame False {
                    # "Increment Frames Processed"
                    n751 = Increment(x=w1730) -> (x+1=w1727:i32)
                  }
                  frame True {
                    # "Reset Frames\nProcessed Count"
                    # "SWEEP SEARCH - Startup"
                    # "Multiple New Step\nby Step SIze"
                    # "F = CCW\nT = CW"
                    # "Last Direction"
                    # "Min Step"
                    # "add 10 in case\nactual position\nis lower than GP"
                    # "Set New Step #"
                    # "Choose Direction"
                    # "Nearest step"
                    # "Adjust Actual Posiiton\n to pre-determiend steps"
                    # "Move Servo 1 \"Step\" to\nSearch"
                    n752 = Subtract(x=w1745, y=u16 524) -> (x-y=w1733:u16)
                    n753 = Add(x=5, y=w1733) -> (x+y=w1751:i32)
                    n754 = Quotient & Remainder(x=w1751, y=w1743) -> (floor(x/y)=w1749:i32)  [unwired: 1 out]
                    n755 = To Byte Integer(number=w1749) -> (8bit integer=w1740:i8)
                    n756 = Less?(x=w1740, y=1) -> (x < y?=w1746:bool)
                    n757 = case shown="False" w1746 {
                      tunnel: w1740 -> [w1762 w1770]
                      tunnel: [w1764 FALSE] -> w1736
                      tunnel: [w1763 w1770] -> w1748
                      tunnel: w1742 -> [w1761 _]
                      tunnel: w1743 -> [w1759 _]
                      frame False {
                        # "Max Step"
                        # "# of steps\nminus 1"
                        n758 = Divide(x=300, y=w1759) -> (x/y=w1756:dbl)
                        n759 = To Unsigned Byte Integer(number=w1756) -> (unsigned 8bit integer=w1757:u8)
                        n760 = Greater Or Equal?(x=w1762, y=w1757) -> (x >= y?=w1758:bool)
                        n761 = case shown="True" w1758 {
                          tunnel: [w1765 TRUE] -> w1764
                          tunnel: [w1766 w1767] -> w1763
                          tunnel: w1762 -> [w1766 w1767]
                          tunnel: w1761 -> [w1765 _]
                          frame False {
                            # "No Need to\nChange Direction"
                          }
                          frame True {
                            # "T"
                            # "Move CW"
                          }
                        }
                      }
                      frame True {
                        # "F"
                        # "Move CCW"
                      }
                    }
                    n762 = case shown="True" w1736 {
                      tunnel: w1748 -> [w1753 w1754]
                      tunnel: [w1752 w1755] -> w1744
                      frame False {
                        # "CCW\n+1"
                        n763 = Increment(x=w1753) -> (x+1=w1752:i8)
                      }
                      frame True {
                        # "CW\n-1"
                        n764 = Decrement(x=w1754) -> (x-1=w1755:i8)
                      }
                    }
                    n765 = Multiply(x=w1744, y=w1743) -> (x*y=w1741:u16)
                    n766 = To Unsigned Word Integer(number=w1741) -> (unsigned 16bit integer=w1739:u16)
                    n767 = Add(x=w1739, y=u16 524) -> (x+y=w1735:u16)
                  }
                }
                n768 = local read "Image Lock - Left"() -> (w1698:bool)
                n769 = case shown="False" w1697 {
                  tunnel: [w1716 w1726] -> w1704
                  tunnel: w1705 -> [w1717 _]
                  tunnel: [w1718 enum16{"Generic Sweep", "Recovery Search"}."Generic Sweep"] -> w1702
                  tunnel: [w1715 w1726] -> w1703
                  tunnel: w1698 -> [w1714 _]
                  frame False {
                    # "Is other servo tracking?"
                    n770 = case shown="True" w1714 {
                      tunnel: [enum16{"Generic Sweep", "Recovery Search"}."Generic Sweep" enum16{"Generic Sweep", "Recovery Search"}."Recovery Search"] -> w1718
                      tunnel: w1717 -> [w1721 _]
                      tunnel: [w1721 FALSE] -> w1716
                      tunnel: [FALSE TRUE] -> w1715
                      frame False {
                        # "Stay in Sweep"
                      }
                      frame True {
                        # "G o to Recovery Search  State"
                      }
                    }
                  }
                  frame True {
                    w1726 = FALSE
                    # "Override Move Servo\nCommand bc an Angle Was Found\nduring this Step"
                    # "Stay In Sweep\nLet Main State Machine transition\ninto Tracking"
                  }
                }
              }
            }
            n771 = Increment(x=w1592) -> (x+1=w1573:i32)
            n772 = case shown="False" w1584 {
              tunnel: w1573 -> [w1607 _]
              tunnel: [w1607 0] -> w1585
              frame False {
              }
              frame True {
              }
            }
            n773 = case shown="False" w1572 {
              tunnel: [T5."Recovery Mode" ("Next Main State") T5."Tracking" ("Next Main State")] -> w1583
              frame False {
              }
              frame True {
              }
            }
          }
        }
        "Current Move Delta - R" <- w1314
        n774 = local write "New Data  Flag\nRight Servo"(FALSE) -> ()
        n775 = Less?(x=w1341, y=w1340) -> (x < y?=w1339:bool)
        n776 = Select(t=w1340, s=w1339, f=w1341) -> (s? t:f=w1336:u16)
        n777 = Greater?(x=w1336, y=w1337) -> (0:w1338:bool)
        n778 = Select(t=w1337, s=w1338, f=w1336) -> (s? t:f=w1335:u16)
      }
    }
    "Next Main State - Right" <- w1180
    "Next Tracking State - Right" <- w1186
    "Next Recovery State - Right" <- w1185
    n779 = flat-sequence {
      tunnel: w1271 -> [w2229]
      tunnel: w1181 -> [w2228]
      tunnel: w1272 -> [w2231]
      tunnel: w1182 -> [w2230]
      tunnel: [w2229] -> w1285
      tunnel: [w2228] -> w1284
      tunnel: w1285 -> [w2237]
      tunnel: [w2236] -> w1280
      tunnel: [w2235] -> w1281
      tunnel: w1284 -> [w2234]
      frame #0 {
        # "Only Update GP if Moving Servo"
        n780 = case shown="True" w2229 {
          tunnel: w2231 -> [_ w2233]
          frame False {
          }
          frame True {
            # "Update Goal Position"
            n781 = local write "Servo Goal Position\n - Left"(w2233) -> ()
          }
        }
        n782 = case shown="True" w2228 {
          tunnel: w2230 -> [_ w2232]
          frame False {
          }
          frame True {
            # "New Direction"
            # "Update Goal Position"
            # "Update Direction"
            n783 = local write "Servo Goal Position\n - Right"(w2232) -> ()
          }
        }
      }
      frame #1 {
        # "Allow Comm Process to Take Down the Flag\nOnly Raise if not already in motion"
        n784 = local read "Servo Moving - R"() -> (w2242:bool)
        n785 = local read "Servo Moving - L"() -> (w2239:bool)
        n786 = local read "Move Servo - L"() -> (w2238:bool)
        n787 = local read "Move Servo - R"() -> (w2245:bool)
        n788 = Not(x=w2242) -> (.not. x?=w2244:bool)
        n789 = Not(x=w2239) -> (.not. x?=w2241:bool)
        n790 = And(x=w2234, y=w2244) -> (x .and. y?=w2243:bool)
        n791 = And(x=w2237, y=w2241) -> (x .and. y?=w2240:bool)
        n792 = case shown="True" w2243 {
          selector: w2243 -> [_ w2247]
          tunnel: [w2246 w2247] -> w2235
          tunnel: w2245 -> [w2246 _]
          frame False {
          }
          frame True {
          }
        }
        n793 = case shown="False" w2240 {
          selector: w2240 -> [_ w2249]
          tunnel: [w2248 w2249] -> w2236
          tunnel: w2238 -> [w2248 _]
          frame False {
          }
          frame True {
          }
        }
        n794 = local write "Move Servo - R"(w2235) -> ()
        n795 = local write "Move Servo - L"(w2236) -> ()
      }
    }
    n796 = local read "Current Tracking State - Right 2"() -> (w1225:enum16{"Track", "Reactive Predict", ""})
    n797 = local read "Current Tracking State - Left"() -> (w1227:enum16{"Track", "Reactive Predict", ""})
    n798 = local read "Current Main State - Left"() -> (w1251:T5)
    n799 = local read "Current Main State - Right"() -> (w1226:T5)
    n800 = Equal?(x=w1226, y=w1250) -> (x = y?=w1220:bool)
    n801 = Equal?(x=w1225, y=w1224) -> (x = y?=w1219:bool)
    n802 = Equal?(x=w1251, y=w1250) -> (x = y?=w1222:bool)
    n803 = Equal?(x=w1227, y=w1224) -> (x = y?=w1223:bool)
    n804 = And(x=w1220, y=w1219) -> (x .and. y?=w1218:bool)
    n805 = And(x=w1222, y=w1223) -> (x .and. y?=w1221:bool)
    n806 = And(x=w1221, y=w1280) -> (x .and. y?=w1276:bool)
    n807 = And(x=w1281, y=w1218) -> (x .and. y?=w1277:bool)
    n808 = And(x=w1221, y=w1218) -> (x .and. y?=w1275:bool)
    n809 = Exclusive Or(1:w1277, 2:w1276) -> (0:w1274:bool)
    n810 = case shown="True" w1274 {
      tunnel: [w2260 w2281] -> w1282
      tunnel: [w2261 w2280] -> w1278
      tunnel: w1183 -> [_ w2284]
      tunnel: w1241 -> [w2258 w2285]
      tunnel: w1194 -> [w2256 w2283]
      tunnel: [w2259 w2271] -> w1279
      tunnel: [w2257 w2270] -> w1283
      tunnel: w1249 -> [_ w2282]
      tunnel: w1275 -> [w2255 _]
      tunnel: w1276 -> [_ w2281]
      tunnel: w1277 -> [_ w2280]
      frame False {
        n811 = case shown="False" w2255 {
          tunnel: [w2265 w2267] -> w2261
          tunnel: [w2264 w2267] -> w2260
          tunnel: [w2263 w2266] -> w2259
          tunnel: w2258 -> [w2263 _]
          tunnel: [w2262 w2266] -> w2257
          tunnel: w2256 -> [w2262 _]
          frame False {
            # "No Movement\nRetain All Values"
            n812 = local read "Move Respond - L"() -> (w2265:bool)
            n813 = local read "Move Respond - R"() -> (w2264:bool)
          }
          frame True {
            w2266 = i16 0
            w2267 = FALSE
            # "Reset Delta Move sum\nfor both"
            # "F"
            # "Both Moved,\nMake Flags False"
          }
        }
      }
      frame True {
        w2277 = 200 ("y")
        w2268 = -200 ("y")
        # "Add/Clear Sum for \nServo That didn't move"
        # "Update Moving Servo's  Delta Position"
        # "if one Servo Moves, other should \nmove too eventually,\nUsed in Search Process"
        # "Only 1 Servo is Moving Due to Tracking --> Update delta move sum"
        n814 = case shown="True" w2280 {
          tunnel: w2285 -> [_ w2293]
          tunnel: w2284 -> [_ w2292]
          tunnel: [i16 0 w2291] -> w2278
          frame False {
          }
          frame True {
            n815 = Add(x=w2293, y=w2292) -> (x+y=w2291:i32)
          }
        }
        n816 = case shown="True" w2281 {
          tunnel: w2283 -> [_ w2289]
          tunnel: w2282 -> [_ w2288]
          tunnel: [i16 0 w2287] -> w2275
          frame False {
          }
          frame True {
            n817 = Add(x=w2289, y=w2288) -> (x+y=w2287:i32)
          }
        }
        n818 = Greater?(x=w2278, y=w2277) -> (0:w2279:bool)
        n819 = Greater?(x=w2275, y=w2277) -> (0:w2276:bool)
        n820 = Select(t=w2277, s=w2276, f=w2275) -> (s? t:f=w2272:i32)
        n821 = Select(t=w2277, s=w2279, f=w2278) -> (s? t:f=w2273:i32)
        n822 = Greater?(x=w2273, y=w2268) -> (0:w2269:bool)
        n823 = Greater?(x=w2272, y=w2268) -> (0:w2274:bool)
        n824 = Select(t=w2272, s=w2274, f=w2268) -> (s? t:f=w2270:i32)
        n825 = Select(t=w2273, s=w2269, f=w2268) -> (s? t:f=w2271:i32)
      }
    }
    n826 = case shown="True" w1187 {
      selector: w1187 -> [_ w2227]
      tunnel: [w2224 w2226] -> w1236
      tunnel: [w2223 i16 0] -> w1237
      tunnel: w1282 -> [w2224 _]
      tunnel: w1283 -> [w2223 _]
      frame False {
      }
      frame True {
        n827 = Not(x=w2227) -> (.not. x?=w2226:bool)
      }
    }
    "Move Respond - R" <- w1236
    "deltaMoveServo\n- R" <- w1237
    n828 = case shown="False" w1247 {
      selector: w1247 -> [_ w2254]
      tunnel: [w2251 w2253] -> w1239
      tunnel: [w2250 i16 0] -> w1242
      tunnel: w1278 -> [w2251 _]
      tunnel: w1279 -> [w2250 _]
      frame False {
      }
      frame True {
        n829 = Not(x=w2254) -> (.not. x?=w2253:bool)
      }
    }
    "Move Respond - L" <- w1239
    "deltaMoveServo\n- L" <- w1242
    "Current Main State - Left" <- w1270
    "Frames Processed\nCount - in -L" <- w1262
    "Recovery Mode Count - in Left" <- w1257
    "Recovery Search\nmove Count - in - L" <- w1256
    "Recovery Search\nAttempt Count - in - L" <- w1255
    "Current Main State - Right" <- w1217
    "Frames Processed\nCount - in Right" <- w1200
    "Recovery Search\nmove Count - Right" <- w1202
    "Recovery Search\nAttempt Count - Right" <- w1201
    "Recovery Mode Count in Right" <- w1193
    "Tracking Timeout\nCount - L" <- w1234
    "Tracking Timeout\nCount - R" <- w1209
    "Current Tracking State - Left" <- w1233
    "Current Tracking State - Right 2" <- w1215
    "Current Recovery State - Right" <- w1216
    "Current Recovery State -L" <- w1230
  }
